vi "Gas Rack MAIN (PC).vi"() -> ()   [LabVIEW 2013]
uses:
  TypeDef/Controller Names.ctl
  TypeDef/StandConfigCluster.ctl
  TypeDef/DataCluster.ctl
  RT subVIs/Controls/TraceCluster.ctl
  TypeDef/Command Cluster.ctl
  TypeDef/TestCfgCluster.ctl
  TCP/PC/Event Mode.ctl
  TypeDef/Stability Cluster.ctl
  <vilib>/Utility/miscctls.llb/LVRowAndColumnTypeDef.ctl
  <vilib>/Utility/miscctls.llb/LVRowAndColumnUnsignedTypeDef.ctl
  TypeDef/Parameter Controls Mode.ctl
  TCP/PC/PCsend RTrecv CMD.ctl
  <vilib>/Utility/miscctls.llb/LVPositionTypeDef.ctl
  TypeDef/ConnSettingCluster.ctl
  <vilib>/Utility/config.llb/Write Key (String).vi
  <vilib>/Utility/file.llb/Write To Spreadsheet File (string).vi
  <vilib>/Utility/config.llb/NI_LVConfig.lvlib
panel:
  in  "Screen Control":enum32{"Page 1"}(tab)
  in  "pb.RunScreen":bool
  in  "pb.TestConfig":bool
  in  "pb.StandConfig":bool
  in  "Screen":T1(tab)=enum."Test Configuration Page"
  in  "FFTwindowMin":u16=300
  in  "FFTwindowMax":u16=1400 caption="Max"
  in  "Steps":u16(ring) items=["Manual", "1)   V=12, P=500, C=50", "2)   V=12, P=450, C=50", "3)   V=12, P=400, C=50"]
  out "Efficiency (%)":dbl format="%.1f"
  out "Controller CMD":dbl format="%#.1f"
  in  "Parameter 3":T2(ring)=enum."Command"
  in  "Setpoint3":dbl=10.0 caption="Setpoint 3" min=10.0 max=90.0 step=0.1
  out "Running?":bool
  in  "Serial Number":string
  out "Speed (RPM)":dbl format="%#.0f"
  out "PumpCurrent(Arms)":dbl caption="Pump Current\n(A RMS)" format="%.2f"
  out "CtrlrCurrent(A)":dbl caption="Controller\nCurrent (A)" format="%.2f"
  out "Fuel Temp (C)":dbl format="%.1f"
  out "Flow (L/H)":dbl format="%.1f"
  out "Pressure (kPa)":dbl format="%.1f"
  in  "Setpoint2":dbl caption="Setpoint 2" min=-1.0 max=800.0
  in  "Setpoint1":dbl caption="Setpoint 1" min=-1.0 max=18.0
  out "RS File Location":string caption="File Location"
  in  "pb.StartTest":bool
  out "Voltage (DC)":dbl caption="Controller\nVoltage (V)" format="%.2f"
  out "Stabilized?":bool
  in  "Tables":enum32{"Data", "Stats", "Notes"}(tab)
  in  "table.Data":string[][](table)
  in  "table.Stats":string[][](table)
  in  "Notes":string
  in  "Parameter 1":T3(ring)
  in  "Parameter 2":enum16{"Voltage", "Pressure", "Flow", "Speed"}(ring)=enum."Pressure"
  in  "Tab.Buttons":enum32{"Manual", "Test"}(tab)
  in  "pb.StartManual":bool
  in  "pb.GrabData":bool
  in  "pb.Pause Test":bool
  in  "pb.Skip Step":bool
  in  "pb.ClearProfile":bool
  in  "pb.load profile":bool
  in  "TestType":enum32{"Flow", "Test", "Hot\nFuel"}(radio)
  in  "File Location":string
  in  "Platform":string
  in  "Customer":string
  in  "Pump Control Style":T4
  in  "pb.load":bool
  in  "pb.save":bool
  in  "pb.new":bool
  in  "Pump Model":string
  in  "Durability Tank Number":string
  in  "Fuel Batch Number":string
  in  "Flow Test Fluid":string
  in  "Durability Fluid":string
  in  "Hours Completed":string
  in  "Shop Order Number":string
  in  "CA Number":string
  in  "Technician Name":string
  in  "Pump# Pages":enum32{"SN", "Auto"}(tab)
  in  "Serial Numbers":string[][](table)
  in  "pb.auto-pop":bool
  in  "pb.auto-confirm":bool
  in  "pb.auto-cancel":bool
  in  "Ending Serial Number":u32
  in  "Serial Number Step":u32
  in  "Starting Serial Number":u32
  in  "Parameters":string[][](table) caption="Parameter Setup"
  out "Hardware Style":string
  in  "Pressure Control":bool
  out "Max Command":dbl
  out "Min Command":dbl
  in  "Gauge Number":string
  out "Calibration Due Date":string
  in  "Speed Tolerance":dbl
  in  "Max Pressure":dbl
  in  "IP Address":string
  in  "Max Voltage":dbl
  in  "Free Flow Pressure":dbl
  in  "Free Flow Voltage":dbl
  in  "Init Free Flow (sec)":dbl
  in  "Max Current":dbl
  in  "Stable Count (sec)":dbl=1.0 min=1.0
  in  "Flow Tolerance":dbl
  in  "Voltage Tolerance":dbl
  in  "Pressure Tolerance":dbl
  in  "Parameter Timeout (sec)":dbl=3.0 min=6.0
  in  "Max Flow":dbl
  in  "Min Flow":dbl
  in  "pb.RetryRIO":bool
  in  "IP Address 2":string caption="IP Address"
  out "Tested Serial Numbers":string[][](table)
  out "Untested Serial Numbers":string[][](table)
  in  "pb.test cancel":bool
  in  "Next Serial Number":string
  in  "pb.select SN":bool
  out "InvalidResponses":string
  out "Error Out":errorcluster
  out "unreachable":bool
  in  "FlattenedData":string
  in  "Command":string
  in  "Connected?":bool
  in  "Connected? 2":bool
  in  "Panel Close?":bool
  out "StoredDataRow":i32
  in  "DataDisplayRefs":refnum<vi>[](array[refnum])
  # "Run Screen"
  # "Test Configuration Page"
  # "Stand Configuration Page"
  # "RIO Connection Page"
  # "Error occured with connection to RIO.\nCheck connections."
  # "Part Change Page"
  # "never implemented"
  # "Para 1 (0-4) [Voltage Pressure Flow Speed Deadhead]\nPara 2 (0-3) [Voltage Pressure Flow Speed]\nPara 3 (0-4) [Voltage Pressure Flow Speed Command]"
  # "New Features:"
  # "* Dynamically controls brushless pumps to meet parameters *"
  # "* Statistics include manually taken data points *"
  # "* Statistics updated with every data point taken *"
  # "* RPM is fully handled, no more user input for FFT windowing *"
  # "_______________________________________________________________________________________________________________________________________________________"
  # "* Calibration standardized *"
  # "* Voltage/current selectable at pump/controller *"
  # "_________________________________________________________________________________________________________________________________"
  # "* Added free flow on startup for brushless pumps *"
  # "Calibration due\nfor verification."
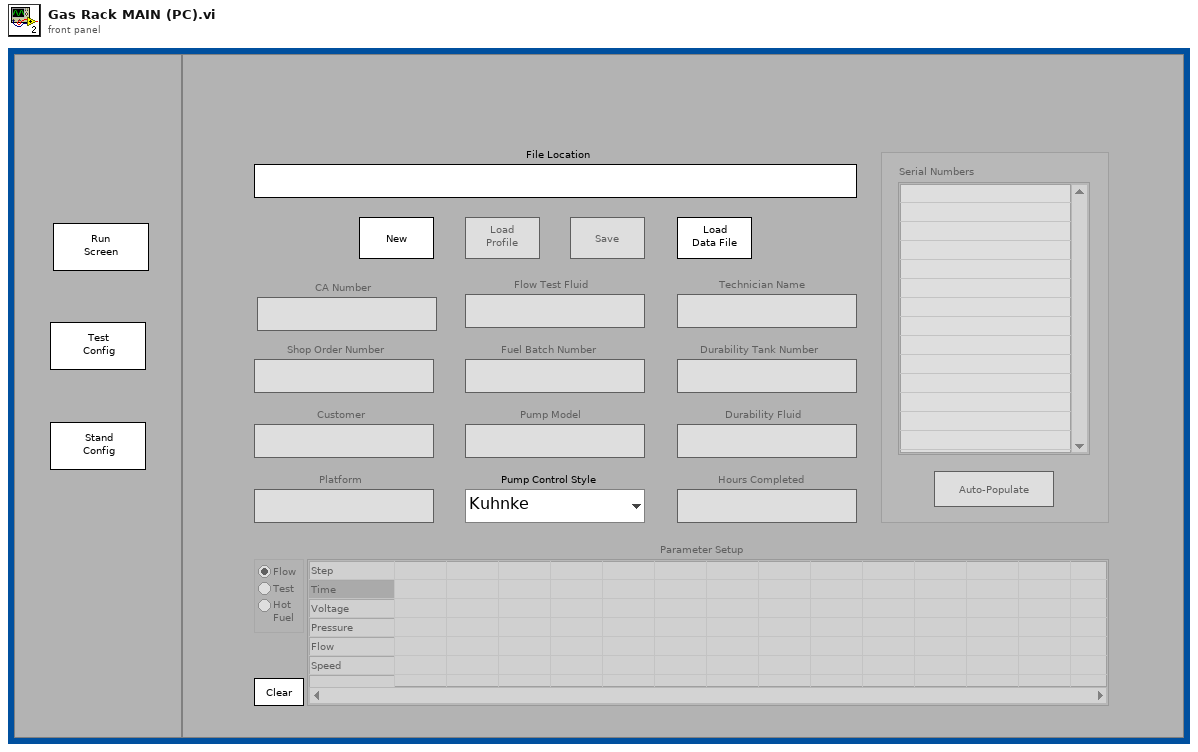
[diagram p1: front panel]
types:
  T1 = enum32{"Run Screen", "Test Configuration Page", "Stand Configuration Page", "RIO Connection", "Part Change", "Spare Front Panel Items", "Intro", "Cal Warning"}
  T2 = enum16{"Voltage", "Pressure", "Flow", "Speed", "Command"}
  T3 = enum16{"Voltage", "Pressure", "Flow", "Speed", "Deadhead"}
  T4 = typedef "Controller Names.ctl" = enum16{"Kuhnke", "McLaren", "Helbako BLDC", "Conti", "Hella E4LMF", "Hella E4LMD", "Hella E4DCG 20mm", "Hella E4DCG 30mm", "Helbako (old)", "TI PWM", "PSA", "Hella Hyundai Gas", "Hella Hyundai Diesel", "8 Comm", "10 Comm", "8 Comm Hella FCA", "10 Comm Hella FCA", "8 Comm Omron", "10 Comm Omron", "8 Comm Nissan", "10 Comm Nissan"}
  T5 = typedef "Stability Cluster.ctl" = cluster{"Voltage Tolerances":dbl, "Pressure Tolerances":dbl, "Flow Tolerances":dbl, "Speed Tolerances":dbl, "Stable Count (sec)":dbl}
  T6 = typedef "Command Cluster.ctl" = cluster{"Para1":i32, "SP1":dbl, "Para2":i32, "SP2":dbl, "Para3":i32, "SP3":dbl}
  T7 = cluster{"ParameterSet":string, "Data":string[][], "Step":i32, "EarliestDate":string, "Stats":string[][]}[]
  T8 = typedef "Event Mode.ctl" = enum16{"Init", "Get", "Set", "Destroy"}
  T9 = cluster{"Controller Name":T4, "CommSeg":i32, "PWM?":bool, "Frequency":i32, "Low Command":dbl, "High Command":dbl, "Stop Command":dbl, "Command Step":dbl, "Solenoid Stop?":bool, "Controller?":bool, "Name":string, "Indirect Nonzero CMD":dbl}[]
  T10 = cluster{"Controller Name":T4, "CommSeg":i32, "PWM?":bool, "Frequency":i32, "Low Command":dbl, "High Command":dbl, "Stop Command":dbl, "Command Step":dbl, "Solenoid Stop?":bool, "Controller?":bool, "Name":string, "Indirect Nonzero CMD":dbl}
  T11 = typedef "TestCfgCluster.ctl" = cluster{"Technician Name":string, "Shop Order Number":string, "Customer":string, "Platform":string, "Flow Test Fluid":string, "Fuel Batch #":string, "CA Number":string, "Durability Tank #":string, "Durability Fluid":string, "Hours Completed":string, "Pump Model":string, "Pump Control Style":T4}
  T12 = typedef "TraceCluster.ctl" = cluster{"PreTriggerPts":i32, "TotalPts":i32, "TriggerLvl":dbl, "PlotStyle":enum16{"Single - Rising Edge", "Single - Falling Edge", "Continuous", "Repeat - Rising Edge", "Repeat - Falling Edge"}, "TriggerChannel":i32, "TraceCtrl":bool}
  T13 = typedef "DataCluster.ctl" = cluster{"Pump Voltage (V)":dbl, "Pump Current (Arms)":dbl, "Pressure (kPA)":dbl, "Flow (L/H)":dbl, "Controller Voltage (V)":dbl, "Controller Current (A)":dbl, "Fuel Temp (C)":dbl, "Speed (RPM)":dbl, "Efficiency (%)":dbl, "Stabilized?":bool, "Controller CMD":dbl}
  T14 = typedef "StandConfigCluster.ctl" = cluster{"Max Voltage":dbl, "Voltage Tolerance":dbl, "Max Current":dbl, "Max Pressure":dbl, "Pressure Tolerance":dbl, "Min Flow":dbl, "Max Flow":dbl, "Flow Tolerance":dbl, "Speed Tolerance":dbl, "Stable Count":dbl, "Parameter Timeout":dbl, "Init Free Flow":dbl, "Free Flow Voltage":dbl, "Free Flow Pressure":dbl}
  T15 = cluster{"TestCfgCluster":T11, "Serial Numbers":string[], "StandConfigCluster":T14, "Serial Number":string, "table.Data":string[][], "table.Stats":string[][], "CommandCluster":T6, "DataCluster":T13, "RIOTries":i32, "TestRunning?":bool, "StepIndex":i32, "CurrentDataFile":path, "DefaultDataPath":path, "PreviousDataFile":path, "Untested SNs":string[], "Tested SNs":string[], "RIOconnection":bool, "StepTimeLimit":dbl, "WaitingData":bool, "Controller":cluster{"Controller Name":T4, "CommSeg":i32, "PWM?":bool, "Frequency":i32, "Low Command":dbl, "High Command":dbl, "Stop Command":dbl, "Command Step":dbl, "Solenoid Stop?":bool, "Controller?":bool, "Name":string, "Indirect Nonzero CMD":dbl}, "TraceCluster":T12, "IP Address":string, "TemplatePath":path, "Notes":string, "LastDataSet":string[], "ValidFile?":bool, "LastDataRow":i32, "LastStatRow":i32, "Gauge Number":string, "Calibration Due Date":string, "Free Flow":bool, "StepDataActive":dbl, "Parameters":string[][], "KF.Parameters":bool, "Flow?":bool, "ColInsert":bool, "SkipStep":bool, "KeepManualPts":bool, "Created/ModFiles":cluster{"FilePath":path, "Save?":bool}[], "Controller List":cluster{"Controller Name":T4, "CommSeg":i32, "PWM?":bool, "Frequency":i32, "Low Command":dbl, "High Command":dbl, "Stop Command":dbl, "Command Step":dbl, "Solenoid Stop?":bool, "Controller?":bool, "Name":string, "Indirect Nonzero CMD":dbl}[], "ProfilePath":path, "LastFileState":enum16{"New File", "Load File", "Neither"}, "NotLoadProfile":bool, "LastDataTime":i64, "ValidPara?":bool, "StatBundle":cluster{"ParameterSet":string, "Data":string[][], "Step":i32, "EarliestDate":string, "Stats":string[][]}[], "DesiredParameters":T6, "Stability Cluster":T5, "DataDisplayRefs":refnum<vi>[], "ExpectedFPGA":i32}
  T16 = typedef "LVRowAndColumnUnsignedTypeDef.ctl" = cluster{"Row":u32, "Column":u32}
  T17 = enum8{"Enabled", "Disabled", "Disabled and Grayed Out"}
  T18 = typedef "Parameter Controls Mode.ctl" = enum16{"Init", "Update Ranges", "Set Controls"}
  T19 = typedef "LVRowAndColumnTypeDef.ctl" = cluster{"Row":i32, "Column":i32}
  T20 = enum32{"invalid app kind", "Development System", "Run Time System", "Student Edition", "Embedded LabVIEW", "Evaluation", "Custom"}
  T21 = enum16{"Init", "Run Screen", "Test Config", "Stand Config", "Lock All", "Other Tab"}
  T22 = cluster{"Command":string, "FlattenedData":string}
  T23 = typedef "PCsend RTrecv CMD.ctl" = enum16{"ConnSettings", "Connect", "CMD", "Controller", "PSenable", "ReqCalDate", "Tolerances", "Stable Trigger", "Stop", "VPLimits", "NeedleValve", "SpeedWindow", "FreezeCmdPID", "LoadFPGA"}
  T24 = cluster{"CurrentDataFile":path, "StandConfigCluster":T14, "IP Address":string, "DefaultDataPath":path, "Gauge Number":string, "ExpectedFPGA":i32}
  T25 = typedef "RTsend PCrecv CMD.ctl" = enum16{"Data", "Connected?", "CalFileDate"}
  T26 = enum16{"Voltage", "Pressure", "Flow", "Speed", "Deadhead"}[]
  T27 = typedef "NI_LVConfig.lvlib/Config Data RefNum.ctl" = refnum<k1>
  T28 = typedef "eventvkey.ctl" = enum16{"ASCII", "Enter", "Return", "Shift", "Ctrl", "Alt", "Cmd", "Opt", "Caps", "NumLock", "Clear", "Break", "Up", "Down", "Left", "Right", "Insert", "Delete", "Home", "End", "PageUp", "PageDown", "Escape", "Help", "Pause", "ScrollLock", "F1", "F2", "F3", "F4", "F5", "F6", "F7", "F8", "F9", "F10", "F11", "F12", "F13", "F14", "F15", "F16", "F17", "F18", "F19", "F20", "F21", "F22", "F23", "F24", "Play", "VolumeUp", "VolumeDown", "Mute", "Two Byte Char"}
  T29 = enum16{"Left Button", "Center Button", "Right Button", "Window Close"}
  T30 = typedef "LVPositionTypeDef.ctl" = cluster{"Left":i32, "Top":i32}
  T31 = cluster{"CommandCluster":T6, "DesiredParameters":T6}
  T32 = cluster{"data string":string, "data string":string}
  T33 = typedef "ConnSettingCluster.ctl" = cluster{"ConnectAttemptLimit(5)":u32, "IP Address":string, "Send Port":u16, "Recv Port":u16}
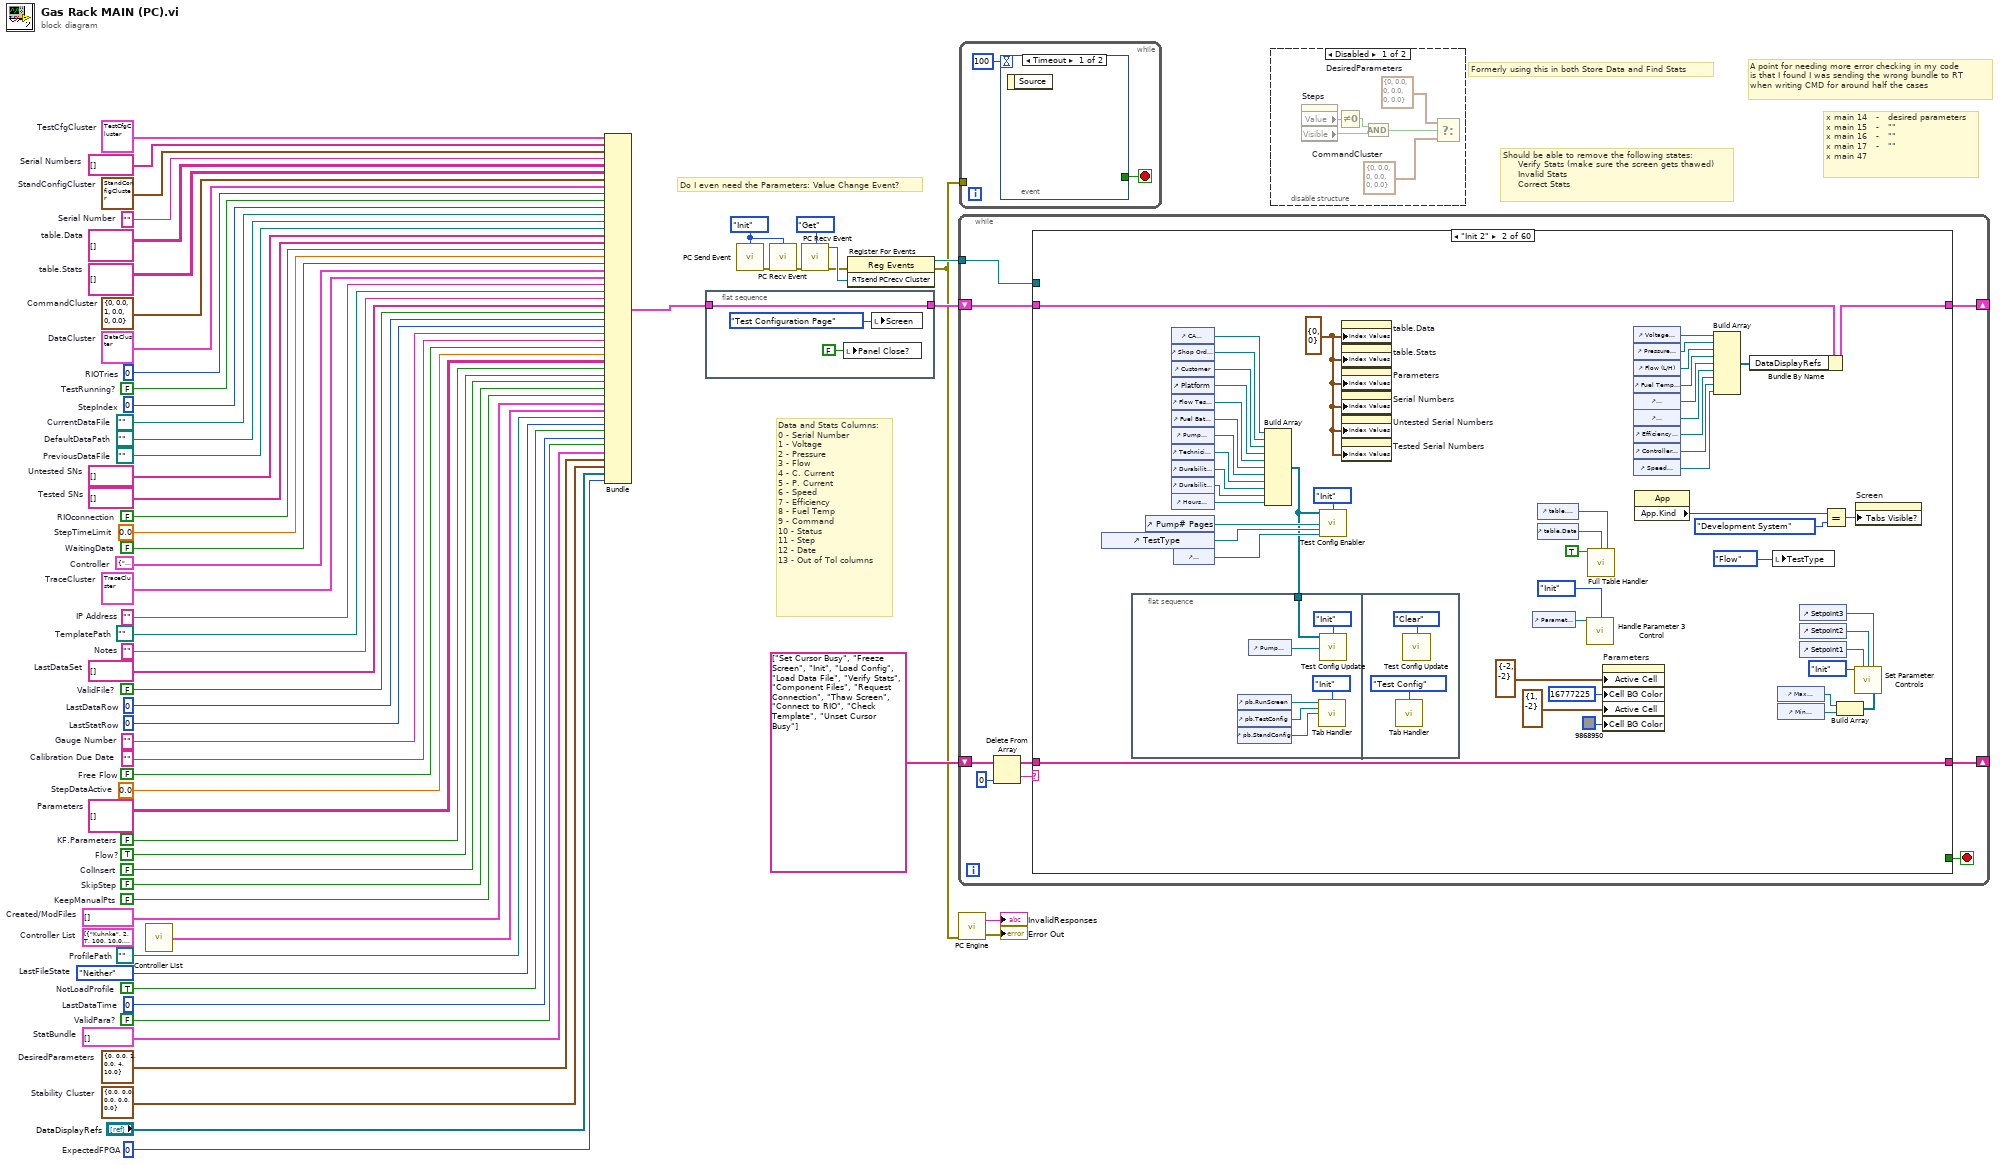
[diagram p0: block diagram]
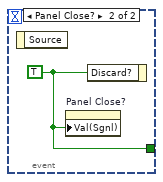
[diagram p3: hidden frame]
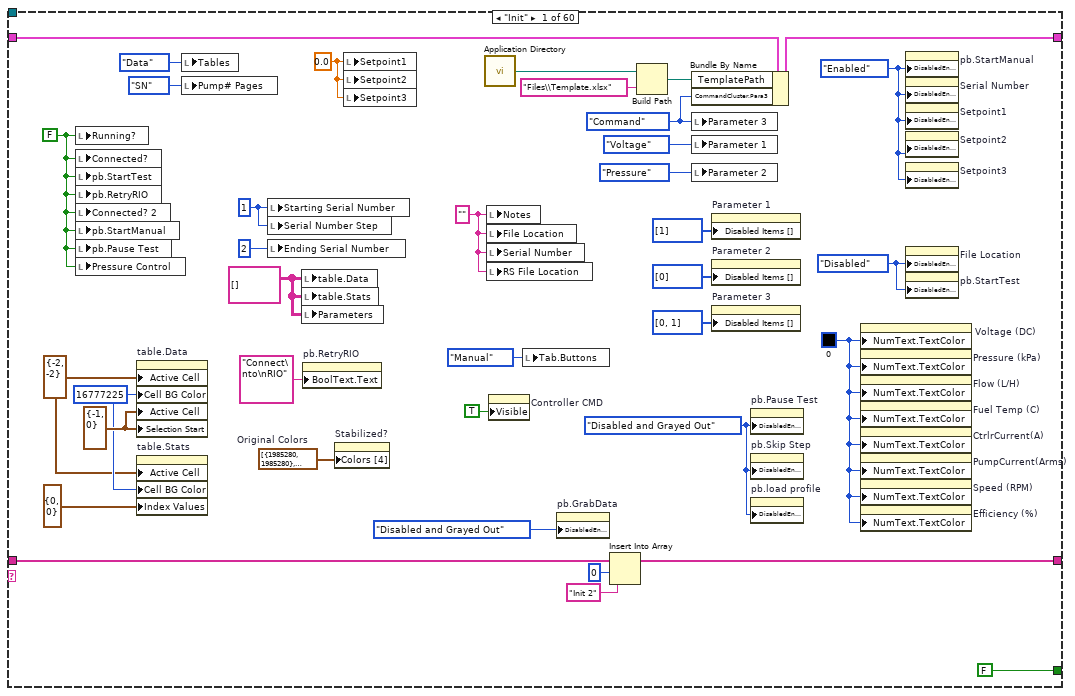
[diagram p4: hidden frame]
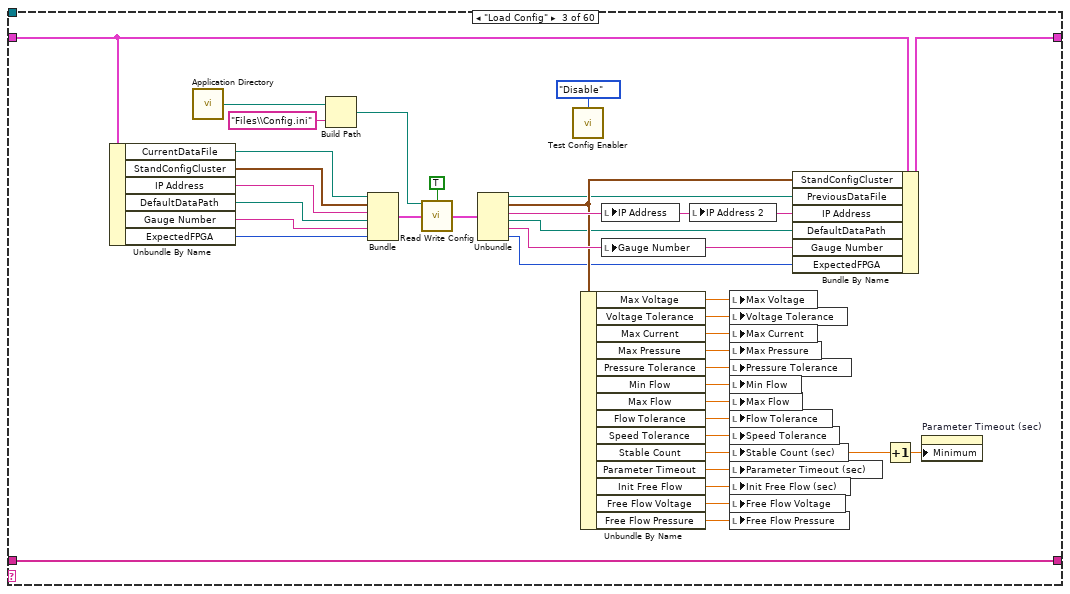
[diagram p5: hidden frame]
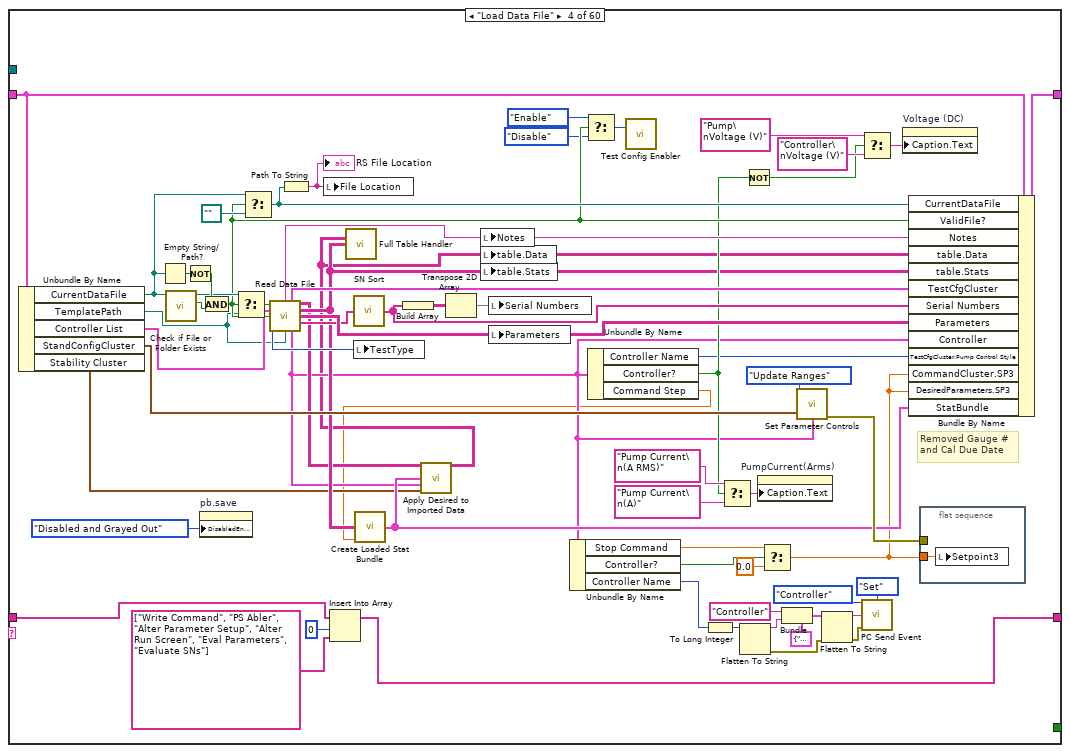
[diagram p6: hidden frame]
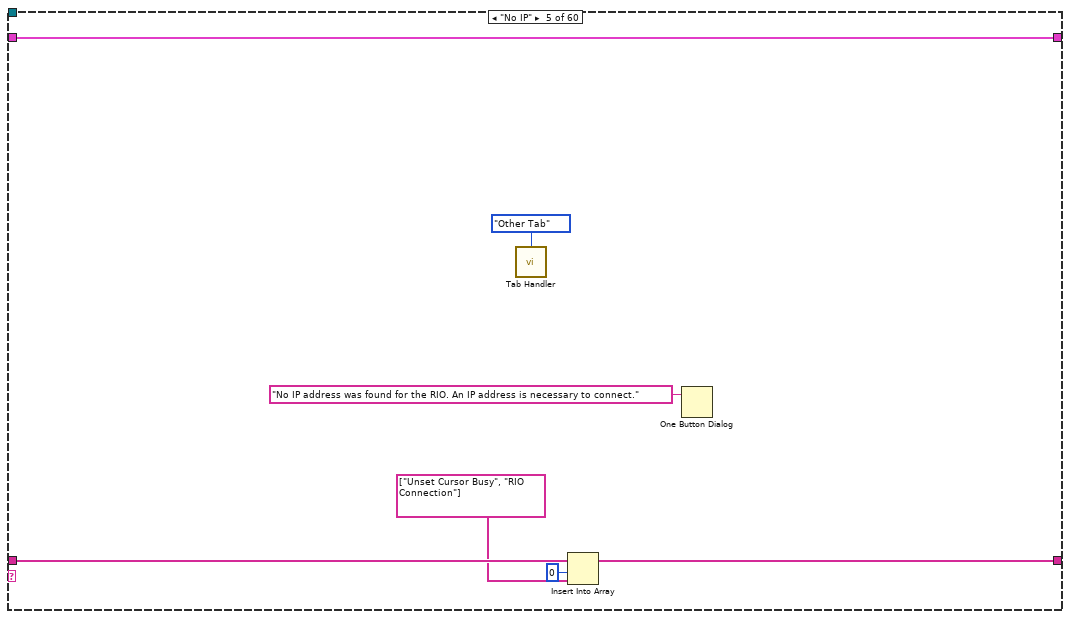
[diagram p7: hidden frame]
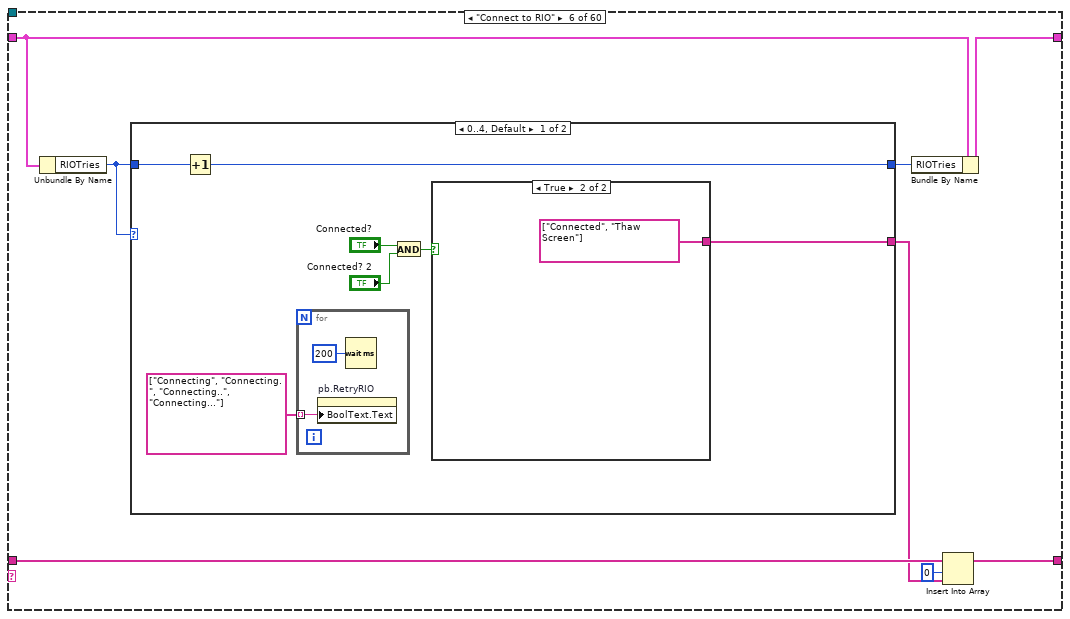
[diagram p8: hidden frame]
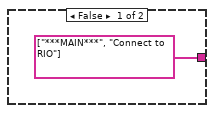
[diagram p9: hidden frame]
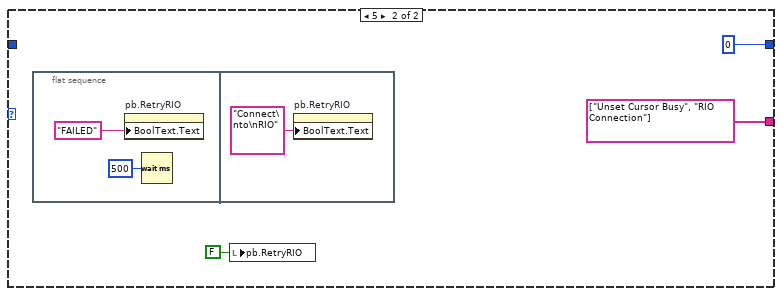
[diagram p10: hidden frame]
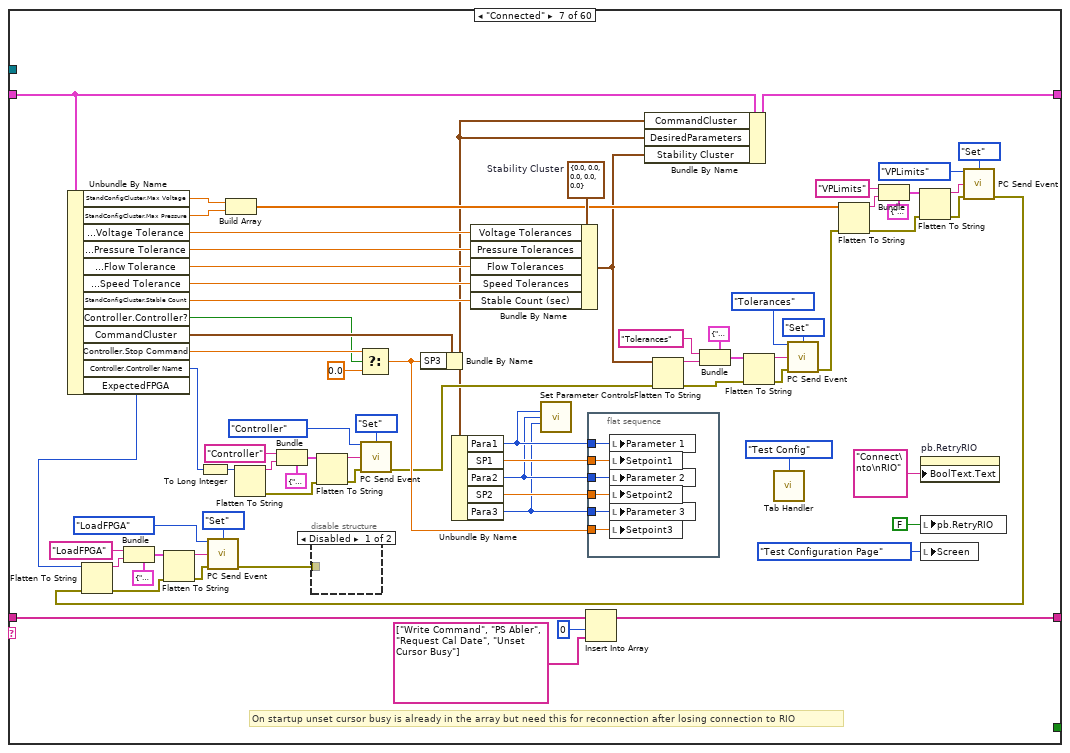
[diagram p11: hidden frame]
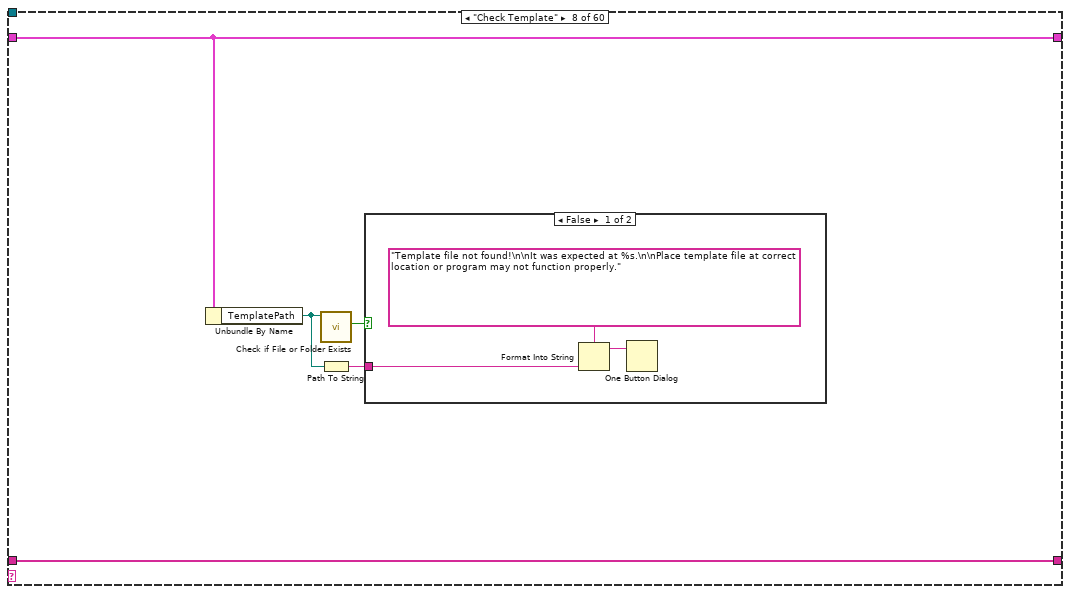
[diagram p13: hidden frame]
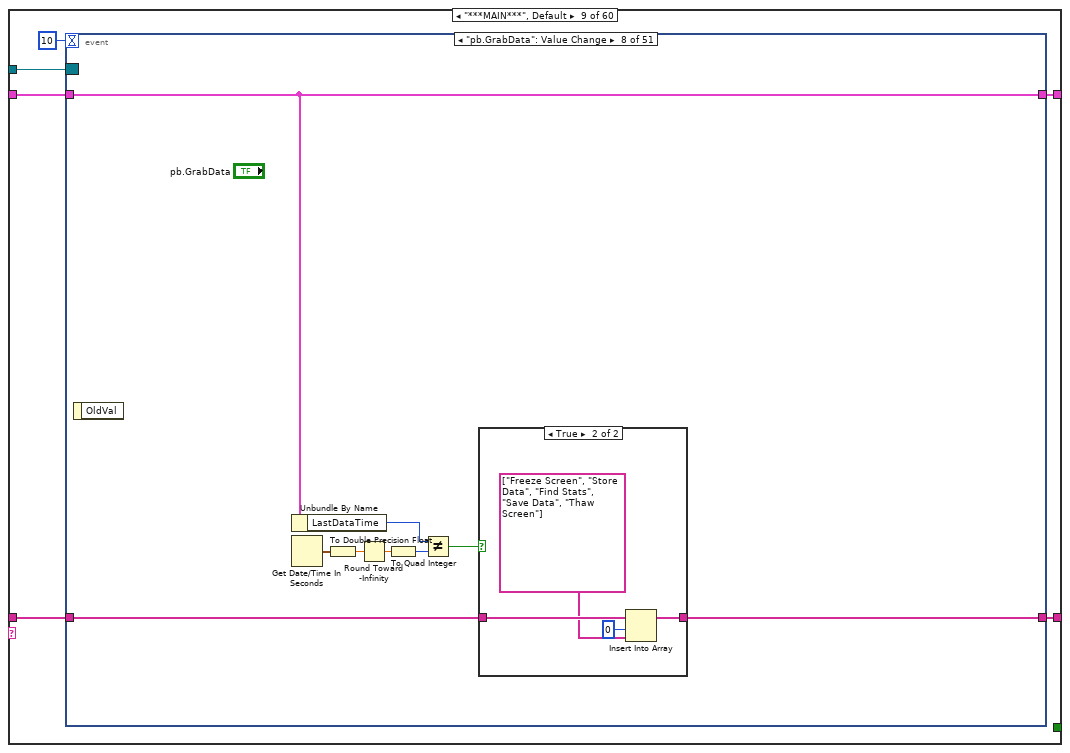
[diagram p15: hidden frame]
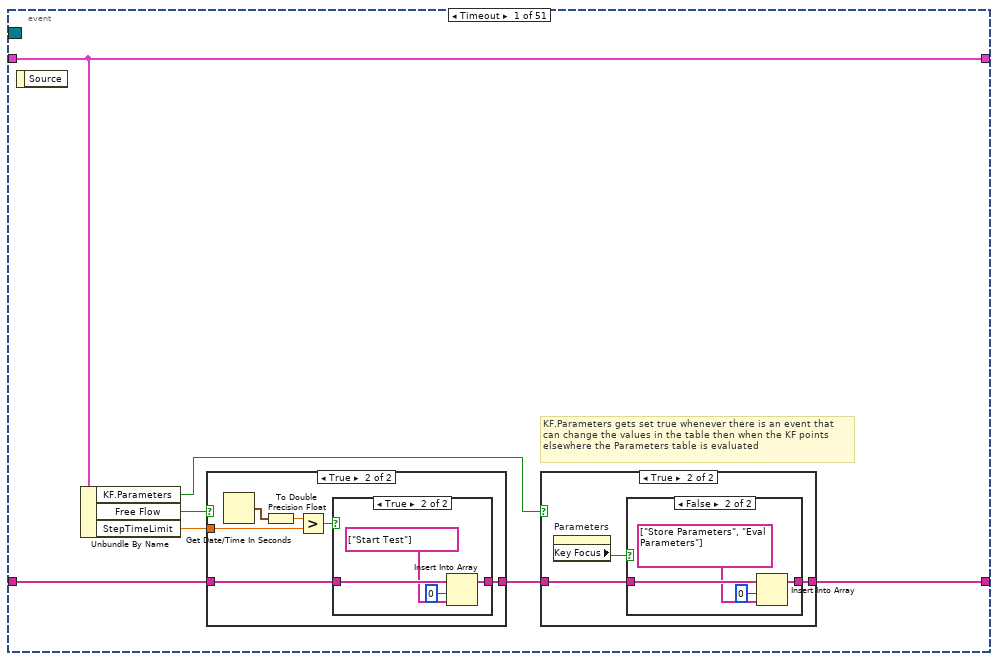
[diagram p16: hidden frame]
diagram:
  w1 = 0  # ExpectedFPGA
  w3 = T5 {"Voltage Tolerances"=0.0, "Pressure Tolerances"=0.0, "Flow Tolerances"=0.0, "Speed Tolerances"=0.0, "Stable Count (sec)"=0.0}  # Stability Cluster
  w4 = T6 {"Para1"=0, "SP1"=0.0, "Para2"=1, "SP2"=0.0, "Para3"=4, "SP3"=10.0}  # DesiredParameters
  w5 = T7 []  # StatBundle
  w6 = FALSE  # ValidPara?
  w7 = i64 0  # LastDataTime
  w15 = Event_Mode."Init" ("Mode")
  w21 = TRUE  # NotLoadProfile
  w22 = enum16{"New File", "Load File", "Neither"}."Neither"  # LastFileState
  w24 = path ""  # ProfilePath
  (unwired) T9 [{"Controller Name"=enum."Kuhnke", "CommSeg"=2, "PWM?"=TRUE, "Frequency"=100, "Low Command"=10.0, "High Command"=90.0, "Stop Command"=10.0, "Command Step"=0.1, "Solenoid Stop?"=FALSE, "Controller?"=TRUE, "Name"="Kuhnke", "Indirect Nonzero CMD"=15.0}, {"Controller Name"=enum."Helbako BLDC", "CommSeg"=2, "PWM?"=TRUE, "Frequency"=100, "Low Command"=10.0, "High Command"=90.0, "Stop Command"=10.0, "Command Step"=0.1, "Solenoid Stop?"=FALSE, "Controller?"=TRUE, "Name"="Helbako BLDC", "Indirect Nonzero CMD"=15.0}, {"Controller Name"=enum."Conti", "CommSeg"=2, "PWM?"=FALSE, "Frequency"=100, "Low Command"=0.0, "High Command"=800.0, "Stop Command"=0.0, "Command Step"=1.0, "Solenoid Stop?"=FALSE, "Controller?"=TRUE, "Name"="Conti", "Indirect Nonzero CMD"=0.0}, {"Controller Name"=enum."Hella E4LMF", "CommSeg"=2, "PWM?"=FALSE, "Frequency"=100, "Low Command"=0.0, "High Command"=100.0, "Stop Command"=0.0, "Command Step"=1.0, "Solenoid Stop?"=FALSE, "Controller?"=TRUE, "Name"="Hella BLDC Screw", "Indirect Nonzero CMD"=10.0}, {"Controller Name"=enum."Helbako (old)", "CommSeg"=2, "PWM?"=FALSE, "Frequency"=100, "Low Command"=0.0, "High Command"=100.0, "Stop Command"=0.0, "Command Step"=1.0, "Solenoid Stop?"=FALSE, "Controller?"=TRUE, "Name"="Hella BLDC Turbine", "Indirect Nonzero CMD"=10.0}, {"Controller Name"=enum."Helbako (old)", "CommSeg"=2, "PWM?"=FALSE, "Frequency"=100, "Low Command"=0.0, "High Command"=100.0, "Stop Command"=0.0, "Command Step"=0.1, "Solenoid Stop?"=FALSE, "Controller?"=TRUE, "Name"="Helbako (old)", "Indirect Nonzero CMD"=0.0}, {"Controller Name"=enum."TI PWM", "CommSeg"=2, "PWM?"=TRUE, "Frequency"=100, "Low Command"=0.0, "High Command"=100.0, "Stop Command"=0.0, "Command Step"=0.1, "Solenoid Stop?"=FALSE, "Controller?"=TRUE, "Name"="TI PWM", "Indirect Nonzero CMD"=0.0}, {"Controller Name"=enum."PSA", "CommSeg"=2, "PWM?"=TRUE, "Frequency"=100, "Low Command"=5.0, "High Command"=95.0, "Stop Command"=5.0, "Command Step"=0.1, "Solenoid Stop?"=FALSE, "Controller?"=TRUE, "Name"="PSA", "Indirect Nonzero CMD"=5.0}, {"Controller Name"=enum."Hella Hyundai Diesel", "CommSeg"=2, "PWM?"=FALSE, "Frequency"=100, "Low Command"=0.0, "High Command"=800.0, "Stop Command"=0.0, "Command Step"=1.0, "Solenoid Stop?"=TRUE, "Controller?"=TRUE, "Name"="Hella Gas", "Indirect Nonzero CMD"=0.0}, {"Controller Name"=enum."8 Comm", "CommSeg"=10, "PWM?"=FALSE, "Frequency"=100, "Low Command"=370.0, "High Command"=461.0, "Stop Command"=370.0, "Command Step"=1.0, "Solenoid Stop?"=TRUE, "Controller?"=TRUE, "Name"="Hella Diesel", "Indirect Nonzero CMD"=370.0}, {"Controller Name"=enum."8 Comm", "CommSeg"=8, "PWM?"=FALSE, "Frequency"=150, "Low Command"=0.0, "High Command"=1.0, "Stop Command"=0.0, "Command Step"=1.0, "Solenoid Stop?"=FALSE, "Controller?"=FALSE, "Name"="8 Comm", "Indirect Nonzero CMD"=0.0}, {"Controller Name"=enum."10 Comm", "CommSeg"=10, "PWM?"=FALSE, "Frequency"=150, "Low Command"=0.0, "High Command"=1.0, "Stop Command"=0.0, "Command Step"=1.0, "Solenoid Stop?"=FALSE, "Controller?"=FALSE, "Name"="10 Comm", "Indirect Nonzero CMD"=0.0}, {"Controller Name"=enum."10 Comm Hella FCA", "CommSeg"=8, "PWM?"=TRUE, "Frequency"=150, "Low Command"=0.0, "High Command"=50.0, "Stop Command"=80.0, "Command Step"=0.1, "Solenoid Stop?"=FALSE, "Controller?"=TRUE, "Name"="8 Comm Hella", "Indirect Nonzero CMD"=0.0}, {"Controller Name"=enum."8 Comm Omron", "CommSeg"=10, "PWM?"=TRUE, "Frequency"=150, "Low Command"=0.0, "High Command"=50.0, "Stop Command"=80.0, "Command Step"=0.1, "Solenoid Stop?"=FALSE, "Controller?"=TRUE, "Name"="10 Comm Hella", "Indirect Nonzero CMD"=0.0}, {"Controller Name"=enum."8 Comm Omron", "CommSeg"=8, "PWM?"=TRUE, "Frequency"=150, "Low Command"=5.0, "High Command"=50.0, "Stop Command"=75.0, "Command Step"=0.1, "Solenoid Stop?"=FALSE, "Controller?"=TRUE, "Name"="8 Comm Omron", "Indirect Nonzero CMD"=5.0}, {"Controller Name"=enum."10 Comm Omron", "CommSeg"=10, "PWM?"=TRUE, "Frequency"=150, "Low Command"=5.0, "High Command"=50.0, "Stop Command"=75.0, "Command Step"=0.1, "Solenoid Stop?"=FALSE, "Controller?"=TRUE, "Name"="10 Comm Omron", "Indirect Nonzero CMD"=5.0}, {"Controller Name"=enum."8 Comm Nissan", "CommSeg"=8, "PWM?"=TRUE, "Frequency"=10, "Low Command"=50.0, "High Command"=90.0, "Stop Command"=50.0, "Command Step"=0.1, "Solenoid Stop?"=TRUE, "Controller?"=TRUE, "Name"="8 Comm Nissan", "Indirect Nonzero CMD"=50.0}, {"Controller Name"=enum."10 Comm Nissan", "CommSeg"=10, "PWM?"=TRUE, "Frequency"=10, "Low Command"=50.0, "High Command"=90.0, "Stop Command"=50.0, "Command Step"=0.1, "Solenoid Stop?"=TRUE, "Controller?"=TRUE, "Name"="10 Comm Nissan", "Indirect Nonzero CMD"=50.0}]  # Controller List
  w25 = T10 {"Controller Name"=enum."Kuhnke", "CommSeg"=2, "PWM?"=TRUE, "Frequency"=100, "Low Command"=10.0, "High Command"=90.0, "Stop Command"=10.0, "Command Step"=0.1, "Solenoid Stop?"=FALSE, "Controller?"=TRUE, "Name"="Kuhnke", "Indirect Nonzero CMD"=15.0}  # Controller
  w50 = T11 {"Technician Name"="", "Shop Order Number"="", "Customer"="", "Platform"="", "Flow Test Fluid"="", "Fuel Batch #"="", "CA Number"="", "Durability Tank #"="", "Durability Fluid"="", "Hours Completed"="", "Pump Model"="", "Pump Control Style"=enum."Kuhnke"}  # TestCfgCluster
  w41 = T6 {"Para1"=0, "SP1"=0.0, "Para2"=1, "SP2"=0.0, "Para3"=0, "SP3"=0.0}  # CommandCluster
  w52 = T12 {"PreTriggerPts"=0, "TotalPts"=10, "TriggerLvl"=0.0, "PlotStyle"=enum."Single - Falling Edge", "TriggerChannel"=2, "TraceCtrl"=FALSE}  # TraceCluster
  w26 = cluster{"FilePath":path, "Save?":bool}[] []  # Created/ModFiles
  w27 = string[][] []  # table.Stats
  w28 = string[][] []  # table.Data
  w29 = FALSE  # KeepManualPts
  w30 = FALSE  # SkipStep
  w31 = FALSE  # ColInsert
  w32 = TRUE  # Flow?
  w33 = FALSE  # KF.Parameters
  w34 = string[][] []  # Parameters
  w35 = 0.0  # StepDataActive
  w36 = FALSE  # Free Flow
  w37 = ""  # Calibration Due Date
  w38 = ""  # Gauge Number
  w39 = path ""  # PreviousDataFile
  w40 = string[] []  # Tested SNs
  w42 = 0  # LastStatRow
  w43 = 0  # LastDataRow
  w44 = string[] []  # Serial Numbers
  w45 = ""  # Serial Number
  w46 = FALSE  # ValidFile?
  w47 = string[] []  # LastDataSet
  w48 = ""  # Notes
  w49 = path ""  # TemplatePath
  w51 = ""  # IP Address
  w53 = FALSE  # WaitingData
  w54 = 0.0  # StepTimeLimit
  w55 = T13 {"Pump Voltage (V)"=0.0, "Pump Current (Arms)"=0.0, "Pressure (kPA)"=0.0, "Flow (L/H)"=0.0, "Controller Voltage (V)"=0.0, "Controller Current (A)"=0.0, "Fuel Temp (C)"=0.0, "Speed (RPM)"=0.0, "Efficiency (%)"=0.0, "Stabilized?"=FALSE, "Controller CMD"=0.0}  # DataCluster
  w61 = string[] []  # Untested SNs
  w60 = path ""  # DefaultDataPath
  w59 = path ""  # CurrentDataFile
  w62 = T14 {"Max Voltage"=0.0, "Voltage Tolerance"=0.0, "Max Current"=0.0, "Max Pressure"=0.0, "Pressure Tolerance"=0.0, "Min Flow"=0.0, "Max Flow"=0.0, "Flow Tolerance"=0.0, "Speed Tolerance"=0.0, "Stable Count"=0.0, "Parameter Timeout"=0.0, "Init Free Flow"=0.0, "Free Flow Voltage"=0.0, "Free Flow Pressure"=0.0}  # StandConfigCluster
  w58 = 0  # StepIndex
  w57 = FALSE  # TestRunning?
  w56 = 0  # RIOTries
  w63 = FALSE  # RIOconnection
  # "x main 14   -   desired parameters\nx main 15   -   \"\"\nx main 16   -   \"\"\nx main 17   -   \"\"\nx main 47"
  # "Formerly using this in both Store Data and Find Stats"
  # "A point for needing more error checking in my code\nis that I found I was sending the wrong bundle to RT\nwhen writing CMD for around half the cases"
  # "Should be able to remove the following states:\n     Verify Stats (make sure the screen gets thawed)\n     Invalid Stats\n     Correct Stats"
  # "Data and Stats Columns:\n0 - Serial Number\n1 - Voltage\n2 - Pressure\n3 - Flow\n4 - C. Current\n5 - P. Current\n6 - Speed\n7 - Efficiency\n8 - Fuel Temp\n9 - Command\n10 - Status\n11 - Step\n12 - Date\n13 - Out of Tol columns"
  # "Do I even need the Parameters: Value Change Event?"
  n1 = call "Controller List.vi"() -> ("Controller List"=w23:T9)  [unwired: 5 in]
  n2 = Bundle("TestCfgCluster"=w50, "Serial Numbers"=w44, "StandConfigCluster"=w62, "Serial Number"=w45, "table.Data"=w28, "table.Stats"=w27, "CommandCluster"=w41, "DataCluster"=w55, "RIOTries"=w56, "TestRunning?"=w57, "StepIndex"=w58, "CurrentDataFile"=w59, "DefaultDataPath"=w60, "PreviousDataFile"=w39, "Untested SNs"=w61, "Tested SNs"=w40, "RIOconnection"=w63, "StepTimeLimit"=w54, "WaitingData"=w53, "Controller"=w25, "TraceCluster"=w52, "IP Address"=w51, "TemplatePath"=w49, "Notes"=w48, "LastDataSet"=w47, "ValidFile?"=w46, "LastDataRow"=w43, "LastStatRow"=w42, "Gauge Number"=w38, "Calibration Due Date"=w37, "Free Flow"=w36, "StepDataActive"=w35, "Parameters"=w34, "KF.Parameters"=w33, "Flow?"=w32, "ColInsert"=w31, "SkipStep"=w30, "KeepManualPts"=w29, "Created/ModFiles"=w26, "Controller List"=w23, "ProfilePath"=w24, "LastFileState"=w22, "NotLoadProfile"=w21, "LastDataTime"=w7, "ValidPara?"=w6, "StatBundle"=w5, "DesiredParameters"=w4, "Stability Cluster"=w3, "DataDisplayRefs"="DataDisplayRefs", "ExpectedFPGA"=w1) -> (w20:T15)  [unwired: 1 in]
  n3 = flat-sequence {
    tunnel: w20 -> [w66]
    tunnel: [w66] -> w10
    frame #0 {
      n4 = local write "Panel Close?"(FALSE ("Panel Close?")) -> ()
      n5 = local write "Screen"(T1."Test Configuration Page" ("Screen")) -> ()
    }
  }
  n6 = call "PC Send Event.vi"("Mode"=w15) -> ("Error Out"=w14:errorcluster)  [unwired: 13 in, 1 out]
  n7 = call "PC Recv Event.vi"("Mode"=w15, "Error In"=w14) -> ("Error Out"=w17:errorcluster)  [unwired: 12 in, 1 out]
  n8 = call "PC Recv Event.vi"("Mode"=Event_Mode."Get", "Error In"=w17) -> ("RTsend PCrecv Cluster"=w16:refnum<user-event>, "Error Out"=w13:errorcluster)  [unwired: 12 in]
  n9 = register-events(error in=w13, w16) -> (reference out=w19:refnum<event-registration>, error out=w8:errorcluster)  [unwired: 1 in]
  n10 = while {
    shift-right: [w72] -> _
    shift-left: string[] ["Set Cursor Busy", "Freeze Screen", "Init", "Load Config", "Load Data File", "Verify Stats", "Component Files", "Request Connection", "Thaw Screen", "Connect to RIO", "Check Template", "Unset Cursor Busy"] -> [w75]
    shift-right: [w67] -> _
    shift-left: w10 -> [w71]
    tunnel: w19 -> [w69]
    stop <- w70 stop-if-true
    n11 = Delete From Array(array=w75, index=0) -> (deleted portion=w68:string, array with subset deleted=w73:string[])  [unwired: 1 in]
    n12 = case shown="\"Init 2\"" w68 {
      selector: w68 -> [_ _ _ _ _ _ _ _ _ _ _ _ _ _ _ _ _ _ _ _ _ _ _ _ _ _ _ _ _ _ _ _ _ _ _ _ _ _ _ _ _ _ _ _ _ _ _ _ w2683 _ _ _ _ _ _ _ _ _ _ _]
      tunnel: w73 -> [w86 w162 w208 w211 w279 w286 w368 w390 w396 w1389 w1412 w1442 w1522 w1574 w1640 w1680 w1702 w1746 w1786 w1895 w1940 w1982 w2030 w2036 w2073 w2098 w2117 w2141 w2186 w2207 w2220 w2247 w2276 w2299 w2351 w2356 w2385 w2421 w2424 w2454 w2485 w2533 w2564 w2586 w2619 w2627 w2645 w2662 w2691 w2734 w2770 w2792 w2794 w2861 w2863 w2865 w2875 w2950 w2955 w2958]
      tunnel: [w85 w162 w208 w210 w276 w283 w367 w390 w394 w1388 w1411 w1441 w1521 w1573 w1639 w1680 w1702 w1746 w1785 w1895 w1939 w1982 w2030 w2035 w2070 w2098 w2117 w2140 w2186 w2207 w2219 w2246 w2275 w2298 w2351 w2355 w2384 w2421 w2423 w2454 w2484 w2533 w2563 w2585 w2619 w2627 w2645 w2661 w2697 w2734 w2770 w2792 w2793 w2861 w2863 w2865 w2875 w2948 w2955 w2958] -> w72
      tunnel: w71 -> [w99 w125 w204 w272 w280 w288 w374 w389 w398 w1391 w1414 w1440 w1520 w1570 w1645 w1674 w1699 w1743 w1787 w1894 w1947 w1989 w2013 w2038 w2082 w2096 w2137 w2144 w2177 w2204 w2235 w2253 w2296 w2302 w2344 w2382 w2394 w2420 w2445 w2455 w2483 w2535 w2562 w2584 w2605 w2622 w2646 w2663 w2699 w2735 w2771 w2785 w2796 w2862 w2864 w2866 w2874 w2944 w2956 w2959]
      tunnel: [FALSE _ _ _ _ _ _ _ _ _ _ _ _ _ _ _ _ _ _ _ _ _ _ _ _ _ _ _ _ _ _ _ _ _ _ _ _ _ _ _ _ _ _ _ _ _ _ _ _ _ _ _ _ _ _ _ _ _ TRUE _] -> w70
      tunnel: w69 -> [_ _ _ _ _ _ _ _ w399 _ _ _ _ _ _ _ _ _ _ _ _ _ _ _ _ _ _ _ _ _ _ _ _ _ _ _ _ _ _ _ _ _ _ _ _ _ _ _ _ _ _ _ _ _ _ _ _ _ _ _]
      tunnel: [w98 w124 w203 w271 w280 w287 w377 w389 w397 w1390 w1413 w1443 w1523 w1569 w1644 w1674 w1701 w1743 w1787 w1893 w1956 w1998 w2012 w2038 w2081 w2097 w2136 w2145 w2176 w2204 w2241 w2254 w2295 w2301 w2345 w2381 w2393 w2419 w2447 w2455 w2482 w2534 w2561 w2583 w2604 w2620 w2646 w2663 w2694 w2735 w2771 w2784 w2795 w2862 w2864 w2866 w2874 w2946 w2956 w2959] -> w67
      frame "Init" {
        w76 = T17."Disabled and Grayed Out" ("Disabled")
        w97 = T2."Command" ("Parameter 3.1")
        w101 = cluster{u32, u32}[] [{1985280, 1985280}, {6618880, 6618880}, {1985280, 1985280}, {6618880, 6618880}]  # Original Colors
        w95 = T19 {"Row"=-1, "Column"=0} ("Active Cell:Active Cell")
        w92 = T19 {"Row"=-2, "Column"=-2} ("Active Cell:Active Cell")
        w93 = u32 16777225 ("Active Cell:Cell Background Color")
        w103 = 0.0 ("Setpoint1")
        w105 = u32 1 ("Starting Serial Number")
        w87 = string[][] [] ("Brushless Parameters")
        w89 = "" ("Technician Name")
        w79 = u32 0
        w81 = T17."Disabled" ("Disabled")
        w78 = FALSE
        w96 = T17."Enabled" ("Disabled")
        n13 = local write "Running?"(w78) -> ()
        n14 = local write "Connected?"(w78) -> ()
        n15 = local write "pb.StartTest"(w78) -> ()
        n16 = local write "pb.RetryRIO"(w78) -> ()
        n17 = local write "Connected? 2"(w78) -> ()
        n18 = local write "pb.StartManual"(w78) -> ()
        n19 = local write "pb.Pause Test"(w78) -> ()
        n20 = local write "Pressure Control"(w78) -> ()
        n21 = property on="table.Data" class="Tbl (strict)"("Active Cell"=w92, "Cell BG Color"=w93, "Active Cell"=w95, "Selection Start"=w95) -> ()  [unwired: 2 in, 2 out]
        n22 = property on="table.Stats" class="Tbl (strict)"("Active Cell"=w92, "Cell BG Color"=w93, "Index Values"=T16 {"Row"=0, "Column"=0}) -> ()  [unwired: 2 in, 2 out]
        n23 = local write "Tables"(enum32{"Data", "Stats", "Notes"}."Data" ("Tables")) -> ()
        n24 = local write "Pump# Pages"(enum32{"SN", "Auto"}."SN" ("Pump# Pages")) -> ()
        n25 = local write "Starting Serial Number"(w105) -> ()
        n26 = local write "Serial Number Step"(w105) -> ()
        n27 = local write "Ending Serial Number"(u32 2 ("Starting Serial Number")) -> ()
        n28 = local write "table.Data"(w87) -> ()
        n29 = local write "table.Stats"(w87) -> ()
        n30 = local write "Parameters"(w87) -> ()
        n31 = property on="pb.RetryRIO" class="Bool (strict)"("BoolText.Text"="Connect\nto\nRIO" ("Boolean Text.Text")) -> ()  [unwired: 2 in, 2 out]
        n32 = property on="Stabilized?" class="Bool (strict)"("Colors [4]"=w101) -> ()  [unwired: 2 in, 2 out]
        n33 = local write "Setpoint1"(w103) -> ()
        n34 = local write "Setpoint2"(w103) -> ()
        n35 = local write "Setpoint3"(w103) -> ()
        n36 = call <vilib>:"Application Directory.vi"() -> ("Application Directory"=w88:path)
        n37 = local write "Notes"(w89) -> ()
        n38 = local write "File Location"(w89) -> ()
        n39 = local write "Serial Number"(w89) -> ()
        n40 = local write "RS File Location"(w89) -> ()
        n41 = property on="Controller CMD" class="DigNum (strict)"("Visible"=TRUE) -> ()  [unwired: 2 in, 2 out]
        n42 = local write "Tab.Buttons"(enum32{"Manual", "Test"}."Manual" ("Tab.Buttons")) -> ()
        n43 = property on="pb.GrabData" class="Bool"("DisabledEnum"=T17."Disabled and Grayed Out" ("Disabled")) -> ()  [unwired: 2 in, 2 out]
        n44 = Insert Into Array(array=w86, index=0, new element="Init 2" ("new element/subarray")) -> (w85:string[])
        n45 = Build Path(base path=w88, name or relative path="Files\\Template.xlsx") -> (appended path=w90:path)
        n46 = Bundle By Name(cluster=w99, "TemplatePath"=w90, "CommandCluster.Para3"=w97) -> (w98:T15)
        n47 = local write "Parameter 3"(w97) -> ()
        n48 = local write "Parameter 1"(T3."Voltage" ("Parameter 1")) -> ()
        n49 = local write "Parameter 2"(enum16{"Voltage", "Pressure", "Flow", "Speed"}."Pressure" ("Parameter 2")) -> ()
        n50 = property on="Parameter 1" class="Enum (strict)"("Disabled Items []"=i32[] [1]) -> ()  [unwired: 2 in, 2 out]
        n51 = property on="Parameter 2" class="Enum (strict)"("Disabled Items []"=i32[] [0]) -> ()  [unwired: 2 in, 2 out]
        n52 = property on="Parameter 3" class="Enum (strict)"("Disabled Items []"=i32[] [0, 1]) -> ()  [unwired: 2 in, 2 out]
        n53 = property on="pb.Pause Test" class="Bool (strict)"("DisabledEnum"=w76) -> ()  [unwired: 2 in, 2 out]
        n54 = property on="pb.Skip Step" class="Bool"("DisabledEnum"=w76) -> ()  [unwired: 2 in, 2 out]
        n55 = property on="pb.load profile" class="Bool"("DisabledEnum"=w76) -> ()  [unwired: 2 in, 2 out]
        n56 = property on="Voltage (DC)" class="DigNum (strict)"("NumText.TextColor"=w79) -> ()  [unwired: 2 in, 2 out]
        n57 = property on="Pressure (kPa)" class="DigNum (strict)"("NumText.TextColor"=w79) -> ()  [unwired: 2 in, 2 out]
        n58 = property on="Flow (L/H)" class="DigNum (strict)"("NumText.TextColor"=w79) -> ()  [unwired: 2 in, 2 out]
        n59 = property on="Fuel Temp (C)" class="DigNum (strict)"("NumText.TextColor"=w79) -> ()  [unwired: 2 in, 2 out]
        n60 = property on="CtrlrCurrent(A)" class="DigNum (strict)"("NumText.TextColor"=w79) -> ()  [unwired: 2 in, 2 out]
        n61 = property on="PumpCurrent(Arms)" class="DigNum (strict)"("NumText.TextColor"=w79) -> ()  [unwired: 2 in, 2 out]
        n62 = property on="Speed (RPM)" class="DigNum (strict)"("NumText.TextColor"=w79) -> ()  [unwired: 2 in, 2 out]
        n63 = property on="Efficiency (%)" class="DigNum (strict)"("NumText.TextColor"=w79) -> ()  [unwired: 2 in, 2 out]
        n64 = property on="pb.StartManual" class="Bool (strict)"("DisabledEnum"=w96) -> ()  [unwired: 2 in, 2 out]
        n65 = property on="Serial Number" class="Str"("DisabledEnum"=w96) -> ()  [unwired: 2 in, 2 out]
        n66 = property on="Setpoint1" class="DigNum (strict)"("DisabledEnum"=w96) -> ()  [unwired: 2 in, 2 out]
        n67 = property on="Setpoint2" class="DigNum (strict)"("DisabledEnum"=w96) -> ()  [unwired: 2 in, 2 out]
        n68 = property on="Setpoint3" class="DigNum (strict)"("DisabledEnum"=w96) -> ()  [unwired: 2 in, 2 out]
        n69 = property on="File Location" class="Str"("DisabledEnum"=w81) -> ()  [unwired: 2 in, 2 out]
        n70 = property on="pb.StartTest" class="Bool (strict)"("DisabledEnum"=w81) -> ()  [unwired: 2 in, 2 out]
      }
      frame "Init 2" {
        w147 = T19 {"Row"=0, "Column"=0} ("Selection Start")
        n71 = control-ref of="TestType"() -> (w149:refnum<vi>)
        n72 = flat-sequence {
          tunnel: w126 -> [w164]
          frame #0 {
            n73 = control-ref of="pb.RunScreen"() -> (w169:refnum<vi>)
            n74 = control-ref of="pb.TestConfig"() -> (w168:refnum<vi>)
            n75 = control-ref of="pb.StandConfig"() -> (w167:refnum<vi>)
            n76 = control-ref of="Pump Control Style"() -> (w163:refnum<vi>)
            n77 = call "Tab Handler.vi"("RunScreen Ref"=w169, "Mode"=T21."Init", "Test Config Ref"=w168, "Stand Config Ref"=w167) -> ()  [unwired: 12 in]
            n78 = call "Test Config Update.vi"("StringRefArray"=w164, "Mode"=enum16{"Init", "Clear", "Update"}."Init", "Pump Control Style"=w163) -> ()  [unwired: 12 in, 1 out]
          }
          frame #1 {
            n79 = call "Tab Handler.vi"("Mode"=T21."Test Config") -> ()  [unwired: 15 in]
            n80 = call "Test Config Update.vi"("Mode"=enum16{"Init", "Clear", "Update"}."Clear") -> ()  [unwired: 14 in, 1 out]
          }
        }
        n81 = control-ref of="Pump# Pages"() -> (w150:refnum<vi>)
        n82 = control-ref of="CA Number"() -> (w160:refnum<vi>)
        n83 = control-ref of="Shop Order Number"() -> (w161:refnum<vi>)
        n84 = control-ref of="Customer"() -> (w159:refnum<vi>)
        n85 = control-ref of="Platform"() -> (w158:refnum<vi>)
        n86 = control-ref of="Flow Test Fluid"() -> (w157:refnum<vi>)
        n87 = control-ref of="Fuel Batch Number"() -> (w156:refnum<vi>)
        n88 = control-ref of="Pump Model"() -> (w155:refnum<vi>)
        n89 = control-ref of="Technician Name"() -> (w154:refnum<vi>)
        n90 = control-ref of="Durability Tank Number"() -> (w153:refnum<vi>)
        n91 = control-ref of="Durability Fluid"() -> (w152:refnum<vi>)
        n92 = control-ref of="Hours Completed"() -> (w151:refnum<vi>)
        n93 = control-ref of="Parameters"() -> (w148:refnum<vi>)
        n94 = Build Array(w160, w161, w159, w158, w157, w156, w155, w154, w153, w152, w151) -> (w126:refnum<vi>[])
        n95 = call "Test Config Enabler.vi"("StringRefArray"=w126, "Mode"=enum16{"Init", "Enable", "Disable", "AutoPop"}."Init", "TabRef"=w150, "RadioButtonRef"=w149, "TableRef"=w148) -> ()  [unwired: 11 in]
        n96 = property on="table.Data" class="Tbl (strict)"("Index Values"=w147) -> ()  [unwired: 2 in, 2 out]
        n97 = property on="table.Stats" class="Tbl (strict)"("Index Values"=w147) -> ()  [unwired: 2 in, 2 out]
        n98 = property on="Parameters" class="Tbl (strict)"("Index Values"=w147) -> ()  [unwired: 2 in, 2 out]
        n99 = property on="Serial Numbers" class="Tbl (strict)"("Index Values"=w147) -> ()  [unwired: 2 in, 2 out]
        n100 = property on="Untested Serial Numbers" class="Tbl (strict)"("Index Values"=w147) -> ()  [unwired: 2 in, 2 out]
        n101 = property on="Tested Serial Numbers" class="Tbl (strict)"("Index Values"=w147) -> ()  [unwired: 2 in, 2 out]
        n102 = control-ref of="Parameter 3"() -> (w139:refnum<vi>)
        n103 = control-ref of="table.Stats"() -> (w129:refnum<vi>)
        n104 = control-ref of="table.Data"() -> (w128:refnum<vi>)
        n105 = call "Handle Parameter 3 Control.vi"("Reference In"=w139, "Mode"=enum16{"Init", "Set"}."Init") -> ()  [unwired: 11 in, 3 out]
        n106 = call "Full Table Handler.vi"("Init"=TRUE, "DataTableRef"=w128, "StatTableRef"=w129) -> ()  [unwired: 13 in]
        n107 = property on="Parameters" class="Tbl (strict)"("Active Cell"=T19 {"Row"=-2, "Column"=-2} ("Active Cell:Active Cell"), "Cell BG Color"=u32 16777225 ("White"), "Active Cell"=T19 {"Row"=1, "Column"=-2} ("Active Cell:Active Cell"), "Cell BG Color"=u32 9868950) -> ()  [unwired: 2 in, 2 out]
        n108 = control-ref of="Voltage (DC)"() -> (w123:refnum<vi>)
        n109 = control-ref of="Pressure (kPa)"() -> (w122:refnum<vi>)
        n110 = control-ref of="Flow (L/H)"() -> (w121:refnum<vi>)
        n111 = control-ref of="Fuel Temp (C)"() -> (w120:refnum<vi>)
        n112 = control-ref of="PumpCurrent(Arms)"() -> (w119:refnum<vi>)
        n113 = control-ref of="CtrlrCurrent(A)"() -> (w118:refnum<vi>)
        n114 = control-ref of="Efficiency (%)"() -> (w117:refnum<vi>)
        n115 = control-ref of="Controller CMD"() -> (w116:refnum<vi>)
        n116 = control-ref of="Speed (RPM)"() -> (w115:refnum<vi>)
        n117 = property class="App"() -> ("App.Kind"=w146:T20)  [unwired: 2 in, 2 out]
        n118 = Build Array(w123, w122, w121, w120, w119, w118, w117, w116, w115) -> (w114:refnum<vi>[])
        n119 = Bundle By Name(cluster=w125, "DataDisplayRefs"=w114) -> (w124:T15)
        n120 = local write "TestType"(enum32{"Flow", "Test", "Hot\nFuel"}."Flow" ("Enum.Radio")) -> ()
        n121 = control-ref of="Max Command"() -> (w134:refnum<vi>)
        n122 = control-ref of="Min Command"() -> (w133:refnum<vi>)
        n123 = control-ref of="Setpoint3"() -> (w137:refnum<vi>)
        n124 = control-ref of="Setpoint2"() -> (w136:refnum<vi>)
        n125 = control-ref of="Setpoint1"() -> (w135:refnum<vi>)
        n126 = Equal?(x=w146, y=T20."Development System" ("Application:Kind")) -> (x = y?=w113:bool)
        n127 = Build Array(w134, w133) -> (w132:refnum<vi>[])
        n128 = call "Set Parameter Controls.vi"("Controls Mode (Set)"=Parameter_Controls_Mode."Init" ("Controls Mode"), "Para 1 Ref"=w135, "Para 2 Ref"=w136, "Para 3 Ref"=w137, "Min/Max Refs"=w132) -> ()  [unwired: 10 in, 1 out]
        n129 = property on="Screen" class="TabCtl (strict)"("Tabs Visible?"=w113) -> ()  [unwired: 2 in, 2 out]
      }
      frame "Load Config" {
        n130 = Unbundle By Name(w204) -> ("CurrentDataFile"=w174:path, "StandConfigCluster"=w206:T14, "IP Address"=w207:string, "DefaultDataPath"=w175:path, "Gauge Number"=w185:string, "ExpectedFPGA"=w178:i32)
        n131 = call <vilib>:"Application Directory.vi"() -> ("Application Directory"=w182:path)
        n132 = Build Path(base path=w182, name or relative path="Files\\Config.ini") -> (appended path=w183:path)
        n133 = Bundle("CurrentDataFile"=w174, "StandConfigCluster"=w206, "IP Address"=w207, "DefaultDataPath"=w175, "Gauge Number"=w185, "ExpectedFPGA"=w178) -> (w186:T24)  [unwired: 1 in]
        n134 = call "Read Write Config.vi"("Config File"=w183, "Read?"=TRUE, "Cluster In"=w186) -> ("Cluster Out"=w202:T24)  [unwired: 11 in, 1 out]
        n135 = Unbundle(w202) -> ("CurrentDataFile"=w173:path, "StandConfigCluster"=w177:T14, "IP Address"=w187:string, "DefaultDataPath"=w172:path, "Gauge Number"=w184:string, "ExpectedFPGA"=w176:i32)
        n136 = call "Test Config Enabler.vi"("Mode"=enum16{"Init", "Enable", "Disable", "AutoPop"}."Disable") -> ()  [unwired: 15 in]
        n137 = Unbundle By Name(w177) -> ("Max Voltage"=w200:dbl, "Voltage Tolerance"=w199:dbl, "Max Current"=w188:dbl, "Max Pressure"=w198:dbl, "Pressure Tolerance"=w197:dbl, "Min Flow"=w196:dbl, "Max Flow"=w195:dbl, "Flow Tolerance"=w194:dbl, "Speed Tolerance"=w193:dbl, "Stable Count"=w180:dbl, "Parameter Timeout"=w192:dbl, "Init Free Flow"=w191:dbl, "Free Flow Voltage"=w190:dbl, "Free Flow Pressure"=w189:dbl)
        n138 = local write "IP Address"(w187) -> ()
        n139 = local write "Gauge Number"(w184) -> ()
        n140 = local write "IP Address 2"(w187) -> ()
        n141 = local write "Max Voltage"(w200) -> ()
        n142 = local write "Voltage Tolerance"(w199) -> ()
        n143 = local write "Max Current"(w188) -> ()
        n144 = local write "Max Pressure"(w198) -> ()
        n145 = local write "Pressure Tolerance"(w197) -> ()
        n146 = local write "Min Flow"(w196) -> ()
        n147 = local write "Max Flow"(w195) -> ()
        n148 = local write "Flow Tolerance"(w194) -> ()
        n149 = local write "Speed Tolerance"(w193) -> ()
        n150 = local write "Stable Count (sec)"(w180) -> ()
        n151 = local write "Parameter Timeout (sec)"(w192) -> ()
        n152 = local write "Init Free Flow (sec)"(w191) -> ()
        n153 = local write "Free Flow Voltage"(w190) -> ()
        n154 = local write "Free Flow Pressure"(w189) -> ()
        n155 = Bundle By Name(cluster=w204, "StandConfigCluster"=w177, "PreviousDataFile"=w173, "IP Address"=w187, "DefaultDataPath"=w172, "Gauge Number"=w184, "ExpectedFPGA"=w176) -> (w203:T15)
        n156 = Increment(x=w180) -> (x+1=w179:dbl)
        n157 = property on="Parameter Timeout (sec)" class="DigNum (strict)"("Minimum"=w179) -> ()  [unwired: 2 in, 2 out]
      }
      frame "Load Data File" {
        # "Removed Gauge #\nand Cal Due Date"
        n158 = Unbundle By Name(w272) -> ("CurrentDataFile"=w257:path, "TemplatePath"=w219:path, "Controller List"=w235:T9, "StandConfigCluster"=w228:T14, "Stability Cluster"=w214:T5)
        n159 = Empty String/Path?(string/path=w257) -> (empty?=w268:bool)
        n160 = call <vilib>:"Check if File or Folder Exists.vi"("path"=w257) -> ("file or folder exists?"=w267:bool, "dup path"=w256:path)  [unwired: 8 in, 1 out]
        n161 = Not(x=w268) -> (.not. x?=w266:bool)
        n162 = property on="pb.save" class="Bool"("DisabledEnum"=T17."Disabled and Grayed Out" ("Disabled")) -> ()  [unwired: 2 in, 2 out]
        n163 = And(x=w266, y=w267) -> (x .and. y?=w237:bool)
        n164 = Select(t=w256, s=w237, f=w219) -> (s? t:f=w265:path)
        n165 = Select(t=w257, s=w237, f=path "") -> (s? t:f=w262:path)
        n166 = call "Read Data File.vi"("Filepath"=w265, "Controller List"=w235, "ValidFile?"=w237, "TemplatePath"=w219) -> ("Notes"=w264:string, "TestCfgCluster"=w223:T11, "Data"=w217:string[][], "Stats"=w221:string[][], "Profile"=w238:string[][], "Test Style"=w229:enum32{"Flow", "Test", "Hot\nFuel"}, "Part#s"=w234:string[], "Controller"=w215:T10)  [unwired: 3 in, 1 out]
        n167 = Path To String(path=w262) -> (string=w236:string)
        "RS File Location" <- w236
        n168 = local write "File Location"(w236) -> ()
        n169 = Insert Into Array(array=w211, index=0, new element=string[] ["Write Command", "PS Abler", "Alter Parameter Setup", "Alter Run Screen", "Eval Parameters", "Evaluate SNs"]) -> (w210:string[])
        n170 = call "SN Sort.vi"("Array In"=w234) -> ("Array Out"=w233:string[])  [unwired: 14 in]
        n171 = local write "TestType"(w229) -> ()
        n172 = Build Array(w233) -> (w261:string[][])
        n173 = Transpose 2D Array(2D array=w261) -> (transposed array=w260:string[][])
        n174 = local write "Notes"(w264) -> ()
        n175 = local write "table.Stats"(w221) -> ()
        n176 = local write "Serial Numbers"(w260) -> ()
        n177 = local write "Parameters"(w238) -> ()
        n178 = Unbundle By Name(w215) -> ("Stop Command"=w251:dbl, "Controller?"=w252:bool, "Controller Name"=w239:T4)
        n179 = Select(t=enum16{"Init", "Enable", "Disable", "AutoPop"}."Enable" ("Mode"), s=w237, f=enum16{"Init", "Enable", "Disable", "AutoPop"}."Disable" ("Mode")) -> (s? t:f=w227:enum16{"Init", "Enable", "Disable", "AutoPop"})
        n180 = Unbundle By Name(w215) -> ("Controller Name"=w218:T4, "Controller?"=w222:bool, "Command Step"=w212:dbl)
        n181 = call "Create Loaded Stat Bundle.vi"("StatArray"=w221, "CMD Step"=w212) -> ("StatBundle Out"=w216:T7)  [unwired: 13 in]
        n182 = call "Apply Desired to Imported Data.vi"("table.Data In"=w217, "StatBundle"=w216, "Controller"=w215, "Stability Cluster"=w214) -> ("table.Data Out"=w213:string[][])  [unwired: 11 in]
        n183 = call "Full Table Handler.vi"("table.Data"=w213, "table.Stats"=w221) -> ()  [unwired: 14 in]
        n184 = local write "table.Data"(w213) -> ()
        n185 = call "Test Config Enabler.vi"("Mode"=w227) -> ()  [unwired: 15 in]
        n186 = To Long Integer(number=w239) -> (32bit integer=w242:i32)
        n187 = Select(t="Pump Current\n(A RMS)" ("Caption.Text"), s=w222, f="Pump Current\n(A)" ("Caption.Text")) -> (s? t:f=w230:string)
        n188 = Flatten To String(anything=w242) -> (data string=w243:string, error out=w241:errorcluster)  [unwired: 3 in, 1 out]
        n189 = Not(x=w222) -> (.not. x?=w224:bool)
        n190 = property on="PumpCurrent(Arms)" class="DigNum (strict)"("Caption.Text"=w230) -> ()  [unwired: 2 in, 2 out]
        n191 = Select(t=w251, s=w252, f=0.0) -> (s? t:f=w209:dbl)
        n192 = Bundle(cluster=T22 {"Command"="", "FlattenedData"=""}, "Command"="Controller", "FlattenedData"=w243) -> (w245:T22)
        n193 = call "Set Parameter Controls.vi"("Controls Mode (Set)"=Parameter_Controls_Mode."Update Ranges", "StandConfigCluster"=w228, "Controller"=w215) -> ("Error Out"=w220:errorcluster)  [unwired: 12 in]
        n194 = Flatten To String(anything=w245, error in (no error)=w241) -> (data string=w247:string, error out=w240:errorcluster)  [unwired: 2 in, 1 out]
        n195 = Select(t="Pump\nVoltage (V)", s=w224, f="Controller\nVoltage (V)") -> (s? t:f=w253:string)
        n196 = call "PC Send Event.vi"("PC Send Command"=PCsend_RTrecv_CMD."Controller", "Mode"=Event_Mode."Set", "Flattened Data"=w247, "Error In"=w240) -> ()  [unwired: 10 in, 2 out]
        n197 = property on="Voltage (DC)" class="DigNum (strict)"("Caption.Text"=w253) -> ()  [unwired: 2 in, 2 out]
        n198 = Bundle By Name(cluster=w272, "CurrentDataFile"=w262, "ValidFile?"=w237, "Notes"=w264, "table.Data"=w213, "table.Stats"=w221, "TestCfgCluster"=w223, "Serial Numbers"=w233, "Parameters"=w238, "Controller"=w215, "TestCfgCluster.Pump Control Style"=w218, "CommandCluster.SP3"=w209, "DesiredParameters.SP3"=w209, "StatBundle"=w216) -> (w271:T15)
        n199 = flat-sequence {
          tunnel: w209 -> [w273]
          tunnel: w220 -> [_]
          frame #0 {
            n200 = local write "Setpoint3"(w273) -> ()
          }
        }
      }
      frame "No IP" {
        n201 = call "Tab Handler.vi"("Mode"=T21."Other Tab") -> ()  [unwired: 15 in]
        n202 = Insert Into Array(array=w279, index=0, new element=string[] ["Unset Cursor Busy", "RIO Connection"]) -> (w276:string[])
        n203 = One Button Dialog(message="No IP address was found for the RIO. An IP address is necessary to connect.") -> ()  [unwired: 1 in, 1 out]
      }
      frame "Connect to RIO" {
        n204 = Unbundle By Name(w288) -> ("RIOTries"=w281:i32)
        n205 = case shown="0..4, Default" w281 {
          tunnel: [w295 string[] ["Unset Cursor Busy", "RIO Connection"]] -> w285
          tunnel: w281 -> [w294 _]
          tunnel: [w293 0] -> w282
          frame 0..4, Default {
            n206 = Increment(x=w294) -> (x+1=w293:i32)
            n207 = for {
              tunnel: string[] ["Connecting", "Connecting.", "Connecting..", "Connecting..."] -> [w297] mode=indexing
              n208 = property on="pb.RetryRIO" class="Bool (strict)"("BoolText.Text"=w297) -> ()  [unwired: 2 in, 2 out]
              n209 = Wait (ms)(milliseconds to wait=u32 200) -> ()  [unwired: 1 out]
            }
            n210 = And(x="Connected?", y="Connected? 2") -> (x .and. y?=w292:bool)
            n211 = case shown="True" w292 {
              tunnel: [string[] ["***MAIN***", "Connect to RIO"] string[] ["Connected", "Thaw Screen"]] -> w295
              frame False {
              }
              frame True {
              }
            }
          }
          frame 5 {
            n212 = flat-sequence {
              frame #0 {
                n213 = property on="pb.RetryRIO" class="Bool (strict)"("BoolText.Text"="FAILED" ("Boolean Text.Text")) -> ()  [unwired: 2 in, 2 out]
                n214 = Wait (ms)(milliseconds to wait=u32 500) -> ()  [unwired: 1 out]
              }
              frame #1 {
                n215 = property on="pb.RetryRIO" class="Bool (strict)"("BoolText.Text"="Connect\nto\nRIO" ("Boolean Text.Text")) -> ()  [unwired: 2 in, 2 out]
              }
            }
            n216 = local write "pb.RetryRIO"(FALSE ("pb.RetryRIO")) -> ()
          }
        }
        n217 = Bundle By Name(cluster=w288, "RIOTries"=w282) -> (w287:T15)
        n218 = Insert Into Array(array=w286, index=0, new element=w285) -> (w283:string[])
      }
      frame "Connected" {
        w347 = T5 {"Voltage Tolerances"=0.0, "Pressure Tolerances"=0.0, "Flow Tolerances"=0.0, "Speed Tolerances"=0.0, "Stable Count (sec)"=0.0}  # Stability Cluster
        # "On startup unset cursor busy is already in the array but need this for reconnection after losing connection to RIO"
        n219 = Unbundle By Name(w374) -> ("StandConfigCluster.Max Voltage"=w324:dbl, "StandConfigCluster.Max Pressure"=w323:dbl, "StandConfigCluster.Voltage Tolerance"=w346:dbl, "StandConfigCluster.Pressure Tolerance"=w345:dbl, "StandConfigCluster.Flow Tolerance"=w344:dbl, "StandConfigCluster.Speed Tolerance"=w343:dbl, "StandConfigCluster.Stable Count"=w342:dbl, "Controller.Controller?"=w365:bool, "CommandCluster"=w370:T6, "Controller.Stop Command"=w373:dbl, "Controller.Controller Name"=w339:T4, "ExpectedFPGA"=w308:i32)
        n220 = To Long Integer(number=w339) -> (32bit integer=w360:i32)
        n221 = Build Array(w324, w323) -> (w326:dbl[])
        n222 = Flatten To String(anything=w360) -> (data string=w361:string, error out=w359:errorcluster)  [unwired: 3 in, 1 out]
        n223 = Bundle(cluster=T22 {"Command"="", "FlattenedData"=""}, "Command"="Controller", "FlattenedData"=w361) -> (w363:T22)
        n224 = Flatten To String(anything=w363, error in (no error)=w359) -> (data string=w356:string, error out=w355:errorcluster)  [unwired: 2 in, 1 out]
        n225 = Select(t=w373, s=w365, f=0.0) -> (s? t:f=w371:dbl)
        n226 = call "PC Send Event.vi"("PC Send Command"=PCsend_RTrecv_CMD."Controller", "Mode"=Event_Mode."Set", "Flattened Data"=w356, "Error In"=w355) -> ("Error Out"=w319:errorcluster)  [unwired: 10 in, 1 out]
        n227 = Bundle By Name(cluster=w370, "SP3"=w371) -> (w318:T6)
        n228 = Unbundle By Name(w318) -> ("Para1"=w338:i32, "SP1"=w376:dbl, "Para2"=w337:i32, "SP2"=w375:dbl, "Para3"=w336:i32)
        n229 = Bundle By Name(cluster=w347, "Voltage Tolerances"=w346, "Pressure Tolerances"=w345, "Flow Tolerances"=w344, "Speed Tolerances"=w343, "Stable Count (sec)"=w342) -> (w320:T5)
        n230 = call "Set Parameter Controls.vi"("Para 1"=w338, "Para 2"=w337, "Para 3"=w336) -> ()  [unwired: 12 in, 1 out]
        n231 = Insert Into Array(array=w368, index=0, new element=string[] ["Write Command", "PS Abler", "Request Cal Date", "Unset Cursor Busy"]) -> (w367:string[])
        n232 = flat-sequence {
          tunnel: w376 -> [w385]
          tunnel: w375 -> [w384]
          tunnel: w371 -> [w383]
          tunnel: w338 -> [w382]
          tunnel: w337 -> [w381]
          tunnel: w336 -> [w380]
          frame #0 {
            n233 = local write "Parameter 1"(w382) -> ()
            n234 = local write "Setpoint1"(w385) -> ()
            n235 = local write "Parameter 2"(w381) -> ()
            n236 = local write "Setpoint2"(w384) -> ()
            n237 = local write "Parameter 3"(w380) -> ()
            n238 = local write "Setpoint3"(w383) -> ()
          }
        }
        n239 = Bundle By Name(cluster=w374, "CommandCluster"=w318, "DesiredParameters"=w318, "Stability Cluster"=w320) -> (w377:T15)
        n240 = Flatten To String(anything=w320, error in (no error)=w319) -> (data string=w350:string, error out=w341:errorcluster)  [unwired: 2 in, 1 out]
        n241 = Bundle(cluster=T22 {"Command"="", "FlattenedData"=""}, "Command"="Tolerances", "FlattenedData"=w350) -> (w352:T22)
        n242 = Flatten To String(anything=w352, error in (no error)=w341) -> (data string=w353:string, error out=w340:errorcluster)  [unwired: 2 in, 1 out]
        n243 = call "Tab Handler.vi"("Mode"=T21."Test Config") -> ()  [unwired: 15 in]
        n244 = call "PC Send Event.vi"("PC Send Command"=PCsend_RTrecv_CMD."Tolerances", "Mode"=Event_Mode."Set", "Flattened Data"=w353, "Error In"=w340) -> ("Error Out"=w321:errorcluster)  [unwired: 10 in, 1 out]
        n245 = Flatten To String(anything=w326, error in (no error)=w321) -> (data string=w334:string, error out=w325:errorcluster)  [unwired: 2 in, 1 out]
        n246 = Bundle(cluster=T22 {"Command"="", "FlattenedData"=""}, "Command"="VPLimits", "FlattenedData"=w334) -> (w332:T22)
        n247 = Flatten To String(anything=w332, error in (no error)=w325) -> (data string=w328:string, error out=w327:errorcluster)  [unwired: 2 in, 1 out]
        n248 = property on="pb.RetryRIO" class="Bool (strict)"("BoolText.Text"="Connect\nto\nRIO" ("Boolean Text.Text")) -> ()  [unwired: 2 in, 2 out]
        n249 = local write "pb.RetryRIO"(FALSE ("pb.RetryRIO")) -> ()
        n250 = local write "Screen"(T1."Test Configuration Page" ("Screen")) -> ()
        n251 = call "PC Send Event.vi"("PC Send Command"=PCsend_RTrecv_CMD."VPLimits", "Mode"=Event_Mode."Set", "Flattened Data"=w328, "Error In"=w327) -> ("Error Out"=w307:errorcluster)  [unwired: 10 in, 1 out]
        n252 = Flatten To String(anything=w308, error in (no error)=w307) -> (data string=w312:string, error out=w313:errorcluster)  [unwired: 2 in, 1 out]
        n253 = Bundle(cluster=T22 {"Command"="", "FlattenedData"=""}, "Command"="LoadFPGA", "FlattenedData"=w312) -> (w310:T22)
        n254 = Flatten To String(anything=w310, error in (no error)=w313) -> (data string=w316:string, error out=w317:errorcluster)  [unwired: 2 in, 1 out]
        n255 = call "PC Send Event.vi"("PC Send Command"=PCsend_RTrecv_CMD."LoadFPGA", "Mode"=Event_Mode."Set", "Flattened Data"=w316, "Error In"=w317) -> ("Error Out"=w306:errorcluster)  [unwired: 10 in, 1 out]
        n256 = disable-structure shown="Disabled" {
          disable-tunnel: w306 -> [_ _]
          frame Disabled {
          }
          frame Enabled {
          }
        }
      }
      frame "Check Template" {
        n257 = Unbundle By Name(w389) -> ("TemplatePath"=w387:path)
        n258 = call <vilib>:"Check if File or Folder Exists.vi"("path"=w387) -> ("file or folder exists?"=w388:bool)  [unwired: 8 in, 2 out]
        n259 = Path To String(path=w387) -> (string=w386:string)
        n260 = case shown="False" w388 {
          tunnel: w386 -> [w392 _]
          frame False {
            n261 = Format Into String(format string="Template file not found!\n\nIt was expected at %s.\n\nPlace template file at correct location or program may not function properly.", w392) -> (resulting string=w391:string)  [unwired: 2 in, 1 out]
            n262 = One Button Dialog(message=w391) -> ()  [unwired: 1 in, 1 out]
          }
          frame True {
          }
        }
      }
      frame "***MAIN***", Default {
        n263 = event shown="[7] \"pb.GrabData\": Value Change" {
          selector: w399 -> [_ _ _ _ _ _ _ _ _ _ _ _ _ _ _ _ _ _ _ _ _ _ _ _ _ _ _ _ _ _ _ _ _ _ _ _ _ _ _ _ _ _ _ _ _ _ _ _ _ _ _]
          dyn-events: _ -> [_ _ _ _ _ _ _ _ _ _ _ _ _ _ _ _ _ _ _ _ _ _ _ _ _ _ _ _ _ _ _ _ _ _ _ _ _ _ _ _ _ _ _ _ _ _ _ _ _ _ _]
          timeout: 10 -> [_ _ _ _ _ _ _ _ _ _ _ _ _ _ _ _ _ _ _ _ _ _ _ _ _ _ _ _ _ _ _ _ _ _ _ _ _ _ _ _ _ _ _ _ _ _ _ _ _ _ _]
          tunnel: [w406 w432 w434 w513 w518 w521 w535 w548 w568 w582 w583 w600 w623 w625 w631 w763 w816 w845 w876 w882 w888 w899 w951 w967 w986 w1005 w1026 w1029 w1036 w1063 w1113 w1117 w1125 w1165 w1216 w1220 w1227 w1230 w1237 w1251 w1263 w1276 w1291 w1304 w1306 w1321 w1326 w1344 w1375 w1378 w1381] -> w397
          tunnel: w398 -> [w406 w432 w436 w513 w518 w521 w535 w548 w561 w582 w584 w600 w623 w626 w649 w783 w834 w859 w876 w882 w888 w897 w951 w967 w986 w1005 w1026 w1029 w1037 w1108 w1113 w1117 w1126 w1177 w1213 w1220 w1228 w1230 w1238 w1251 w1263 w1277 w1292 w1304 w1306 w1321 w1326 w1345 w1375 w1378 w1382]
          tunnel: w396 -> [w403 w431 w435 w514 w517 w522 w537 w555 w562 w580 w587 w603 w622 w630 w638 w769 w824 w852 w875 w881 w887 w900 w961 w977 w988 w1009 w1025 w1028 w1032 w1100 w1112 w1116 w1128 w1142 w1215 w1219 w1226 w1229 w1247 w1250 w1264 w1273 w1288 w1302 w1309 w1320 w1325 w1329 w1374 w1377 w1385]
          tunnel: [w400 w428 w433 w514 w517 w522 w536 w554 w563 w579 w586 w602 w621 w629 w637 w770 w823 w851 w875 w881 w887 w900 w960 w977 w987 w1008 w1025 w1028 w1031 w1099 w1111 w1115 w1127 w1169 w1215 w1219 w1226 w1229 w1247 w1250 w1264 w1272 w1287 w1301 w1308 w1320 w1324 w1328 w1374 w1377 w1384] -> w394
          event Timeout {
            # "KF.Parameters gets set true whenever there is an event that\ncan change the values in the table then when the KF points\nelsewhere the Parameters table is evaluated"
            n264 = event-data() -> ()  [unwired: 1 in, 1 out]
            n265 = Unbundle By Name(w406) -> ("KF.Parameters"=w402:bool, "Free Flow"=w405:bool, "StepTimeLimit"=w404:dbl)
            n266 = case shown="True" w405 {
              tunnel: w403 -> [w416 w418]
              tunnel: [w416 w417] -> w401
              tunnel: w404 -> [_ w420]
              frame False {
              }
              frame True {
                n267 = Get Date/Time In Seconds() -> (seconds since 1Jan1904=w422:timestamp)
                n268 = To Double Precision Float(number=w422) -> (double precision float=w421:dbl)
                n269 = Greater?(x=w421, y=w420) -> (0:w419:bool)
                n270 = case shown="True" w419 {
                  tunnel: w418 -> [w423 w427]
                  tunnel: [w423 w424] -> w417
                  frame False {
                  }
                  frame True {
                    n271 = Insert Into Array(array=w427, index=0, new element=string[] ["Start Test"]) -> (w424:string[])
                  }
                }
              }
            }
            n272 = case shown="True" w402 {
              tunnel: w401 -> [w407 w410]
              tunnel: [w407 w409] -> w400
              frame False {
              }
              frame True {
                n273 = property on="Parameters" class="Tbl (strict)"() -> ("Key Focus"=w408:bool)  [unwired: 2 in, 2 out]
                n274 = case shown="False" w408 {
                  tunnel: w410 -> [w411 w415]
                  tunnel: [w411 w412] -> w409
                  frame True {
                  }
                  frame False {
                    n275 = Insert Into Array(array=w415, index=0, new element=string[] ["Store Parameters", "Eval Parameters"]) -> (w412:string[])
                  }
                }
              }
            }
          }
          event "Panel Close?": Value Change {
            n276 = event-data() -> ()  [unwired: 1 in, 1 out]
            n277 = Insert Into Array(array=w431, index=0, new element=string[] ["Exit Preparation"]) -> (w428:string[])
          }
          event User Event {
            n278 = event-data() -> ("RTsend/PCrecv CMD"=w438:T25, "Flattened Data"=w437:string)  [unwired: 1 in]
            n279 = case shown="\"Data\"" w438 {
              tunnel: w437 -> [_ w463 w482 w503]
              tunnel: w436 -> [w440 w461 w479 w500]
              tunnel: w435 -> [w439 w455 w475 w504]
              tunnel: [w440 w462 w480 w499] -> w434
              tunnel: [w439 w454 w474 w504] -> w433
              frame Default {
              }
              frame "Data" {
                w460 = T13 {"Pump Voltage (V)"=0.0, "Pump Current (Arms)"=0.0, "Pressure (kPA)"=0.0, "Flow (L/H)"=0.0, "Controller Voltage (V)"=0.0, "Controller Current (A)"=0.0, "Fuel Temp (C)"=0.0, "Speed (RPM)"=0.0, "Efficiency (%)"=0.0, "Stabilized?"=FALSE, "Controller CMD"=0.0}  # DataCluster
                n280 = Unbundle By Name(w461) -> ("DesiredParameters"=w443:T6, "Stability Cluster"=w444:T5, "Controller.Controller?"=w446:bool, "DataDisplayRefs"=w445:refnum<vi>[], "TestRunning?"=w459:bool, "WaitingData"=w458:bool, "StepDataActive"=w457:dbl, "Free Flow"=w456:bool, "StepTimeLimit"=w453:dbl, "LastDataTime"=w450:i64, "StandConfigCluster.Stable Count"=w451:dbl)
                n281 = Unflatten From String(type=w460, binary string=w463) -> (value=w448:T13)  [unwired: 3 in, 2 out]
                n282 = local read "TestType"() -> (w452:enum32{"Flow", "Test", "Hot\nFuel"})
                n283 = control-ref of="Stabilized?"() -> (w447:refnum<vi>)
                n284 = call "Write Values and Check for Stabilization.vi"("DataCluster In"=w448, "DesiredParameters"=w443, "Stability Cluster"=w444, "Controller?"=w446, "DataDisplayRefs"=w445, "StabilizedRef"=w447) -> ("DataCluster Out"=w442:T13)  [unwired: 9 in]
                n285 = Unbundle By Name(w442) -> ("Stabilized?"=w441:bool)
                n286 = call "Test Sequencer.vi"("WaitingData"=w458, "TestRunning?"=w459, "Stabilized?"=w441, "Stabilized"=w447, "StepDataActive"=w457, "FreeFlow"=w456, "StepTimeLimit"=w453, "State Array In"=w455, "LastDataTime"=w450, "StableCount"=w451, "TestType"=w452) -> ("FreezeCmdPID"=w449:bool, "State Array Out"=w454:string[])  [unwired: 3 in]
                n287 = case shown="True" w449 {
                  frame False {
                  }
                  frame True {
                    n288 = Flatten To String(anything=TRUE) -> (data string=w469:string, error out=w468:errorcluster)  [unwired: 3 in, 1 out]
                    n289 = Bundle(cluster=T22 {"Command"="", "FlattenedData"=""}, "Command"="FreezeCmdPID", "FlattenedData"=w469) -> (w471:T22)
                    n290 = Flatten To String(anything=w471, error in (no error)=w468) -> (data string=w466:string, error out=w465:errorcluster)  [unwired: 2 in, 1 out]
                    n291 = call "PC Send Event.vi"("PC Send Command"=PCsend_RTrecv_CMD."FreezeCmdPID", "Mode"=Event_Mode."Set", "Flattened Data"=w466, "Error In"=w465) -> ()  [unwired: 10 in, 2 out]
                  }
                }
                n292 = Bundle By Name(cluster=w461, "DataCluster"=w442) -> (w462:T15)
              }
              frame "Connected?" {
                n293 = Unbundle By Name(w479) -> ("RIOconnection"=w477:bool)
                n294 = Unflatten From String(type=TRUE, binary string=w482) -> (value=w478:bool)  [unwired: 3 in, 2 out]
                n295 = Less?(x=w478, y=w477) -> (x < y?=w476:bool)
                n296 = Bundle By Name(cluster=w479, "RIOconnection"=w478) -> (w480:T15)
                n297 = local write "Connected?"(w478) -> ()
                n298 = local write "Connected? 2"(w478) -> ()
                n299 = case shown="True" w476 {
                  tunnel: w475 -> [w483 w488]
                  tunnel: [w483 w487] -> w474
                  frame False {
                  }
                  frame True {
                    n300 = local write "pb.RetryRIO"(FALSE ("pb.RetryRIO")) -> ()
                    n301 = call "Tab Handler.vi"("Mode"=T21."Other Tab") -> ()  [unwired: 15 in]
                    n302 = property on="pb.RetryRIO" class="Bool (strict)"("BoolText.Text"="Connect\nto\nRIO" ("Boolean Text.Text")) -> ()  [unwired: 2 in, 2 out]
                    n303 = Insert Into Array(array=w488, index=0, new element=string[] ["Unset Cursor Busy", "RIO Connection"]) -> (w487:string[])
                  }
                }
              }
              frame "CalFileDate" {
                n304 = Unflatten From String(type=cluster{i32, u8} {0, 0}, binary string=w503) -> (value=w494:cluster{i32, u8})  [unwired: 3 in, 2 out]
                n305 = Unbundle(w494) -> (w493:i32, w492:u8)
                n306 = case shown="2" w492 {
                  tunnel: ["Standard" "Portable" "Warranty"] -> w491
                  frame 0, Default {
                  }
                  frame 1 {
                  }
                  frame 2 {
                  }
                }
                "Hardware Style" <- w491
                n307 = call "Cal Date Valid.vi"("PrevCalDate"=w493) -> ("Cal Valid?"=w496:bool, "Calibration Due Date"=w497:string)  [unwired: 9 in]
                "Calibration Due Date" <- w497
                n308 = Select(t=u32 0, s=w496, f=u32 16711680) -> (s? t:f=w498:u32)
                n309 = case shown="False" w496 {
                  frame True {
                  }
                  frame False {
                    n310 = flat-sequence {
                      frame #0 {
                        n311 = local write "Screen"(T1."Cal Warning" ("Screen")) -> ()
                      }
                      frame #1 {
                        n312 = Wait (ms)(milliseconds to wait=u32 2500) -> ()  [unwired: 1 out]
                      }
                      frame #2 {
                        n313 = local write "Screen"(T1."Test Configuration Page" ("Screen")) -> ()
                      }
                    }
                  }
                }
                n314 = property on="Voltage (DC)" class="DigNum (strict)"("NumText.TextColor"=w498) -> ()  [unwired: 2 in, 2 out]
                n315 = property on="Pressure (kPa)" class="DigNum (strict)"("NumText.TextColor"=w498) -> ()  [unwired: 2 in, 2 out]
                n316 = property on="Flow (L/H)" class="DigNum (strict)"("NumText.TextColor"=w498) -> ()  [unwired: 2 in, 2 out]
                n317 = property on="Fuel Temp (C)" class="DigNum (strict)"("NumText.TextColor"=w498) -> ()  [unwired: 2 in, 2 out]
                n318 = property on="CtrlrCurrent(A)" class="DigNum (strict)"("NumText.TextColor"=w498) -> ()  [unwired: 2 in, 2 out]
                n319 = property on="PumpCurrent(Arms)" class="DigNum (strict)"("NumText.TextColor"=w498) -> ()  [unwired: 2 in, 2 out]
                n320 = property on="Speed (RPM)" class="DigNum (strict)"("NumText.TextColor"=w498) -> ()  [unwired: 2 in, 2 out]
                n321 = property on="Efficiency (%)" class="DigNum (strict)"("NumText.TextColor"=w498) -> ()  [unwired: 2 in, 2 out]
                n322 = Bundle By Name(cluster=w500, "Calibration Due Date"=w497) -> (w499:T15)
              }
            }
          }
          event "pb.RunScreen": Value Change {
            n323 = event-data() -> ()  [unwired: 1 in, 1 out]
            n324 = call "Tab Handler.vi"("Mode"=T21."Run Screen") -> ()  [unwired: 15 in]
            n325 = local write "Screen"(T1."Run Screen" ("Screen")) -> ()
          }
          event "pb.TestConfig": Value Change {
            n326 = event-data() -> ()  [unwired: 1 in, 1 out]
            n327 = call "Tab Handler.vi"("Mode"=T21."Test Config") -> ()  [unwired: 15 in]
            n328 = local write "Screen"(T1."Test Configuration Page" ("Screen")) -> ()
          }
          event "pb.StandConfig": Value Change {
            n329 = event-data() -> ()  [unwired: 1 in, 1 out]
            n330 = call "Tab Handler.vi"("Mode"=T21."Stand Config") -> ()  [unwired: 15 in]
            n331 = local write "Screen"(T1."Stand Configuration Page" ("Screen")) -> ()
          }
          event "pb.StartManual": Value Change {
            n332 = event-data() -> ()  [unwired: 1 in, 1 out]
            n333 = Unbundle By Name(w535) -> ("ValidFile?"=w525:bool, "ValidPara?"=w526:bool, "Controller.Stop Command"=w523:dbl)
            n334 = And(x=w525, y=w526) -> (x .and. y?=w524:bool)
            n335 = case shown="False" "pb.StartManual" {
              tunnel: [string[] ["Stop Manual", "Alter Run Screen"] string[] ["Write Command", "Alter Run Screen"]] -> w539
              tunnel: T17."Enabled" ("Disabled") -> [_ w545]
              tunnel: T17."Disabled and Grayed Out" ("Disabled") -> [w541 _]
              tunnel: [w541 w545] -> w527
              tunnel: w524 -> [_ _]
              tunnel: w523 -> [_ _]
              frame False {
                n336 = call "Tab Handler.vi"("Mode"=T21."Run Screen") -> ()  [unwired: 15 in]
              }
              frame True {
                w543 = u16 0 items=["Manual", "1)   V=1, P=1, C=15", "2)   V=2, P=2, C=15", "3)   V=3, P=3, C=15"] ("Steps")
                n337 = call "Tab Handler.vi"("Mode"=T21."Lock All") -> ()  [unwired: 15 in]
                n338 = local write "Steps"(w543) -> ()
              }
            }
            n339 = Compound Arithmetic op=AND(w524, invert "pb.StartManual") -> (w533:bool)
            n340 = Select(t=T17."Enabled" ("Disabled"), s=w533, f=T17."Disabled and Grayed Out" ("Disabled")) -> (s? t:f=w534:T17)
            n341 = Insert Into Array(array=w537, index=0, new element=w539) -> (w536:string[])
            n342 = property on="pb.StartTest" class="Bool (strict)"("DisabledEnum"=w534) -> ()  [unwired: 2 in, 2 out]
            n343 = property on="pb.GrabData" class="Bool"("DisabledEnum"=w527) -> ()  [unwired: 2 in, 2 out]
          }
          event "pb.GrabData": Value Change {
            n344 = event-data() -> ()  [unwired: 1 in, 1 out]
            n345 = Unbundle By Name(w548) -> ("LastDataTime"=w551:i64)
            n346 = Get Date/Time In Seconds() -> (seconds since 1Jan1904=w553:timestamp)
            n347 = To Double Precision Float(number=w553) -> (double precision float=w549:dbl)
            n348 = Round Toward -Infinity(1:w549) -> (0:w552:dbl)
            n349 = To Quad Integer(1:w552) -> (0:w550:i64)
            n350 = Not Equal?(x=w551, y=w550) -> (x != y?=w547:bool)
            n351 = case shown="True" w547 {
              tunnel: w555 -> [w556 w559]
              tunnel: [w556 w558] -> w554
              frame False {
              }
              frame True {
                n352 = Insert Into Array(array=w559, index=0, new element=string[] ["Freeze Screen", "Store Data", "Find Stats", "Save Data", "Thaw Screen"]) -> (w558:string[])
              }
            }
          }
          event "pb.new": Value Change {
            n353 = event-data() -> ()  [unwired: 1 in, 1 out]
            n354 = Unbundle By Name(w561) -> ("ValidFile?"=w565:bool, "table.Data"=w564:string[][])
            n355 = Empty Array?(array=w564) -> (empty?=w566:bool)
            n356 = Or(x=w565, y=w566) -> (x .or. y?=w567:bool)
            n357 = case shown="True" w567 {
              tunnel: w562 -> [w573 w577]
              tunnel: [w572 w576] -> w563
              frame True {
                n358 = Insert Into Array(array=w573, index=0, new element="New File" ("new element/subarray")) -> (w572:string[])
              }
              frame False {
                n359 = Insert Into Array(array=w577, index=0, new element="Save Check New" ("new element/subarray")) -> (w576:string[])
              }
            }
            n360 = Bundle By Name(cluster=w561, "LastFileState"=enum16{"New File", "Load File", "Neither"}."New File") -> (w568:T15)
          }
          event "pb.save": Value Change {
            n361 = event-data() -> ()  [unwired: 1 in, 1 out]
            n362 = Insert Into Array(array=w580, index=0, new element=string[] ["Store Parameters", "Eval Parameters", "Save Test Config"]) -> (w579:string[])
          }
          event "pb.load": Value Change {
            n363 = event-data() -> ()  [unwired: 1 in, 1 out]
            n364 = Unbundle By Name(w584) -> ("ValidFile?"=w589:bool, "table.Data"=w591:string[][])
            n365 = Empty Array?(array=w591) -> (empty?=w590:bool)
            n366 = Or(x=w589, y=w590) -> (x .or. y?=w588:bool)
            n367 = case shown="True" w588 {
              tunnel: w587 -> [w595 w599]
              tunnel: [w594 w598] -> w586
              frame True {
                n368 = Insert Into Array(array=w595, index=0, new element="Load File" ("new element/subarray")) -> (w594:string[])
              }
              frame False {
                n369 = Insert Into Array(array=w599, index=0, new element="Save Check Load" ("new element/subarray")) -> (w598:string[])
              }
            }
            n370 = Bundle By Name(cluster=w584, "LastFileState"=enum16{"New File", "Load File", "Neither"}."Load File") -> (w583:T15)
          }
          event "pb.StartTest": Value Change {
            n371 = event-data() -> ()  [unwired: 1 in, 1 out]
            n372 = case shown="False" "pb.StartTest" {
              tunnel: w603 -> [w609 w614]
              tunnel: [w608 w613] -> w602
              frame True {
                # "Start Test"
                n373 = call "Tab Handler.vi"("Mode"=T21."Lock All") -> ()  [unwired: 15 in]
                n374 = local write "Tab.Buttons"(enum32{"Manual", "Test"}."Test" ("Tab.Buttons")) -> ()
                n375 = Insert Into Array(array=w609, index=0, new element=string[] ["PS Abler", "Evaluate SNs", "Start Test Prep"]) -> (w608:string[])
              }
              frame False {
                n376 = call "Tab Handler.vi"("Mode"=T21."Run Screen") -> ()  [unwired: 15 in]
                n377 = local write "Tab.Buttons"(enum32{"Manual", "Test"}."Manual" ("Tab.Buttons")) -> ()
                n378 = Insert Into Array(array=w614, index=0, new element=string[] ["Stop Test"]) -> (w613:string[])
              }
            }
          }
          event "pb.Pause Test": Value Change {
            n379 = event-data() -> ()  [unwired: 1 in, 1 out]
            n380 = Select(t="Pause Test" ("new element/subarray"), s="pb.Pause Test", f="Resume Test" ("new element/subarray")) -> (s? t:f=w616:string)
            n381 = Insert Into Array(array=w622, index=0, new element=w616) -> (w621:string[])
          }
          event "pb.Skip Step": Value Change {
            n382 = event-data() -> ()  [unwired: 1 in, 1 out]
            n383 = Bundle By Name(cluster=w626, "SkipStep"=TRUE) -> (w625:T15)
            n384 = Insert Into Array(array=w630, index=0, new element="Skip Step" ("new element/subarray")) -> (w629:string[])
          }
          event "Parameter 1": Value Change {
            n385 = event-data() -> ("OldVal"=w653:T3, "NewVal"=w652:T3)  [unwired: 1 in]
            n386 = Unbundle By Name(w649) -> ("Controller.Stop Command"=w651:dbl, "CommandCluster.SP3"=w650:dbl)
            n387 = case shown="Default" w653 {
              selector: w653 -> [w669 _]
              tunnel: [w686 w753] -> w640
              tunnel: [w685 w745] -> w641
              tunnel: [w684 w751] -> w642
              tunnel: [w683 w745] -> w643
              tunnel: w652 -> [_ w749]
              tunnel: [w675 w747] -> w647
              tunnel: [w674 w746] -> w646
              frame Default {
                n388 = property on="Parameter 1" class="Enum (strict)"() -> ("Disabled Items []"=w671:i32[])  [unwired: 2 in, 2 out]
                n389 = local read "Parameter 2"() -> (w688:enum16{"Voltage", "Pressure", "Flow", "Speed"})
                n390 = local read "Setpoint2"() -> (w678:dbl)
                n391 = Not Equal?(x=T3."Voltage" ("OldVal"), y=w669) -> (x != y?=w668:bool)
                n392 = case shown="\"Deadhead\"" "Parameter 1" {
                  selector: "Parameter 1" -> [w706 w714 w722 w730 w742]
                  tunnel: w688 -> [w705 w713 w721 w729 _]
                  tunnel: [FALSE w718 w726 w734 FALSE] -> w690
                  tunnel: 0.0 ("Setpoint1") -> [w707 w716 w724 w732 w736]
                  tunnel: [w709 w717 w725 w733 T17."Disabled and Grayed Out" ("Disabled")] -> w682
                  tunnel: T17."Enabled" ("Disabled") -> [w709 w717 w725 w733 _]
                  tunnel: [w707 w716 w724 w732 w736] -> w680
                  tunnel: [w708 w715 w723 w731 w735] -> w679
                  tunnel: w678 -> [w708 w715 w723 w731 _]
                  tunnel: [w706 w714 w722 w730 w742] -> w677
                  tunnel: [w705 w713 w721 w729 enum16{"Voltage", "Pressure", "Flow", "Speed"}."Voltage" ("Parameter2")] -> w676
                  tunnel: [w704 w712 w720 w728 w740] -> w673
                  tunnel: [w703 w711 w719 w727 i32[] [] ("Disabled Items []")] -> w672
                  tunnel: w671 -> [w703 w711 w719 w727 _]
                  tunnel: w668 -> [_ _ _ _ w738]
                  frame "Voltage", Default {
                    n393 = Build Array(w706) -> (w704:T26)
                  }
                  frame "Pressure" {
                    n394 = Greater?(x=w714, y=w713) -> (0:w718:bool)
                    n395 = Build Array(w714) -> (w712:T26)
                  }
                  frame "Flow" {
                    n396 = Greater?(x=w722, y=w721) -> (0:w726:bool)
                    n397 = Build Array(w722) -> (w720:T26)
                  }
                  frame "Speed" {
                    n398 = Greater?(x=w730, y=w729) -> (0:w734:bool)
                    n399 = Build Array(w730) -> (w728:T26)
                  }
                  frame "Deadhead" {
                    w740 = enum16{"Voltage", "Pressure", "Flow", "Speed"}[] [enum."Pressure", enum."Flow", enum."Speed"] items=["Voltage", "Pressure", "Flow", "Speed"]
                    # "should be an array\nof incoming para1"
                    n400 = local read "Setpoint1"() -> (w737:dbl)
                    n401 = Select(t=w736, s=w738, f=w737) -> (s? t:f=w735:dbl)
                  }
                }
                n402 = case shown="True" w690 {
                  tunnel: [w694 w701] -> w686
                  tunnel: [w693 w698] -> w684
                  tunnel: [w696 w702] -> w685
                  tunnel: [w695 w697] -> w683
                  tunnel: w680 -> [w696 w697]
                  tunnel: w679 -> [w695 w702]
                  tunnel: w677 -> [w694 w698]
                  tunnel: w676 -> [w693 w701]
                  tunnel: [w691 w700] -> w675
                  tunnel: [w692 w699] -> w674
                  tunnel: w673 -> [w692 w700]
                  tunnel: w672 -> [w691 w699]
                  frame False {
                    # "Parameters\nare in the\ncorrect order"
                  }
                  frame True {
                    # "Switch\nparameter\norder"
                  }
                }
                n403 = property on="Setpoint1" class="DigNum (strict)"("DisabledEnum"=w682) -> ()  [unwired: 2 in, 2 out]
              }
              frame "Deadhead" {
                w745 = 0.0 ("Setpoint1")
                n404 = Increment(x=w749) -> (x+1=w752:T3)
                n405 = Less Or Equal?(x=w752, y=T3."Speed") -> (x <= y?=w754:bool)
                n406 = case shown="True" w754 {
                  tunnel: w749 -> [w758 w762]
                  tunnel: [w757 w762] -> w753
                  tunnel: w749 -> [w759 w761]
                  tunnel: [w757 w761] -> w748
                  tunnel: w752 -> [_ w760]
                  tunnel: [w758 w760] -> w751
                  tunnel: [w759 w760] -> w750
                  frame False {
                    w757 = T3."Voltage" ("NewVal")
                  }
                  frame True {
                  }
                }
                n407 = property on="Setpoint1" class="DigNum (strict)"("DisabledEnum"=T17."Enabled" ("Disabled")) -> ()  [unwired: 2 in, 2 out]
                n408 = Build Array(w748) -> (w746:T26)
                n409 = Build Array(w750) -> (w747:T26)
              }
            }
            n410 = local read "pb.StartManual"() -> (w639:bool)
            n411 = case shown="True" w639 {
              tunnel: w638 -> [w658 w661]
              tunnel: [w658 w660] -> w637
              frame False {
              }
              frame True {
                n412 = Insert Into Array(array=w661, index=0, new element=string[] ["Write Command"]) -> (w660:string[])
              }
            }
            n413 = call "Handle Parameter 3 Control.vi"("Parameter 1"=w640, "Parameter 2"=w642, "Stop Command"=w651, "Last Command"=w650) -> ("Parameter 3"=w648:i32, "Command  Out"=w644:dbl)  [unwired: 9 in, 1 out]
            n414 = property on="Parameter 1" class="Enum (strict)"("Disabled Items []"=w647) -> ()  [unwired: 2 in, 2 out]
            n415 = property on="Parameter 2" class="Enum (strict)"("Disabled Items []"=w646) -> ()  [unwired: 2 in, 2 out]
            n416 = call "Set Parameter Controls.vi"("Para 1"=w640, "Para 2"=w642, "Para 3"=w648) -> ("Error Out"=w645:errorcluster)  [unwired: 12 in]
            n417 = property on="Steps" class="Ring (strict)"() -> ("Value"=w636:u16, "Visible"=w634:bool)  [unwired: 2 in, 2 out]
            n418 = flat-sequence {
              tunnel: w645 -> [_]
              tunnel: w644 -> [w667]
              tunnel: w643 -> [w666]
              tunnel: w642 -> [w665]
              tunnel: w641 -> [w664]
              tunnel: w640 -> [w663]
              frame #0 {
                n419 = local write "Parameter 1"(w663) -> ()
                n420 = local write "Setpoint1"(w664) -> ()
                n421 = local write "Parameter 2"(w665) -> ()
                n422 = local write "Setpoint2"(w666) -> ()
                n423 = local write "Setpoint3"(w667) -> ()
              }
            }
            n424 = Not Equal To 0?(x=w636) -> (x != 0?=w635:bool)
            n425 = And(x=w635, y=w634) -> (x .and. y?=w633:bool)
            n426 = Bundle By Name(cluster=w649, "CommandCluster.Para1"=w640, "CommandCluster.SP1"=w641, "CommandCluster.Para2"=w642, "CommandCluster.SP2"=w643, "CommandCluster.Para3"=w648, "CommandCluster.SP3"=w644) -> (w632:T15)
            n427 = case shown="False" w633 {
              tunnel: w632 -> [w656 w657]
              tunnel: [w655 w657] -> w631
              frame False {
                # "Not running a test\nstep so make:\nDesiredParameters\n= CommandCluster"
                n428 = Unbundle By Name(w656) -> ("CommandCluster"=w654:T6)
                n429 = Bundle By Name(cluster=w656, "DesiredParameters"=w654) -> (w655:T15)
              }
              frame True {
                # "Running a test step\nso do not change\nDesiredParameters"
              }
            }
          }
          event "Parameter 2": Value Change {
            n430 = event-data() -> ()  [unwired: 1 in, 1 out]
            n431 = Unbundle By Name(w783) -> ("Controller.Stop Command"=w781:dbl, "CommandCluster.SP3"=w782:dbl)
            n432 = local read "Parameter 1"() -> (w785:T3)
            n433 = Build Array("Parameter 2") -> (w778:enum16{"Voltage", "Pressure", "Flow", "Speed"}[])
            n434 = case shown="\"Voltage\"..\"Flow\", Default" "Parameter 2" {
              selector: "Parameter 2" -> [w813 _]
              tunnel: w785 -> [w814 _]
              tunnel: [w812 FALSE] -> w784
              frame "Voltage".."Flow", Default {
                n435 = Less?(x=w813, y=w814) -> (x < y?=w812:bool)
              }
              frame "Speed" {
              }
            }
            n436 = property on="Parameter 1" class="Enum (strict)"("Disabled Items []"=w778) -> ()  [unwired: 2 in, 2 out]
            n437 = local read "pb.StartManual"() -> (w771:bool)
            n438 = case shown="True" w784 {
              tunnel: [w803 w807] -> w775
              tunnel: [w802 w806] -> w776
              tunnel: [w801 0.0 ("Setpoint1")] -> w773
              tunnel: [0.0 ("Setpoint1") w805] -> w774
              frame False {
                # "Parameters in correct order"
                n439 = local read "Parameter 1"() -> (w803:T3)
                n440 = local read "Parameter 2"() -> (w802:enum16{"Voltage", "Pressure", "Flow", "Speed"})
                n441 = local read "Setpoint1"() -> (w801:dbl)
              }
              frame True {
                # "Switch"
                n442 = property on="Parameter 1" class="Enum (strict)"() -> ("Disabled Items []"=w809:i32[])  [unwired: 2 in, 2 out]
                n443 = property on="Parameter 2" class="Enum (strict)"() -> ("Disabled Items []"=w808:i32[])  [unwired: 2 in, 2 out]
                n444 = local read "Parameter 2"() -> (w807:enum16{"Voltage", "Pressure", "Flow", "Speed"})
                n445 = local read "Parameter 1"() -> (w806:T3)
                n446 = local read "Setpoint1"() -> (w805:dbl)
                n447 = flat-sequence {
                  tunnel: w808 -> [w811]
                  tunnel: w809 -> [w810]
                  frame #0 {
                    n448 = property on="Parameter 2" class="Enum (strict)"("Disabled Items []"=w810) -> ()  [unwired: 2 in, 2 out]
                    n449 = property on="Parameter 1" class="Enum (strict)"("Disabled Items []"=w811) -> ()  [unwired: 2 in, 2 out]
                  }
                }
              }
            }
            n450 = case shown="True" w771 {
              tunnel: w769 -> [w790 w793]
              tunnel: [w790 w792] -> w770
              frame False {
              }
              frame True {
                n451 = Insert Into Array(array=w793, index=0, new element=string[] ["Write Command"]) -> (w792:string[])
              }
            }
            n452 = call "Handle Parameter 3 Control.vi"("Parameter 1"=w775, "Parameter 2"=w776, "Stop Command"=w781, "Last Command"=w782) -> ("Parameter 3"=w779:i32, "Command  Out"=w780:dbl)  [unwired: 9 in, 1 out]
            n453 = call "Set Parameter Controls.vi"("Para 1"=w775, "Para 2"=w776, "Para 3"=w779) -> ("Error Out"=w772:errorcluster)  [unwired: 12 in]
            n454 = property on="Steps" class="Ring (strict)"() -> ("Value"=w768:u16, "Visible"=w766:bool)  [unwired: 2 in, 2 out]
            n455 = Not Equal To 0?(x=w768) -> (x != 0?=w767:bool)
            n456 = flat-sequence {
              tunnel: w780 -> [w799]
              tunnel: w776 -> [w798]
              tunnel: w775 -> [w797]
              tunnel: w774 -> [w796]
              tunnel: w773 -> [w795]
              tunnel: w772 -> [_]
              frame #0 {
                n457 = local write "Parameter 1"(w797) -> ()
                n458 = local write "Setpoint1"(w795) -> ()
                n459 = local write "Parameter 2"(w798) -> ()
                n460 = local write "Setpoint2"(w796) -> ()
                n461 = local write "Setpoint3"(w799) -> ()
              }
            }
            n462 = And(x=w767, y=w766) -> (x .and. y?=w765:bool)
            n463 = Bundle By Name(cluster=w783, "CommandCluster.Para1"=w775, "CommandCluster.SP1"=w773, "CommandCluster.Para2"=w776, "CommandCluster.SP2"=w774, "CommandCluster.Para3"=w779, "CommandCluster.SP3"=w780) -> (w764:T15)
            n464 = case shown="False" w765 {
              tunnel: w764 -> [w788 w789]
              tunnel: [w787 w789] -> w763
              frame False {
                # "Not running a test\nstep so make:\nDesiredParameters\n= CommandCluster"
                n465 = Unbundle By Name(w788) -> ("CommandCluster"=w786:T6)
                n466 = Bundle By Name(cluster=w788, "DesiredParameters"=w786) -> (w787:T15)
              }
              frame True {
                # "Running a test step\nso do not change\nDesiredParameters"
              }
            }
          }
          event "Parameter 3": Value Change {
            # "have to have the new\nmin/max values in before\nasserting new value"
            n467 = event-data() -> ()  [unwired: 1 in, 1 out]
            n468 = Unbundle By Name(w834) -> ("CommandCluster.Para1"=w825:i32, "CommandCluster.Para2"=w829:i32, "Controller.Stop Command"=w833:dbl)
            n469 = Equal?(x="Parameter 3", y=T2."Command") -> (x = y?=w830:bool)
            n470 = call "Set Parameter Controls.vi"("Para 1"=w825, "Para 2"=w829, "Para 3"="Parameter 3") -> ("Error Out"=w827:errorcluster)  [unwired: 12 in]
            n471 = local read "pb.StartManual"() -> (w822:bool)
            n472 = Select(t=w833, s=w830, f=0.0) -> (s? t:f=w831:dbl)
            n473 = flat-sequence {
              tunnel: w831 -> [w844]
              tunnel: w827 -> [_]
              frame #0 {
                n474 = local write "Setpoint3"(w844) -> ()
              }
            }
            n475 = case shown="True" w822 {
              tunnel: w824 -> [w839 w842]
              tunnel: [w839 w841] -> w823
              frame False {
              }
              frame True {
                n476 = Insert Into Array(array=w842, index=0, new element=string[] ["Write Command"]) -> (w841:string[])
              }
            }
            n477 = Bundle By Name(cluster=w834, "CommandCluster.Para3"="Parameter 3", "CommandCluster.SP3"=w831) -> (w817:T15)
            n478 = property on="Steps" class="Ring (strict)"() -> ("Value"=w821:u16, "Visible"=w819:bool)  [unwired: 2 in, 2 out]
            n479 = Not Equal To 0?(x=w821) -> (x != 0?=w820:bool)
            n480 = And(x=w820, y=w819) -> (x .and. y?=w818:bool)
            n481 = case shown="False" w818 {
              tunnel: w817 -> [w837 w838]
              tunnel: [w836 w838] -> w816
              frame False {
                # "Not running a test\nstep so make:\nDesiredParameters\n= CommandCluster"
                n482 = Unbundle By Name(w837) -> ("CommandCluster"=w835:T6)
                n483 = Bundle By Name(cluster=w837, "DesiredParameters"=w835) -> (w836:T15)
              }
              frame True {
                # "Running a test step\nso do not change\nDesiredParameters"
              }
            }
          }
          event "Setpoint1", "Setpoint2", "Setpoint3": Value Change {
            n484 = event-data() -> ()  [unwired: 1 in, 1 out]
            n485 = local read "Parameter 1"() -> (w865:T3)
            n486 = Equal?(x=w865, y=T3."Deadhead") -> (x = y?=w863:bool)
            n487 = Select(t=0.0, s=w863, f="Setpoint1") -> (s? t:f=w860:dbl)
            n488 = Bundle By Name(cluster=w859, "CommandCluster.SP1"=w860, "CommandCluster.SP2"="Setpoint2", "CommandCluster.SP3"="Setpoint3") -> (w847:T15)
            n489 = local read "pb.StartManual"() -> (w854:bool)
            n490 = property on="Steps" class="Ring (strict)"() -> ("Value"=w850:u16, "Visible"=w848:bool)  [unwired: 2 in, 2 out]
            n491 = Not Equal To 0?(x=w850) -> (x != 0?=w849:bool)
            n492 = And(x=w849, y=w848) -> (x .and. y?=w846:bool)
            n493 = case shown="False" w846 {
              tunnel: w847 -> [w869 w870]
              tunnel: [w868 w870] -> w845
              frame False {
                # "Not running a test\nstep so make:\nDesiredParameters\n= CommandCluster"
                n494 = Unbundle By Name(w869) -> ("CommandCluster"=w867:T6)
                n495 = Bundle By Name(cluster=w869, "DesiredParameters"=w867) -> (w868:T15)
              }
              frame True {
                # "Running a test step\nso do not change\nDesiredParameters"
              }
            }
            n496 = Select(t=string[] ["Apply Limits", "Write Command"], s=w854, f=string[] ["PS Abler", "Apply Limits"]) -> (s? t:f=w853:string[])
            n497 = Insert Into Array(array=w852, index=0, new element=w853) -> (w851:string[])
          }
          event "pb.auto-pop": Value Change {
            w872 = T17."Disabled and Grayed Out" ("Disabled")
            n498 = event-data() -> ()  [unwired: 1 in, 1 out]
            n499 = local write "Pump# Pages"(enum32{"SN", "Auto"}."Auto" ("Pump# Pages")) -> ()
            n500 = call "Test Config Enabler.vi"("Mode"=enum16{"Init", "Enable", "Disable", "AutoPop"}."AutoPop") -> ()  [unwired: 15 in]
            n501 = call "Tab Handler.vi"("Mode"=T21."Lock All") -> ()  [unwired: 15 in]
            n502 = property on="pb.new" class="Bool"("DisabledEnum"=w872) -> ()  [unwired: 2 in, 2 out]
            n503 = property on="pb.save" class="Bool"("DisabledEnum"=w872) -> ()  [unwired: 2 in, 2 out]
            n504 = property on="pb.load" class="Bool"("DisabledEnum"=w872) -> ()  [unwired: 2 in, 2 out]
            n505 = property on="pb.load profile" class="Bool"("DisabledEnum"=w872) -> ()  [unwired: 2 in, 2 out]
          }
          event "pb.auto-cancel": Value Change {
            w878 = T17."Enabled" ("Disabled")
            n506 = event-data() -> ()  [unwired: 1 in, 1 out]
            n507 = local write "Pump# Pages"(enum32{"SN", "Auto"}."SN" ("Pump# Pages")) -> ()
            n508 = call "Tab Handler.vi"("Mode"=T21."Test Config") -> ()  [unwired: 15 in]
            n509 = property on="pb.new" class="Bool"("DisabledEnum"=w878) -> ()  [unwired: 2 in, 2 out]
            n510 = property on="pb.save" class="Bool"("DisabledEnum"=w878) -> ()  [unwired: 2 in, 2 out]
            n511 = property on="pb.load" class="Bool"("DisabledEnum"=w878) -> ()  [unwired: 2 in, 2 out]
            n512 = property on="pb.load profile" class="Bool"("DisabledEnum"=w878) -> ()  [unwired: 2 in, 2 out]
            n513 = call "Test Config Enabler.vi"("Mode"=enum16{"Init", "Enable", "Disable", "AutoPop"}."Enable") -> ()  [unwired: 15 in]
          }
          event "Starting Serial Number", "Serial Number Step", "Ending Serial Number": Value Change {
            n514 = event-data() -> ()  [unwired: 1 in, 1 out]
            n515 = call "Valid AutoPopulate.vi"("Starting Serial Number"="Ending Serial Number", "Ending Serial Number"="Starting Serial Number", "Serial Number Step"="Serial Number Step") -> ("Valid?"=w883:bool)  [unwired: 12 in]
            n516 = case shown="False" w883 {
              frame False {
                n517 = property on="pb.auto-confirm" class="Bool"("DisabledEnum"=T17."Disabled and Grayed Out" ("Disabled")) -> ()  [unwired: 2 in, 2 out]
              }
              frame True {
                n518 = property on="pb.auto-confirm" class="Bool"("DisabledEnum"=T17."Enabled" ("Disabled")) -> ()  [unwired: 2 in, 2 out]
              }
            }
          }
          event "pb.auto-confirm": Value Change {
            n519 = event-data() -> ()  [unwired: 1 in, 1 out]
            n520 = local read "Starting Serial Number"() -> (w892:u32)
            n521 = local read "Ending Serial Number"() -> (w894:u32)
            n522 = local read "Serial Number Step"() -> (w896:u32)
            n523 = To Long Integer(number=w892) -> (32bit integer=w891:i32)
            n524 = To Long Integer(number=w894) -> (32bit integer=w893:i32)
            n525 = To Long Integer(number=w896) -> (32bit integer=w895:i32)
            n526 = call "Valid AutoPopulate.vi"("Starting Serial Number"=w894, "Ending Serial Number"=w892, "Serial Number Step"=w896) -> ("Valid?"=w898:bool)  [unwired: 12 in]
            n527 = case shown="True" w898 {
              tunnel: w895 -> [_ w917]
              tunnel: w893 -> [_ w915]
              tunnel: w891 -> [_ w914]
              tunnel: [w901 w913] -> w899
              tunnel: w897 -> [w901 w905]
              frame False {
                n528 = property on="pb.auto-confirm" class="Bool"("DisabledEnum"=T17."Disabled and Grayed Out" ("Disabled")) -> ()  [unwired: 2 in, 2 out]
              }
              frame True {
                n529 = Less?(x=w914, y=w915) -> (x < y?=w916:bool)
                n530 = while {
                  shift-right: [w933] -> _
                  shift-left: w914 -> [w937]
                  tunnel: w917 -> [w936]
                  tunnel: w915 -> [w934]
                  tunnel: w916 -> [w935]
                  tunnel: [w932] -> w909 mode=indexing
                  tunnel: [w930] -> w910
                  stop <- w931 stop-if-true
                  n531 = case shown="False" w935 {
                    tunnel: w937 -> [w943 w949]
                    tunnel: w936 -> [w942 w948]
                    tunnel: [w939 w946] -> w933
                    tunnel: w934 -> [w938 w945]
                    tunnel: [w941 w947] -> w931
                    tunnel: [w940 w944] -> w930
                    frame False {
                      n532 = Subtract(x=w943, y=w942) -> (x-y=w939:i32)
                      n533 = Less Or Equal?(x=w939, y=w938) -> (x <= y?=w941:bool)
                      n534 = Equal?(x=w939, y=w938) -> (x = y?=w940:bool)
                    }
                    frame True {
                      n535 = Add(x=w949, y=w948) -> (x+y=w946:i32)
                      n536 = Greater Or Equal?(x=w946, y=w945) -> (x >= y?=w947:bool)
                      n537 = Equal?(x=w946, y=w945) -> (x = y?=w944:bool)
                    }
                  }
                  n538 = Number To Decimal String(number=w933) -> (decimal integer string=w932:string)  [unwired: 1 in]
                }
                n539 = Unbundle By Name(w905) -> ("ValidFile?"=w906:bool)
                n540 = property on="pb.auto-confirm" class="Bool"("DisabledEnum"=T17."Enabled" ("Disabled")) -> ()  [unwired: 2 in, 2 out]
                n541 = case shown="True" w906 {
                  frame False {
                  }
                  frame True {
                    n542 = property on="pb.save" class="Bool"("DisabledEnum"=T17."Enabled" ("Disabled")) -> ()  [unwired: 2 in, 2 out]
                  }
                }
                n543 = Number To Decimal String(number=w914) -> (decimal integer string=w918:string)  [unwired: 1 in]
                n544 = case shown="False" w910 {
                  tunnel: w909 -> [w922 w923]
                  tunnel: [w921 w923] -> w908
                  frame False {
                    n545 = Delete From Array(array=w922) -> (array with subset deleted=w921:string[])  [unwired: 2 in, 1 out]
                  }
                  frame True {
                  }
                }
                n546 = Insert Into Array(array=w908, index=0, new element=w918) -> (w904:string[])
                n547 = call "SN Sort.vi"("Array In"=w904) -> ("Array Out"=w903:string[])  [unwired: 14 in]
                n548 = Bundle By Name(cluster=w905, "Serial Numbers"=w903) -> (w913:T15)
                n549 = Build Array(w903) -> (w912:string[][])
                n550 = Transpose 2D Array(2D array=w912) -> (transposed array=w911:string[][])
                n551 = stacked-sequence {
                  tunnel: w911 -> [w924 _]
                  frame #0 {
                    n552 = local write "Serial Numbers"(w924) -> ()
                  }
                  frame #1 {
                    w926 = T17."Enabled" ("Disabled")
                    n553 = local write "Pump# Pages"(enum32{"SN", "Auto"}."SN" ("Pump# Pages")) -> ()
                    n554 = property on="pb.new" class="Bool"("DisabledEnum"=w926) -> ()  [unwired: 2 in, 2 out]
                    n555 = property on="pb.save" class="Bool"("DisabledEnum"=w926) -> ()  [unwired: 2 in, 2 out]
                    n556 = property on="pb.load" class="Bool"("DisabledEnum"=w926) -> ()  [unwired: 2 in, 2 out]
                    n557 = property on="pb.load profile" class="Bool"("DisabledEnum"=w926) -> ()  [unwired: 2 in, 2 out]
                    n558 = property on="Serial Numbers" class="Tbl (strict)"("Index Values"=T16 {"Row"=0, "Column"=0}) -> ()  [unwired: 2 in, 2 out]
                    n559 = call "Tab Handler.vi"("Mode"=T21."Test Config") -> ()  [unwired: 15 in]
                    n560 = call "Test Config Enabler.vi"("Mode"=enum16{"Init", "Enable", "Disable", "AutoPop"}."Enable") -> ()  [unwired: 15 in]
                  }
                }
              }
            }
          }
          event "table.Data": Mouse Up {
            # "If the click was in the scrollbar ignore\nif it was not handle selecting the correct row"
            n561 = event-data() -> ("Coords.Horizontal"=w955:i32, "Coords.Vertical"=w954:i32)  [unwired: 1 in]
            n562 = In Range and Coerce(upper limit=-640, x=w955, lower limit=-657) -> (In Range?=w953:bool)  [unwired: 1 out]
            n563 = In Range and Coerce(upper limit=-337, x=w954, lower limit=-599) -> (In Range?=w952:bool)  [unwired: 1 out]
            n564 = And(x=w953, y=w952) -> (x .and. y?=w950:bool)
            n565 = case shown="False" w950 {
              tunnel: w961 -> [w962 w966]
              tunnel: [w962 w963] -> w960
              frame True {
              }
              frame False {
                n566 = Insert Into Array(array=w966, index=0, new element=string[] ["Data Table Mouse Up"]) -> (w963:string[])
              }
            }
          }
          event "table.Stats": Mouse Up {
            # "If the click was in the\nscrollbar, ignore it. If it\nwas not, handle selecting\nthe correct row"
            n567 = event-data() -> ("Coords.Horizontal"=w970:i32, "Coords.Vertical"=w969:i32)  [unwired: 1 in]
            n568 = In Range and Coerce(upper limit=-640, x=w970, lower limit=-657) -> (In Range?=w972:bool)  [unwired: 1 out]
            n569 = In Range and Coerce(upper limit=-337, x=w969, lower limit=-599) -> (In Range?=w971:bool)  [unwired: 1 out]
            n570 = And(x=w972, y=w971) -> (x .and. y?=w968:bool)
            n571 = case shown="False" w968 {
              tunnel: w967 -> [_ w979]
              frame True {
              }
              frame False {
                n572 = Unbundle By Name(w979) -> ("table.Data"=w981:string[][], "table.Stats"=w982:string[][])
                n573 = property on="table.Stats" class="Tbl (strict)"() -> ("Selection Start"=w980:T19)  [unwired: 2 in, 2 out]
                n574 = Unbundle(w980) -> ("Row"=w978:i32)  [unwired: 1 out]
                n575 = call "Full Table Handler.vi"("table.Data"=w981, "table.Stats"=w982, "Stat Row Index"=w978) -> ()  [unwired: 13 in]
              }
            }
          }
          event "table.Data": Mouse Down? {
            n576 = event-data() -> ("Button"=w991:u16)  [unwired: 1 in]
            n577 = Unbundle By Name(w986) -> ("TestRunning?"=w985:bool)
            n578 = Equal?(x=w991, y=u16 2) -> (x = y?=w984:bool)
            n579 = Compound Arithmetic op=AND(invert w985, w984) -> (w983:bool)
            n580 = case shown="True" w983 {
              tunnel: w988 -> [w994 w1003]
              tunnel: [w993 w1003] -> w987
              frame True {
                # "Right-Click"
                n581 = Two Button Dialog(message="Delete highlighted row?", 1:"No" ("F button name (\"Cancel\")"), 2:"Yes" ("T button name (\"OK\")")) -> (T button?=w992:bool)
                n582 = case shown="True" w992 {
                  tunnel: w994 -> [w998 w1002]
                  tunnel: [w998 w1001] -> w993
                  frame False {
                  }
                  frame True {
                    n583 = Insert Into Array(array=w1002, index=0, new element="Delete Data Row" ("new element/subarray")) -> (w1001:string[])
                  }
                }
              }
              frame False {
                # "Left-Click handled by mouse up event"
              }
            }
            n584 = event-data("Discard?"=FALSE) -> ()  [unwired: 1 in, 1 out]
          }
          event "table.Stats": Mouse Down? {
            n585 = event-data() -> ("Button"=w1012:u16)  [unwired: 1 in]
            n586 = Unbundle By Name(w1005) -> ("TestRunning?"=w1007:bool)
            n587 = Equal?(x=w1012, y=u16 2) -> (x = y?=w1006:bool)
            n588 = Compound Arithmetic op=AND(invert w1007, w1006) -> (w1004:bool)
            n589 = case shown="True" w1004 {
              tunnel: w1009 -> [w1015 w1024]
              tunnel: [w1014 w1024] -> w1008
              frame True {
                # "Right-Click"
                n590 = Two Button Dialog(message="Delete highlighted row?", 1:"No" ("F button name (\"Cancel\")"), 2:"Yes" ("T button name (\"OK\")")) -> (T button?=w1013:bool)
                n591 = case shown="True" w1013 {
                  tunnel: w1015 -> [w1019 w1023]
                  tunnel: [w1019 w1022] -> w1014
                  frame False {
                  }
                  frame True {
                    n592 = Insert Into Array(array=w1023, index=0, new element="Delete Stat Row" ("new element/subarray")) -> (w1022:string[])
                  }
                }
              }
              frame False {
                # "Left-Click handled by mouse up event"
              }
            }
            n593 = event-data("Discard?"=FALSE) -> ()  [unwired: 1 in, 1 out]
          }
          event "table.Data": Value Change {
            # "The only situation where this event occurs is if\nsomeone tries to change a serial number but\ncannot disable this control or I lose my insert\nand delete functionality"
            n594 = event-data() -> ()  [unwired: 1 in, 1 out]
            n595 = Unbundle By Name(w1026) -> ("table.Data"=w1027:string[][])
            n596 = local write "table.Data"(w1027) -> ()
          }
          event "table.Stats": Value Change {
            # "The only situation where this event occurs is if\nsomeone tries to change a serial number but\ncannot disable this control or I lose my insert\nand delete functionality"
            n597 = event-data() -> ()  [unwired: 1 in, 1 out]
            n598 = Unbundle By Name(w1029) -> ("table.Stats"=w1030:string[][])
            n599 = local write "table.Stats"(w1030) -> ()
          }
          event "IP Address": Value Change {
            n600 = event-data() -> ("NewVal"=w1035:string)  [unwired: 1 in]
            n601 = String Length(string=w1035) -> (length=w1047:i32)
            n602 = Search and Replace String(replace all?=TRUE ("replace all? (F)"), input string=w1035, search string=".") -> (number of replacements=w1041:i32)  [unwired: 5 in, 3 out]
            n603 = In Range and Coerce(upper limit=15, x=w1047, lower limit=7) -> (In Range?=w1042:bool)  [unwired: 1 out]
            n604 = Equal?(x=w1041, y=3) -> (x = y?=w1039:bool)
            n605 = And(x=w1039, y=w1042) -> (x .and. y?=w1038:bool)
            n606 = case shown="True" w1038 {
              tunnel: w1035 -> [_ w1050]
              frame False {
              }
              frame True {
                n607 = Current VI's Path() -> (path=w1054:path)
                n608 = Strip Path(path=w1054) -> (stripped path=w1053:path)  [unwired: 1 out]
                n609 = Build Path(base path=w1053, name or relative path="IP.ini") -> (appended path=w1051:path)
                n610 = call <vilib>:"Open Config Data.vi"("configuration file path"=w1051) -> ("error out"=w1057:errorcluster, "refnum"=w1055:T27)  [unwired: 8 in, 1 out]
                n611 = call-poly <vilib>:"Write Key.vi"("section"="IP", "error in (no error)"=w1057, "value"=w1050, "key"="IP Address", "refnum"=w1055) -> ("error out"=w1048:errorcluster, "refnum out"=w1049:T27)  [unwired: 4 in, 1 out]
                n612 = local write "IP Address"(w1050) -> ()
                n613 = local write "IP Address 2"(w1050) -> ()
                n614 = call <vilib>:"Close Config Data.vi"("error in (no error)"=w1048, "refnum"=w1049) -> ()  [unwired: 8 in, 2 out]
              }
            }
            n615 = Bundle By Name(cluster=w1037, "IP Address"=w1035) -> (w1036:T15)
            n616 = Insert Into Array(array=w1032, index=0, new element="Save Config") -> (w1031:string[])
          }
          event "Max Voltage", "Voltage Tolerance", "Max Current", "Max Pressure", "Pressure Tolerance", "Min Flow", "Max Flow", "Flow Tolerance", "Speed Tolerance", "Parameter Timeout (sec)", "Stable Count (sec)", "Init Free Flow (sec)", "Free Flow Voltage", "Free Flow Pressure", "Gauge Number": Value Change {
            w1088 = T5 {"Voltage Tolerances"=0.0, "Pressure Tolerances"=0.0, "Flow Tolerances"=0.0, "Speed Tolerances"=0.0, "Stable Count (sec)"=0.0}  # Stability Cluster
            n617 = event-data() -> ()  [unwired: 1 in, 1 out]
            n618 = call "Remove Tildes (String).vi"("String In"="Gauge Number") -> ("String Out"=w1080:string)  [unwired: 2 in]
            n619 = Build Array("Max Voltage", "Max Pressure") -> (w1070:dbl[])
            n620 = Bundle By Name(cluster=w1108, "StandConfigCluster.Max Voltage"="Max Voltage", "StandConfigCluster.Voltage Tolerance"="Voltage Tolerance", "StandConfigCluster.Max Current"="Max Current", "StandConfigCluster.Max Pressure"="Max Pressure", "StandConfigCluster.Pressure Tolerance"="Pressure Tolerance", "StandConfigCluster.Min Flow"="Min Flow", "StandConfigCluster.Max Flow"="Max Flow", "StandConfigCluster.Flow Tolerance"="Flow Tolerance", "StandConfigCluster.Speed Tolerance"="Speed Tolerance", "StandConfigCluster.Stable Count"="Stable Count (sec)", "StandConfigCluster.Parameter Timeout"="Parameter Timeout (sec)", "StandConfigCluster.Init Free Flow"="Init Free Flow (sec)", "StandConfigCluster.Free Flow Voltage"="Free Flow Voltage", "StandConfigCluster.Free Flow Pressure"="Free Flow Pressure", "Gauge Number"=w1080) -> (w1064:T15)
            n621 = Flatten To String(anything=w1070) -> (data string=w1079:string, error out=w1068:errorcluster)  [unwired: 3 in, 1 out]
            n622 = Bundle(cluster=T22 {"Command"="", "FlattenedData"=""}, "Command"="VPLimits", "FlattenedData"=w1079) -> (w1077:T22)
            n623 = Flatten To String(anything=w1077, error in (no error)=w1068) -> (data string=w1073:string, error out=w1072:errorcluster)  [unwired: 2 in, 1 out]
            n624 = Unbundle By Name(w1064) -> ("StandConfigCluster"=w1083:T14, "Controller"=w1082:T10)
            n625 = call "PC Send Event.vi"("PC Send Command"=PCsend_RTrecv_CMD."VPLimits", "Mode"=Event_Mode."Set", "Flattened Data"=w1073, "Error In"=w1072) -> ("Error Out"=w1067:errorcluster)  [unwired: 10 in, 1 out]
            n626 = Bundle By Name(cluster=w1088, "Voltage Tolerances"="Voltage Tolerance", "Pressure Tolerances"="Pressure Tolerance", "Flow Tolerances"="Flow Tolerance", "Speed Tolerances"="Speed Tolerance", "Stable Count (sec)"="Stable Count (sec)") -> (w1062:T5)
            n627 = Add(x="Stable Count (sec)", y=2.0) -> (x+y=w1060:dbl)
            n628 = Insert Into Array(array=w1100, index=0, new element="Save Config") -> (w1099:string[])
            n629 = property on="Parameter Timeout (sec)" class="DigNum (strict)"("Minimum"=w1060) -> ()  [unwired: 2 in, 2 out]
            n630 = Bundle By Name(cluster=w1064, "Stability Cluster"=w1062) -> (w1063:T15)
            n631 = Flatten To String(anything=w1062, error in (no error)=w1067) -> (data string=w1091:string, error out=w1066:errorcluster)  [unwired: 2 in, 1 out]
            n632 = Bundle(cluster=T22 {"Command"="", "FlattenedData"=""}, "Command"="Tolerances", "FlattenedData"=w1091) -> (w1093:T22)
            n633 = call "Set Parameter Controls.vi"("Controls Mode (Set)"=Parameter_Controls_Mode."Update Ranges", "StandConfigCluster"=w1083, "Controller"=w1082) -> ()  [unwired: 12 in, 1 out]
            n634 = Flatten To String(anything=w1093, error in (no error)=w1066) -> (data string=w1094:string, error out=w1065:errorcluster)  [unwired: 2 in, 1 out]
            n635 = call "PC Send Event.vi"("PC Send Command"=PCsend_RTrecv_CMD."Tolerances", "Mode"=Event_Mode."Set", "Flattened Data"=w1094, "Error In"=w1065) -> ()  [unwired: 10 in, 2 out]
          }
          event "pb.select SN": Value Change {
            n636 = event-data() -> ()  [unwired: 1 in, 1 out]
            n637 = Insert Into Array(array=w1112, index=0, new element="Part Change" ("new element/subarray")) -> (w1111:string[])
          }
          event "Next Serial Number": Key Down {
            n638 = event-data() -> ("VKey"=w1114:T28)  [unwired: 1 in]
            n639 = case shown="\"Enter\", \"Return\"" w1114 {
              tunnel: w1116 -> [w1118 w1120]
              tunnel: [w1118 w1119] -> w1115
              frame Default {
              }
              frame "Enter", "Return" {
                n640 = Insert Into Array(array=w1120, index=0, new element="Part Change" ("new element/subarray")) -> (w1119:string[])
              }
            }
          }
          event "pb.test cancel": Value Change {
            n641 = event-data() -> ()  [unwired: 1 in, 1 out]
            n642 = Unbundle By Name(w1126) -> ("TestRunning?"=w1129:bool)
            n643 = case shown="True" w1129 {
              tunnel: w1128 -> [w1131 w1139]
              tunnel: [w1131 w1138] -> w1127
              tunnel: w1126 -> [w1130 w1135]
              tunnel: [w1130 w1134] -> w1125
              frame False {
              }
              frame True {
                w1133 = FALSE ("pb.StartTest")
                n644 = local write "Tab.Buttons"(enum32{"Manual", "Test"}."Manual" ("Tab.Buttons")) -> ()
                n645 = local write "pb.StartTest"(w1133) -> ()
                n646 = Insert Into Array(array=w1139, index=0, new element=string[] ["Stop Test"]) -> (w1138:string[])
                n647 = Bundle By Name(cluster=w1135, "TestRunning?"=w1133) -> (w1134:T15)
                n648 = local write "Running?"(w1133) -> ()
              }
            }
            n649 = call "Tab Handler.vi"("Mode"=T21."Run Screen") -> ()  [unwired: 15 in]
            n650 = local write "Screen"(T1."Run Screen" ("Screen")) -> ()
          }
          event Value Change {
            w1140 = 4 ("DesiredParameters.Para3")
            w1151 = Event_Mode."Set" ("Mode")
            # "Eval Parameters was added so that if there is data in\nthe command row of the profile it will be deleted\nwhen changing from controller to no controller"
            n651 = event-data() -> ()  [unwired: 1 in, 1 out]
            n652 = Unbundle By Name(w1177) -> ("Controller List"=w1161:T9, "ValidFile?"=w1166:bool, "StandConfigCluster"=w1164:T14)
            n653 = Index Array(array=w1161, index="Pump Control Style") -> (element=w1163:T10)
            n654 = case shown="True" w1166 {
              frame False {
              }
              frame True {
                n655 = property on="pb.save" class="Bool"("DisabledEnum"=T17."Enabled" ("Disabled")) -> ()  [unwired: 2 in, 2 out]
              }
            }
            n656 = Unbundle By Name(w1163) -> ("Stop Command"=w1168:dbl, "Controller Name"=w1179:T4, "Controller?"=w1144:bool)
            n657 = To Long Integer(number=w1179) -> (32bit integer=w1178:i32)
            n658 = Flatten To String(anything=w1178) -> (data string=w1180:string, error out=w1174:errorcluster)  [unwired: 3 in, 1 out]
            n659 = Not(x=w1144) -> (.not. x?=w1143:bool)
            n660 = Bundle(cluster=T22 {"Command"="", "FlattenedData"=""}, "Command"="Controller", "FlattenedData"=w1180) -> (w1182:T22)
            n661 = Flatten To String(anything=w1182, error in (no error)=w1174) -> (data string=w1184:string, error out=w1173:errorcluster)  [unwired: 2 in, 1 out]
            n662 = Select(t=w1168, s=w1144, f=nan) -> (s? t:f=w1141:dbl)
            n663 = call "PC Send Event.vi"("PC Send Command"=PCsend_RTrecv_CMD."Controller", "Mode"=w1151, "Flattened Data"=w1184, "Error In"=w1173) -> ("Error Out"=w1152:errorcluster)  [unwired: 10 in, 1 out]
            n664 = Select(t="Pump Current\n(A RMS)" ("Caption.Text"), s=w1144, f="Pump Current\n(A)" ("Caption.Text")) -> (s? t:f=w1145:string)
            n665 = Select(t="Pump\nVoltage (V)", s=w1143, f="Controller\nVoltage (V)") -> (s? t:f=w1170:string)
            n666 = local read "FFTwindowMax"() -> (w1150:u16)
            n667 = local read "FFTwindowMin"() -> (w1149:u16)
            n668 = property on="PumpCurrent(Arms)" class="DigNum (strict)"("Caption.Text"=w1145) -> ()  [unwired: 2 in, 2 out]
            n669 = property on="Voltage (DC)" class="DigNum (strict)"("Caption.Text"=w1170) -> ()  [unwired: 2 in, 2 out]
            n670 = Insert Into Array(array=w1142, index=0, new element=string[] ["Write Command", "PS Abler", "Alter Run Screen", "Alter Parameter Setup", "Eval Parameters"]) -> (w1169:string[])
            n671 = call "Set Parameter Controls.vi"("Controls Mode (Set)"=Parameter_Controls_Mode."Update Ranges", "StandConfigCluster"=w1164, "Controller"=w1163) -> ("Error Out"=w1162:errorcluster)  [unwired: 12 in]
            n672 = Bundle("FFTwindowMin"=w1149, "FFTwindowMax"=w1150) -> (w1148:cluster{"FFTwindowMin":u16, "FFTwindowMax":u16})  [unwired: 1 in]
            n673 = Flatten To String(anything=w1148, error in (no error)=w1152) -> (data string=w1160:string, error out=w1153:errorcluster)  [unwired: 2 in, 1 out]
            n674 = Bundle(cluster=T22 {"Command"="", "FlattenedData"=""}, "Command"="SpeedWindow", "FlattenedData"=w1160) -> (w1158:T22)
            n675 = flat-sequence {
              tunnel: w1141 -> [w1189]
              tunnel: w1162 -> [_]
              tunnel: w1140 -> [w1188]
              frame #0 {
                n676 = local write "Parameter 3"(w1188) -> ()
                n677 = local write "Setpoint3"(w1189) -> ()
              }
            }
            n678 = Flatten To String(anything=w1158, error in (no error)=w1153) -> (data string=w1155:string, error out=w1154:errorcluster)  [unwired: 2 in, 1 out]
            n679 = Bundle By Name(cluster=w1177, "CommandCluster.Para3"=w1140, "DesiredParameters.Para3"=w1140, "DesiredParameters.SP3"=w1141, "CommandCluster.SP3"=w1141, "Controller"=w1163, "TestCfgCluster.Pump Control Style"=w1179) -> (w1165:T15)
            n680 = call "PC Send Event.vi"("PC Send Command"=PCsend_RTrecv_CMD."SpeedWindow", "Mode"=w1151, "Flattened Data"=w1155, "Error In"=w1154) -> ()  [unwired: 10 in, 2 out]
          }
          event "Technician Name", "Shop Order Number", "Customer", "Platform", "Flow Test Fluid", "Fuel Batch Number", "CA Number", "Durability Tank Number", "Durability Fluid", "Hours Completed", "Pump Model": Value Change {
            n681 = event-data() -> ()  [unwired: 1 in, 1 out]
            n682 = Unbundle By Name(w1213) -> ("ValidFile?"=w1214:bool)
            n683 = case shown="True" w1214 {
              frame False {
              }
              frame True {
                n684 = property on="pb.save" class="Bool"("DisabledEnum"=T17."Enabled" ("Disabled")) -> ()  [unwired: 2 in, 2 out]
              }
            }
            n685 = call "Remove Tildes (String).vi"("String In"="Technician Name") -> ("String Out"=w1201:string)  [unwired: 2 in]
            n686 = call "Remove Tildes (String).vi"("String In"="Shop Order Number") -> ("String Out"=w1200:string)  [unwired: 2 in]
            n687 = call "Remove Tildes (String).vi"("String In"="Customer") -> ("String Out"=w1199:string)  [unwired: 2 in]
            n688 = call "Remove Tildes (String).vi"("String In"="Platform") -> ("String Out"=w1198:string)  [unwired: 2 in]
            n689 = call "Remove Tildes (String).vi"("String In"="Flow Test Fluid") -> ("String Out"=w1197:string)  [unwired: 2 in]
            n690 = call "Remove Tildes (String).vi"("String In"="Fuel Batch Number") -> ("String Out"=w1196:string)  [unwired: 2 in]
            n691 = call "Remove Tildes (String).vi"("String In"="CA Number") -> ("String Out"=w1195:string)  [unwired: 2 in]
            n692 = call "Remove Tildes (String).vi"("String In"="Durability Tank Number") -> ("String Out"=w1194:string)  [unwired: 2 in]
            n693 = call "Remove Tildes (String).vi"("String In"="Durability Fluid") -> ("String Out"=w1193:string)  [unwired: 2 in]
            n694 = call "Remove Tildes (String).vi"("String In"="Hours Completed") -> ("String Out"=w1192:string)  [unwired: 2 in]
            n695 = call "Remove Tildes (String).vi"("String In"="Pump Model") -> ("String Out"=w1191:string)  [unwired: 2 in]
            n696 = Bundle By Name(cluster=w1213, "TestCfgCluster.Technician Name"=w1201, "TestCfgCluster.Shop Order Number"=w1200, "TestCfgCluster.Customer"=w1199, "TestCfgCluster.Platform"=w1198, "TestCfgCluster.Flow Test Fluid"=w1197, "TestCfgCluster.Fuel Batch #"=w1196, "TestCfgCluster.CA Number"=w1195, "TestCfgCluster.Durability Tank #"=w1194, "TestCfgCluster.Durability Fluid"=w1193, "TestCfgCluster.Hours Completed"=w1192, "TestCfgCluster.Pump Model"=w1191) -> (w1216:T15)
          }
          event "Serial Number": Mouse Down {
            n697 = event-data() -> ("Mods.Double Click"=w1218:bool)  [unwired: 1 in]
            n698 = case shown="True" w1218 {
              frame False {
              }
              frame True {
                n699 = property on="pb.select SN" class="Bool"("Key Focus"=TRUE) -> ()  [unwired: 2 in, 2 out]
                n700 = call "Tab Handler.vi"("Mode"=T21."Other Tab") -> ()  [unwired: 15 in]
                n701 = local write "Screen"(T1."Part Change" ("Screen")) -> ()
              }
            }
          }
          event "Serial Number": Value Change {
            n702 = event-data() -> ()  [unwired: 1 in, 1 out]
            n703 = local read "Serial Number"() -> (w1225:string)
            n704 = call "Remove Tildes (String).vi"("String In"=w1225) -> ("String Out"=w1224:string)  [unwired: 2 in]
            n705 = Bundle By Name(cluster=w1228, "Serial Number"=w1224) -> (w1227:T15)
          }
          event "Serial Numbers": Key Down? {
            n706 = event-data() -> ("CtlRef"=w1236:refnum<vi>, "Char"=w1235:i16, "VKey"=w1234:T28, "ScanCode"=w1233:i16)  [unwired: 1 in]
            n707 = call "TableControl_1Column.vi"("CtlRef"=w1236, "CharIn"=w1235, "VKey"=w1234, "ScanCode"=w1233) -> ("CharOut"=w1232:i16, "Discard?"=w1231:bool)  [unwired: 10 in]
            n708 = event-data("Char"=w1232, "Discard?"=w1231) -> ()  [unwired: 1 in, 1 out]
          }
          event "Serial Numbers": Value Change {
            n709 = event-data() -> ()  [unwired: 1 in, 1 out]
            n710 = Unbundle By Name(w1238) -> ("ValidFile?"=w1244:bool)
            n711 = Index Array(array="Serial Numbers", index (col)=0 ("disabled index (col)")) -> (element=w1243:string[])  [unwired: 1 in]
            n712 = case shown="True" w1244 {
              frame False {
              }
              frame True {
                n713 = property on="pb.save" class="Bool"("DisabledEnum"=T17."Enabled" ("Disabled")) -> ()  [unwired: 2 in, 2 out]
              }
            }
            n714 = call "Remove Tildes (Array).vi"("String In"=w1243) -> ("String Out"=w1242:string[])  [unwired: 2 in]
            n715 = call "Remove Duplicates.vi"("Array In"=w1242) -> ("Array Out"=w1241:string[])  [unwired: 2 in]
            n716 = Build Array(w1241) -> (w1240:string[][])
            n717 = Transpose 2D Array(2D array=w1240) -> (transposed array=w1239:string[][])
            n718 = Bundle By Name(cluster=w1238, "Serial Numbers"=w1241) -> (w1237:T15)
            n719 = local write "Serial Numbers"(w1239) -> ()
          }
          event "Untested Serial Numbers": Mouse Down {
            n720 = event-data() -> ()  [unwired: 1 in, 1 out]
            n721 = flat-sequence {
              tunnel: [w1254] -> w1249
              frame #0 {
                n722 = local read "Untested Serial Numbers"() -> (w1257:string[][])
                n723 = local read "Next Serial Number"() -> (w1253:string)
                n724 = property on="Untested Serial Numbers" class="Tbl (strict)"() -> ("EditPos"=w1260:T19)  [unwired: 2 in, 2 out]
                n725 = Unbundle By Name(w1260) -> ("Row"=w1258:i32)
                n726 = call "Remove Tildes (String).vi"("String In"=w1253) -> ("String Out"=w1252:string)  [unwired: 2 in]
                n727 = Index Array(array=w1257, index (row)=w1258, index (col)=0 ("disabled index (col)")) -> (element=w1255:string)
                n728 = Empty String/Path?(string/path=w1255) -> (empty?=w1256:bool)
                n729 = Select(t=w1252, s=w1256, f=w1255) -> (s? t:f=w1254:string)
              }
            }
            n730 = local write "Next Serial Number"(w1249) -> ()
          }
          event "Tested Serial Numbers": Mouse Down {
            n731 = event-data() -> ()  [unwired: 1 in, 1 out]
            n732 = local read "Tested Serial Numbers"() -> (w1266:string[][])
            n733 = local read "Next Serial Number"() -> (w1262:string)
            n734 = property on="Tested Serial Numbers" class="Tbl (strict)"() -> ("EditPos"=w1267:T19)  [unwired: 2 in, 2 out]
            n735 = Unbundle By Name(w1267) -> ("Row"=w1270:i32)
            n736 = call "Remove Tildes (String).vi"("String In"=w1262) -> ("String Out"=w1261:string)  [unwired: 2 in]
            n737 = Index Array(array=w1266, index (row)=w1270, index (col)=0 ("disabled index (col)")) -> (element=w1268:string)
            n738 = Empty String/Path?(string/path=w1268) -> (empty?=w1269:bool)
            n739 = Select(t=w1261, s=w1269, f=w1268) -> (s? t:f=w1265:string)
            n740 = local write "Next Serial Number"(w1265) -> ()
          }
          event "Notes": Value Change {
            n741 = event-data() -> ()  [unwired: 1 in, 1 out]
            n742 = Unbundle By Name(w1277) -> ("ValidFile?"=w1278:bool)
            n743 = case shown="True" w1278 {
              tunnel: w1273 -> [w1279 w1283]
              tunnel: [w1279 w1282] -> w1272
              frame False {
              }
              frame True {
                n744 = Insert Into Array(array=w1283, index=0, new element="Save Test Config" ("new element/subarray")) -> (w1282:string[])
              }
            }
            n745 = call "Remove Tildes (String).vi"("String In"="Notes") -> ("String Out"=w1274:string)  [unwired: 2 in]
            n746 = Bundle By Name(cluster=w1277, "Notes"=w1274) -> (w1276:T15)
          }
          event "Parameters": Key Down? {
            n747 = event-data() -> ("CtlRef"=w1298:refnum<vi>, "Char"=w1297:i16, "VKey"=w1296:T28, "ScanCode"=w1295:i16)  [unwired: 1 in]
            n748 = Unbundle By Name(w1292) -> ("Controller.Controller?"=w1293:bool)
            n749 = local read "TestType"() -> (w1289:enum32{"Flow", "Test", "Hot\nFuel"})
            n750 = call "ProfilesTableControl.vi"("CtlRef"=w1298, "Flow?"=w1289, "Controller?"=w1293, "CharIn"=w1297, "VKey"=w1296, "ScanCode"=w1295) -> ("ColInsert?"=w1284:bool, "CharOut"=w1299:i16, "Discard?"=w1294:bool)  [unwired: 7 in]
            n751 = Insert Into Array(array=w1288, index=0, new element="Store Parameters" ("new element/subarray")) -> (w1287:string[])
            n752 = Bundle By Name(cluster=w1292, "KF.Parameters"=TRUE, "ColInsert"=w1284) -> (w1291:T15)
            n753 = event-data("Char"=w1299, "Discard?"=w1294) -> ()  [unwired: 1 in, 1 out]
          }
          event "Parameters": Value Change {
            n754 = event-data() -> ()  [unwired: 1 in, 1 out]
            n755 = Insert Into Array(array=w1302, index=0, new element=string[] ["Store Parameters", "Eval Para No Warning"]) -> (w1301:string[])
          }
          event "TestType": Value Change {
            n756 = event-data() -> ()  [unwired: 1 in, 1 out]
            n757 = Insert Into Array(array=w1309, index=0, new element=string[] ["Alter Parameter Setup", "Eval Parameters"]) -> (w1308:string[])
          }
          event "Pressure Control": Value Change {
            n758 = event-data() -> ()  [unwired: 1 in, 1 out]
            n759 = Flatten To String(anything="Pressure Control") -> (data string=w1319:string, error out=w1311:errorcluster)  [unwired: 3 in, 1 out]
            n760 = Bundle(cluster=T22 {"Command"="", "FlattenedData"=""}, "Command"="NeedleValve", "FlattenedData"=w1319) -> (w1317:T22)
            n761 = Flatten To String(anything=w1317, error in (no error)=w1311) -> (data string=w1313:string, error out=w1312:errorcluster)  [unwired: 2 in, 1 out]
            n762 = call "PC Send Event.vi"("PC Send Command"=PCsend_RTrecv_CMD."NeedleValve", "Mode"=Event_Mode."Set", "Flattened Data"=w1313, "Error In"=w1312) -> ()  [unwired: 10 in, 2 out]
          }
          event "pb.load profile": Value Change {
            n763 = event-data() -> ()  [unwired: 1 in, 1 out]
            n764 = Insert Into Array(array=w1325, index=0, new element="Load Profile Prep" ("new element/subarray")) -> (w1324:string[])
          }
          event "Steps": Value Change {
            n765 = event-data() -> ()  [unwired: 1 in, 1 out]
            n766 = Unbundle By Name(w1345) -> ("Controller.Controller?"=w1343:bool, "CommandCluster"=w1352:T6, "Parameters"=w1351:string[][], "Controller.Stop Command"=w1340:dbl)
            n767 = case shown="0" "Steps" {
              selector: "Steps" -> [_ w1361]
              tunnel: [w1353 w1359] -> w1331
              tunnel: w1352 -> [_ w1358]
              tunnel: w1351 -> [_ w1357]
              tunnel: w1340 -> [w1355 _]
              tunnel: w1343 -> [_ w1356]
              frame 0 {
                n768 = Bundle By Name(cluster=T6 {"Para1"=0, "SP1"=0.0, "Para2"=1, "SP2"=0.0, "Para3"=4, "SP3"=0.0} ("CMD Cluster Out"), "SP3"=w1355) -> (w1353:T6)
              }
              frame 1.., Default {
                n769 = Decrement(x=w1361) -> (x-1=w1360:u16)
                n770 = call "Test Step Parser.vi"("Controller?"=w1356, "Step In"=w1360, "CMD Cluster IN"=w1358, "Profile"=w1357) -> ("CMD Cluster Out"=w1359:T6)  [unwired: 8 in, 3 out]
              }
            }
            n771 = Unbundle By Name(w1331) -> ("Para1"=w1339:i32, "SP1"=w1350:dbl, "Para2"=w1338:i32, "SP2"=w1349:dbl, "Para3"=w1347:i32, "SP3"=w1341:dbl)
            n772 = Equal?(x=4, y=w1339) -> (x = y?=w1335:bool)
            n773 = Insert Into Array(array=w1329, index=0, new element=string[] ["Write Command", "PS Abler"]) -> (w1328:string[])
            n774 = local write "Parameter 1"(w1339) -> ()
            n775 = local write "Setpoint1"(w1350) -> ()
            n776 = local write "Parameter 2"(w1338) -> ()
            n777 = local write "Setpoint2"(w1349) -> ()
            n778 = local write "Parameter 3"(w1347) -> ()
            n779 = local write "Setpoint3"(w1341) -> ()
            n780 = Build Array(w1339) -> (w1333:i32[])
            n781 = Build Array(w1338) -> (w1342:i32[])
            n782 = Bundle By Name(cluster=w1345, "CommandCluster"=w1331, "DesiredParameters"=w1331) -> (w1344:T15)
            n783 = call "Handle Parameter 3 Control.vi"("Parameter 1"=w1339, "Parameter 2"=w1338, "Stop Command"=w1340, "Last Command"=w1341) -> ("Parameter 3"=w1337:i32, "Error Out"=w1336:errorcluster)  [unwired: 9 in, 1 out]
            n784 = Select(t=i32[] [1, 2, 3] ("appended array"), s=w1335, f=w1333) -> (s? t:f=w1332:i32[])
            n785 = property on="Parameter 2" class="Enum (strict)"("Disabled Items []"=w1332) -> ()  [unwired: 2 in, 2 out]
            n786 = property on="Parameter 1" class="Enum (strict)"("Disabled Items []"=w1342) -> ()  [unwired: 2 in, 2 out]
            n787 = call "Set Parameter Controls.vi"("Para 1"=w1339, "Para 2"=w1338, "Para 3"=w1337, "Error In"=w1336) -> ()  [unwired: 11 in, 1 out]
          }
          event "FFTwindowMax", "FFTwindowMin": Value Change {
            n788 = event-data() -> ()  [unwired: 1 in, 1 out]
            n789 = Bundle("FFTwindowMin"="FFTwindowMin", "FFTwindowMax"="FFTwindowMax") -> (w1362:cluster{"FFTwindowMin":u16, "FFTwindowMax":u16})  [unwired: 1 in]
            n790 = Flatten To String(anything=w1362) -> (data string=w1373:string, error out=w1365:errorcluster)  [unwired: 3 in, 1 out]
            n791 = Bundle(cluster=T22 {"Command"="", "FlattenedData"=""}, "Command"="SpeedWindow", "FlattenedData"=w1373) -> (w1371:T22)
            n792 = Flatten To String(anything=w1371, error in (no error)=w1365) -> (data string=w1367:string, error out=w1366:errorcluster)  [unwired: 2 in, 1 out]
            n793 = call "PC Send Event.vi"("PC Send Command"=PCsend_RTrecv_CMD."SpeedWindow", "Mode"=Event_Mode."Set", "Flattened Data"=w1367, "Error In"=w1366) -> ()  [unwired: 10 in, 2 out]
          }
          event "Tables": Value Change {
            n794 = event-data() -> ()  [unwired: 1 in, 1 out]
            n795 = Equal?(x="Tables", y=enum32{"Data", "Stats", "Notes"}."Notes" ("Tables")) -> (x = y?=w1376:bool)
            n796 = property on="Notes" class="Str"("Key Focus"=w1376) -> ()  [unwired: 2 in, 2 out]
          }
          event "pb.ClearProfile": Value Change {
            w1383 = string[][] [] ("Parameters")
            n797 = event-data() -> ()  [unwired: 1 in, 6 out]
            n798 = local write "Parameters"(w1383) -> ()
            n799 = Bundle By Name(cluster=w1382, "Parameters"=w1383) -> (w1381:T15)
            n800 = Insert Into Array(array=w1385, index=0, new element=string[] ["Store Parameters", "Eval Para No Warning"]) -> (w1384:string[])
          }
        }
      }
      frame "Save Check New" {
        n801 = call <vilib>:"Three Button Dialog.vi"("Allow user to close window? (TRUE)"=FALSE, "message"="Data has been stored without a file location to save to. Would you like to save the data?") -> ("Which Button?"=w1392:T29)  [unwired: 9 in]
        n802 = case shown="\"Center Button\"" w1392 {
          tunnel: [w1397 w1403 w1410] -> w1390
          tunnel: w1391 -> [w1398 w1404 w1410]
          tunnel: w1389 -> [w1396 w1408 w1409]
          tunnel: [w1395 w1407 w1409] -> w1388
          frame "Left Button", Default {
            # "Yes"
            n803 = Bundle By Name(cluster=w1398, "KeepManualPts"=TRUE) -> (w1397:T15)
            n804 = Insert Into Array(array=w1396, index=0, new element="New File" ("new element/subarray")) -> (w1395:string[])
          }
          frame "Center Button" {
            # "No"
            n805 = Bundle By Name(cluster=w1404, "KeepManualPts"=FALSE) -> (w1403:T15)
            n806 = Insert Into Array(array=w1408, index=0, new element="New File" ("new element/subarray")) -> (w1407:string[])
          }
          frame "Right Button" {
            # "Cancel"
          }
        }
      }
      frame "Save Check Load" {
        n807 = call <vilib>:"Three Button Dialog.vi"("Allow user to close window? (TRUE)"=FALSE, "message"="Data has been stored without a file location to save to. Would you like to save the data?") -> ("Which Button?"=w1415:T29)  [unwired: 9 in]
        n808 = case shown="\"Center Button\"" w1415 {
          tunnel: [w1421 w1427 w1433] -> w1413
          tunnel: w1414 -> [w1422 w1428 w1433]
          tunnel: w1412 -> [w1420 w1431 w1432]
          tunnel: [w1419 w1430 w1432] -> w1411
          frame "Left Button", Default {
            # "Yes"
            n809 = Bundle By Name(cluster=w1422, "KeepManualPts"=TRUE) -> (w1421:T15)
            n810 = Insert Into Array(array=w1420, index=0, new element=string[] ["Load File"]) -> (w1419:string[])
          }
          frame "Center Button" {
            # "No"
            n811 = Bundle By Name(cluster=w1428, "KeepManualPts"=FALSE) -> (w1427:T15)
            n812 = Insert Into Array(array=w1431, index=0, new element=string[] ["Load File"]) -> (w1430:string[])
          }
          frame "Right Button" {
            # "Cancel"
          }
        }
      }
      frame "New File" {
        # "Probably redundant..."
        n813 = Unbundle By Name(w1440) -> ("DefaultDataPath"=w1444:path, "Created/ModFiles"=w1445:cluster{"FilePath":path, "Save?":bool}[], "TemplatePath"=w1434:path, "KeepManualPts"=w1439:bool)
        n814 = call "File Dialog4"("start path"=w1444, "prompt"="Create a new file", "pattern (all files)"="*.xlsx", "pattern label"="Excel Workbook") -> ("selected path"=w1451:path, "cancelled"=w1449:bool, "error out"=w1452:errorcluster)  [unwired: 8 in, 1 out]
        n815 = call <vilib>:"Check if File or Folder Exists.vi"("path"=w1451) -> ("file or folder exists?"=w1450:bool, "dup path"=w1447:path)  [unwired: 8 in, 1 out]
        n816 = call <vilib>:"Clear Errors.vi"("error in (no error)"=w1452) -> ()  [unwired: 6 in, 1 out]
        n817 = case shown="True" w1450 {
          tunnel: w1449 -> [w1456 _]
          tunnel: [w1456 w1457] -> w1448
          tunnel: w1447 -> [w1455 w1459]
          tunnel: [w1455 w1458] -> w1446
          frame False {
            # "The file does not exist\n\nno changes needed"
          }
          frame True {
            n818 = Two Button Dialog(message="File already exists! Continuing will permanently delete all previous data.", 2:"Continue" ("T button name (\"OK\")")) -> (T button?=w1460:bool)  [unwired: 1 in]
            n819 = case shown="True" w1460 {
              tunnel: w1459 -> [w1464 w1467]
              tunnel: [w1464 w1466] -> w1458
              tunnel: [TRUE FALSE] -> w1457
              frame False {
                # "cancel any\nactions\ndont want\nto delete\nfile already\ncreated"
              }
              frame True {
                # "Delete file\ndont cancel\nstart fresh\nfile with \nsame name"
                n820 = Delete(path (use dialog)=w1467) -> (deleted path=w1466:path)  [unwired: 4 in, 2 out]
              }
            }
          }
        }
        n821 = Select(t=string[] ["Save Config", "Save Test Config", "Save Component Data"], s=w1439, f=string[] ["Save Config", "New Test Config", "Save Test Config"]) -> (s? t:f=w1436:string[])
        n822 = case shown="False" w1448 {
          tunnel: w1440 -> [w1470 w1487]
          tunnel: [w1469 w1486] -> w1443
          tunnel: w1446 -> [_ w1485]
          tunnel: w1442 -> [w1471 w1482]
          tunnel: [w1471 w1481] -> w1441
          tunnel: w1445 -> [_ w1479]
          tunnel: w1436 -> [_ w1477]
          tunnel: w1434 -> [_ w1473]
          frame True {
            # "New File Canceled"
            n823 = Bundle By Name(cluster=w1470, "KeepManualPts"=FALSE) -> (w1469:T15)
          }
          frame False {
            n824 = Path To String(path=w1485) -> (string=w1489:string)
            n825 = Equal?(x=path "" ("selected path"), y=w1485) -> (x = y?=w1478:bool)
            n826 = Strip Path(path=w1485) -> (stripped path=w1488:path)  [unwired: 1 out]
            n827 = Select(t="", s=w1478, f=w1489) -> (s? t:f=w1484:string)
            n828 = case shown="False" w1478 {
              tunnel: w1485 -> [_ w1493]
              tunnel: w1473 -> [_ w1492]
              frame True {
              }
              frame False {
                # "If the path is not empty\nor created, create the file"
                n829 = call "Create Hidden Files.vi"("TemplatePath"=w1492, "DataFilePath"=w1493) -> ()  [unwired: 7 in, 3 out]
              }
            }
            n830 = local write "File Location"(w1484) -> ()
            n831 = local write "RS File Location"(w1484) -> ()
            n832 = case shown="False" w1478 {
              tunnel: w1487 -> [w1503 w1507]
              tunnel: [w1502 w1506] -> w1486
              tunnel: w1485 -> [w1495 w1505]
              tunnel: w1488 -> [w1501 _]
              tunnel: w1479 -> [w1498 _]
              frame False {
                w1494 = TRUE ("ValidFile?")
                n833 = Bundle("deleted path"=w1495, TRUE) -> (w1496:cluster{"deleted path":path, bool})  [unwired: 1 in]
                n834 = Build Array (concatenate)(w1496, w1498) -> (w1500:cluster{"FilePath":path, "Save?":bool}[])
                n835 = Bundle By Name(cluster=w1503, "Created/ModFiles"=w1500, "CurrentDataFile"=w1495, "DefaultDataPath"=w1501, "ValidFile?"=w1494, "KeepManualPts"=FALSE, "NotLoadProfile"=w1494) -> (w1502:T15)
              }
              frame True {
                n836 = Bundle By Name(cluster=w1507, "CurrentDataFile"=w1505, "KeepManualPts"=FALSE) -> (w1506:T15)
              }
            }
            n837 = Insert Into Array(array=w1482, index=0, new element=w1477) -> (w1481:string[])
            n838 = Select(t=enum16{"Init", "Enable", "Disable", "AutoPop"}."Disable" ("Mode"), s=w1478, f=enum16{"Init", "Enable", "Disable", "AutoPop"}."Enable" ("Mode")) -> (s? t:f=w1474:enum16{"Init", "Enable", "Disable", "AutoPop"})
            n839 = property on="pb.load profile" class="Bool"("DisabledEnum"=T17."Enabled" ("Disabled")) -> ()  [unwired: 2 in, 2 out]
            n840 = property on="pb.save" class="Bool"("DisabledEnum"=T17."Disabled and Grayed Out" ("Disabled")) -> ()  [unwired: 2 in, 2 out]
            n841 = call "Test Config Enabler.vi"("Mode"=w1474) -> ()  [unwired: 15 in]
          }
        }
      }
      frame "Load File" {
        # "F:File has already been opened once during this run of the program - prevent opening"
        # "File exists and is the\ncorrect filetype"
        n842 = Unbundle By Name(w1520) -> ("Created/ModFiles"=w1516:cluster{"FilePath":path, "Save?":bool}[], "PreviousDataFile"=w1519:path, "CurrentDataFile"=w1533:path, "Created/ModFiles"=w1517:cluster{"FilePath":path, "Save?":bool}[])
        n843 = for {
          tunnel: w1516 -> [w1540] mode=indexing
          tunnel: [w1539] -> w1514 mode=indexing
          n844 = Unbundle(w1540) -> ("FilePath"=w1539:path)  [unwired: 1 out]
        }
        n845 = Empty String/Path?(string/path=w1533) -> (empty?=w1534:bool)
        n846 = Select(t=w1519, s=w1534, f=w1533) -> (s? t:f=w1527:path)
        n847 = Strip Path(path=w1527) -> (name=w1526:string)  [unwired: 1 out]
        n848 = call "File Dialog"("start path"=w1527, "prompt"="Select a file to load", "default name"=w1526, "pattern (all files)"="*.xlsx", "pattern label"="Excel Workbook") -> ("selected path"=w1515:path, "cancelled"=w1512:bool, "error out"=w1531:errorcluster)  [unwired: 7 in, 1 out]
        n849 = Path To String(path=w1515) -> (string=w1532:string)
        n850 = Equal?(x=path "" ("selected path"), y=w1515) -> (x = y?=w1530:bool)
        n851 = Search 1D Array(1D array=w1514, element=w1515) -> (index of element=w1513:i32)  [unwired: 1 in]
        n852 = Strip Path(path=w1515) -> (stripped path=w1529:path)  [unwired: 1 out]
        n853 = call <vilib>:"Clear Errors.vi"("error in (no error)"=w1531) -> ()  [unwired: 6 in, 1 out]
        n854 = Less Than 0?(x=w1513) -> (x < 0?=w1509:bool)
        n855 = Select(t="", s=w1530, f=w1532) -> (s? t:f=w1528:string)
        n856 = call <vilib>:"Check if File or Folder Exists.vi"("path"=w1515) -> ("file or folder exists?"=w1525:bool)  [unwired: 8 in, 2 out]
        n857 = call "Excel File Query.vi"("Filename"=w1528) -> ("Excel File?"=w1524:bool)  [unwired: 4 in]
        n858 = And(x=w1525, y=w1524) -> (x .and. y?=w1510:bool)
        n859 = And(x=w1509, y=w1512) -> (x .and. y?=w1511:bool)
        n860 = And(x=w1509, y=w1510) -> (x .and. y?=w1508:bool)
        n861 = case shown="True" w1508 {
          tunnel: w1522 -> [w1543 w1554]
          tunnel: [w1543 w1553] -> w1521
          tunnel: w1530 -> [_ w1552]
          tunnel: w1515 -> [_ w1551]
          tunnel: w1529 -> [_ w1550]
          tunnel: [w1542 w1549] -> w1523
          tunnel: w1520 -> [w1542 w1548]
          tunnel: w1528 -> [_ w1547]
          tunnel: w1511 -> [w1541 _]
          tunnel: w1517 -> [_ w1546]
          frame False {
            n862 = case shown="False" w1541 {
              frame True {
                # "Load file was\ncancelled\n\ndo not error"
              }
              frame False {
                n863 = One Button Dialog(message="Invalid File!") -> ()  [unwired: 1 in, 1 out]
              }
            }
          }
          frame True {
            n864 = local write "File Location"(w1547) -> ()
            n865 = local write "RS File Location"(w1547) -> ()
            n866 = case shown="False" w1552 {
              tunnel: w1548 -> [w1565 w1568]
              tunnel: [w1564 w1567] -> w1549
              tunnel: w1551 -> [w1562 w1566]
              tunnel: w1550 -> [w1563 _]
              tunnel: w1546 -> [w1559 _]
              frame False {
                n867 = Bundle("selected path"=w1562, FALSE) -> (w1561:cluster{"selected path":path, bool})  [unwired: 1 in]
                n868 = Build Array (concatenate)(w1561, w1559) -> (w1558:cluster{"FilePath":path, "Save?":bool}[])
                n869 = Bundle By Name(cluster=w1565, "CurrentDataFile"=w1562, "DefaultDataPath"=w1563, "Created/ModFiles"=w1558, "NotLoadProfile"=TRUE) -> (w1564:T15)
              }
              frame True {
                n870 = Bundle By Name(cluster=w1568, "CurrentDataFile"=w1566) -> (w1567:T15)
              }
            }
            n871 = Insert Into Array(array=w1554, index=0, new element=string[] ["Load Data File", "Verify Stats"]) -> (w1553:string[])
            n872 = property on="pb.load profile" class="Bool"("DisabledEnum"=T17."Enabled" ("Disabled")) -> ()  [unwired: 2 in, 2 out]
          }
        }
      }
      frame "Load Profile Prep" {
        # "File exists and is the\ncorrect filetype"
        n873 = Unbundle By Name(w1570) -> ("PreviousDataFile"=w1572:path, "CurrentDataFile"=w1587:path)
        n874 = Empty String/Path?(string/path=w1587) -> (empty?=w1588:bool)
        n875 = Select(t=w1572, s=w1588, f=w1587) -> (s? t:f=w1580:path)
        n876 = Strip Path(path=w1580) -> (name=w1579:string)  [unwired: 1 out]
        n877 = call "File Dialog2"("start path"=w1580, "prompt"="Select a file to load", "default name"=w1579, "pattern (all files)"="*.xlsx", "pattern label"="Excel Workbook") -> ("selected path"=w1578:path, "cancelled"=w1581:bool, "error out"=w1585:errorcluster)  [unwired: 7 in, 1 out]
        n878 = Path To String(path=w1578) -> (string=w1586:string)
        n879 = Equal?(x=path "" ("selected path"), y=w1578) -> (x = y?=w1584:bool)
        n880 = Strip Path(path=w1578) -> (stripped path=w1583:path)  [unwired: 1 out]
        n881 = call <vilib>:"Clear Errors.vi"("error in (no error)"=w1585) -> ()  [unwired: 6 in, 1 out]
        n882 = Select(t="", s=w1584, f=w1586) -> (s? t:f=w1582:string)
        n883 = call <vilib>:"Check if File or Folder Exists.vi"("path"=w1578) -> ("file or folder exists?"=w1577:bool)  [unwired: 8 in, 2 out]
        n884 = call "Excel File Query.vi"("Filename"=w1582) -> ("Excel File?"=w1576:bool)  [unwired: 4 in]
        n885 = And(x=w1577, y=w1576) -> (x .and. y?=w1575:bool)
        n886 = case shown="True" w1575 {
          tunnel: w1574 -> [w1595 w1601]
          tunnel: [w1595 w1600] -> w1573
          tunnel: w1584 -> [_ _]
          tunnel: w1578 -> [_ w1599]
          tunnel: w1583 -> [_ _]
          tunnel: w1581 -> [w1594 _]
          tunnel: w1570 -> [w1593 w1598]
          tunnel: [w1593 w1597] -> w1569
          frame False {
            n887 = case shown="False" w1594 {
              frame True {
                # "Load file was\ncancelled\n\ndo not error"
              }
              frame False {
                n888 = One Button Dialog(message="Invalid File!") -> ()  [unwired: 1 in, 1 out]
              }
            }
          }
          frame True {
            n889 = Bundle By Name(cluster=w1598, "ProfilePath"=w1599) -> (w1597:T15)
            n890 = Insert Into Array(array=w1601, index=0, new element=string[] ["Load Profile"]) -> (w1600:string[])
          }
        }
      }
      frame "Load Profile" {
        # "remove all highlighting\nand select (0,0) in both\ntables"
        n891 = Unbundle By Name(w1645) -> ("ValidFile?"=w1605:bool, "TestCfgCluster"=w1614:T11, "LastFileState"=w1637:enum16{"New File", "Load File", "Neither"}, "ProfilePath"=w1646:path, "Controller List"=w1643:T9, "StandConfigCluster"=w1608:T14)
        n892 = disable-structure shown="Enabled" {
          disable-tunnel: w1605 -> [w1647 _]
          disable-tunnel: [w1647 TRUE ("ValidFile?")] -> w1604
          frame Disabled {
          }
          frame Enabled {
          }
        }
        n893 = call "Read Profile from Data File.vi"("Filepath"=w1646, "Controller List"=w1643) -> ("Profile"=w1642:string[][], "Pump Control Style"=w1613:i32, "Test Style"=w1606:enum32{"Flow", "Test", "Hot\nFuel"})  [unwired: 10 in, 1 out]
        n894 = Bundle By Name(cluster=w1614, "Pump Control Style"=w1613) -> (w1611:T11)
        n895 = Index Array(array=w1643, index=w1613) -> (element=w1609:T10)
        n896 = case shown="True" w1604 {
          frame False {
          }
          frame True {
            n897 = property on="pb.save" class="Bool"("DisabledEnum"=T17."Enabled" ("Disabled")) -> ()  [unwired: 2 in, 2 out]
          }
        }
        n898 = Unbundle By Name(w1609) -> ("Stop Command"=w1636:dbl, "Controller?"=w1615:bool, "Controller Name"=w1624:T4)
        n899 = local write "Parameters"(w1642) -> ()
        n900 = local write "TestType"(w1606) -> ()
        n901 = local write "Pump Control Style"(w1613) -> ()
        n902 = call "Set Parameter Controls.vi"("Controls Mode (Set)"=Parameter_Controls_Mode."Update Ranges", "StandConfigCluster"=w1608, "Controller"=w1609) -> ("Error Out"=w1607:errorcluster)  [unwired: 12 in]
        n903 = To Long Integer(number=w1624) -> (32bit integer=w1627:i32)
        n904 = Select(t=w1636, s=w1615, f=0.0) -> (s? t:f=w1619:dbl)
        n905 = Flatten To String(anything=w1627) -> (data string=w1628:string, error out=w1626:errorcluster)  [unwired: 3 in, 1 out]
        n906 = call "Test Config Update.vi"("Mode"=enum16{"Init", "Clear", "Update"}."Update", "TestCfgCluster"=w1611) -> ()  [unwired: 13 in, 1 out]
        n907 = Bundle(cluster=T22 {"Command"="", "FlattenedData"=""}, "Command"="Controller", "FlattenedData"=w1628) -> (w1630:T22)
        n908 = flat-sequence {
          tunnel: w1619 -> [w1649]
          tunnel: w1607 -> [_]
          frame #0 {
            n909 = local write "Setpoint3"(w1649) -> ()
          }
        }
        n910 = Flatten To String(anything=w1630, error in (no error)=w1626) -> (data string=w1632:string, error out=w1625:errorcluster)  [unwired: 2 in, 1 out]
        n911 = case shown="\"New File\", \"Neither\", Default" w1637 {
          tunnel: w1645 -> [w1656 w1673]
          tunnel: [w1655 w1672] -> w1644
          tunnel: w1642 -> [w1654 w1671]
          tunnel: w1609 -> [w1653 w1670]
          tunnel: w1613 -> [w1652 w1669]
          frame "New File", "Neither", Default {
            n912 = Bundle By Name(cluster=w1656, "NotLoadProfile"=FALSE, "Parameters"=w1654, "Controller"=w1653, "TestCfgCluster.Pump Control Style"=w1652) -> (w1655:T15)
          }
          frame "Load File" {
            w1660 = "" ("Technician Name")
            w1663 = T19 {"Row"=-2, "Column"=-2} ("Active Cell:Active Cell")
            w1661 = T19 {"Row"=0, "Column"=-2} ("Active Cell:Active Cell")
            w1662 = T19 {"Row"=0, "Column"=0} ("Active Cell:Active Cell")
            w1664 = u32 16777225 ("Active Cell:Cell Background Color")
            w1668 = string[] [] ("Untested SNs")
            w1667 = string[][] []
            n913 = call "Test Config Update.vi"("Mode"=enum16{"Init", "Clear", "Update"}."Clear") -> ()  [unwired: 14 in, 1 out]
            n914 = property on="table.Data" class="Tbl (strict)"("Active Cell"=w1663, "Cell BG Color"=w1664, "Selection Start"=w1662, "Active Cell"=w1661) -> ()  [unwired: 2 in, 2 out]
            n915 = local write "Notes"(w1660) -> ()
            n916 = local write "Next Serial Number"(w1660) -> ()
            n917 = local write "Serial Number"(w1660) -> ()
            n918 = property on="table.Stats" class="Tbl (strict)"("Active Cell"=w1663, "Cell BG Color"=w1664, "Selection Start"=w1662, "Active Cell"=w1661) -> ()  [unwired: 2 in, 2 out]
            n919 = property on="pb.save" class="Bool"("DisabledEnum"=T17."Disabled and Grayed Out" ("Disabled")) -> ()  [unwired: 2 in, 2 out]
            n920 = local write "Serial Numbers"(w1667) -> ()
            n921 = local write "table.Data"(w1667) -> ()
            n922 = local write "table.Stats"(w1667) -> ()
            n923 = local write "Tested Serial Numbers"(w1667) -> ()
            n924 = local write "Untested Serial Numbers"(w1667) -> ()
            n925 = Bundle By Name(cluster=w1673, "table.Data"=w1667, "table.Stats"=w1667, "ValidFile?"=FALSE, "LastDataRow"=1, "Serial Number"=w1660, "Untested SNs"=w1668, "Tested SNs"=w1668, "Serial Numbers"=w1668, "Parameters"=w1671, "Controller"=w1670, "TestCfgCluster.Pump Control Style"=w1669, "NotLoadProfile"=FALSE) -> (w1672:T15)
          }
        }
        n926 = call "PC Send Event.vi"("PC Send Command"=PCsend_RTrecv_CMD."Controller", "Mode"=Event_Mode."Set", "Flattened Data"=w1632, "Error In"=w1625) -> ()  [unwired: 10 in, 2 out]
        n927 = Not(x=w1615) -> (.not. x?=w1620:bool)
        n928 = Select(t="Pump\nVoltage (V)", s=w1620, f="Controller\nVoltage (V)") -> (s? t:f=w1621:string)
        n929 = Select(t="Pump Current\n(A RMS)" ("Caption.Text"), s=w1615, f="Pump Current\n(A)" ("Caption.Text")) -> (s? t:f=w1616:string)
        n930 = property on="Voltage (DC)" class="DigNum (strict)"("Caption.Text"=w1621) -> ()  [unwired: 2 in, 2 out]
        n931 = property on="PumpCurrent(Arms)" class="DigNum (strict)"("Caption.Text"=w1616) -> ()  [unwired: 2 in, 2 out]
        n932 = Insert Into Array(array=w1640, index=0, new element=string[] ["Write Command", "PS Abler", "Alter Run Screen", "Alter Parameter Setup", "Eval Parameters"]) -> (w1639:string[])
      }
      frame "Save Component Data" {
        w1679 = cluster{u32, u32}[] [{1985280, 1985280}, {6618880, 6618880}, {1985280, 1985280}, {6618880, 6618880}]  # Original Colors
        n933 = Unbundle By Name(w1674) -> ("CurrentDataFile"=w1677:path, "table.Data"=w1678:string[][], "ValidFile?"=w1676:bool, "table.Stats"=w1675:string[][])
        n934 = case shown="True" w1676 {
          tunnel: w1678 -> [_ w1695]
          tunnel: w1677 -> [_ w1682]
          tunnel: w1675 -> [_ w1681]
          frame False {
          }
          frame True {
            n935 = call "Filepath 2 Hidden Files.vi"("DataFilePath"=w1682, "Enum"=enum16{"Data", "Stats", "Specs"}."Stats") -> ("HiddenFilePath"=w1683:path)  [unwired: 13 in]
            n936 = Array Subset(array=w1695, index (col)=0 ("index"), length (col)=13 ("length")) -> (w1692:string[][])  [unwired: 2 in]
            n937 = call "Filepath 2 Hidden Files.vi"("DataFilePath"=w1682, "Enum"=enum16{"Data", "Stats", "Specs"}."Data") -> ("HiddenFilePath"=w1690:path)  [unwired: 13 in]
            n938 = Array Subset(array=w1681, index (col)=0 ("index"), length (col)=13 ("length")) -> (w1686:string[][])  [unwired: 2 in]
            n939 = call-poly <vilib>:"Write To Spreadsheet File.vi"("delimiter (\\t)"="~" ("delimiter (\\t)"), "2D data"=w1692, "file path (dialog if empty)"=w1690) -> ()  [unwired: 5 in, 1 out]
            n940 = call-poly <vilib>:"Write To Spreadsheet File.vi"("delimiter (\\t)"="~" ("delimiter (\\t)"), "2D data"=w1686, "file path (dialog if empty)"=w1683) -> ()  [unwired: 5 in, 1 out]
          }
        }
        n941 = property on="Stabilized?" class="Bool (strict)"("Colors [4]"=w1679) -> ()  [unwired: 2 in, 2 out]
      }
      frame "Store Parameters" {
        # "Had to add the sequence structure because if the row is inserted with the voltage\nactive in edit position then it stays there and is placed in the newly inserted blank row"
        n942 = Unbundle By Name(w1699) -> ("ValidFile?"=w1700:bool, "ColInsert"=w1698:bool)
        n943 = case shown="True" w1698 {
          tunnel: "Parameters" -> [w1703 w1716]
          tunnel: [w1703 w1717] -> w1696
          frame False {
          }
          frame True {
            # "Enter or Return was pressed in the last available row"
            n944 = property on="Parameters" class="Tbl (strict)"() -> ("EditPos"=w1704:T19)  [unwired: 2 in, 2 out]
            n945 = Unbundle(w1704) -> ("Column"=w1714:i32)  [unwired: 1 out]
            n946 = Index Array(array=w1716, index (col)=w1714) -> (element=w1715:string[])  [unwired: 1 in]
            n947 = Index Array(array=w1715) -> (element #1=w1713:string, element #2=w1712:string, element #3=w1711:string, element #4=w1710:string, element #5=w1709:string, element #6=w1708:string, element #7=w1707:string)  [unwired: 7 in]
            n948 = Concatenate Strings(w1713, w1712, w1711, w1710, w1709, w1708, w1707) -> (w1706:string)
            n949 = Empty String/Path?(string/path=w1706) -> (empty?=w1705:bool)
            n950 = case shown="False" w1705 {
              tunnel: [w1718 w1726] -> w1717
              tunnel: w1716 -> [w1718 w1727]
              tunnel: w1714 -> [_ w1725]
              tunnel: w1704 -> [_ w1722]
              frame True {
                # "Next column was empty\n     no action"
              }
              frame False {
                n951 = flat-sequence {
                  tunnel: w1722 -> [w1729]
                  tunnel: w1725 -> [w1730]
                  tunnel: w1727 -> [w1731]
                  tunnel: [w1731] -> w1721
                  tunnel: [w1730] -> w1720
                  tunnel: [w1729] -> w1719
                  tunnel: [w1734] -> w1724
                  tunnel: [w1732] -> w1723
                  tunnel: w1721 -> [w1736]
                  tunnel: w1720 -> [w1733]
                  tunnel: w1719 -> [w1732]
                  tunnel: [w1739] -> w1726
                  tunnel: w1724 -> [w1739]
                  tunnel: w1723 -> [w1738]
                  frame #0 {
                    n952 = property on="Parameters" class="Tbl (strict)"("Key Focus"=FALSE) -> ()  [unwired: 2 in, 2 out]
                  }
                  frame #1 {
                    # "Next column had data\nso insert blank column"
                    n953 = Insert Into Array(array=w1736, index (col)=w1733, new element=string[] [""] ("new element/subarray")) -> (w1734:string[][])  [unwired: 1 in]
                    n954 = local write "Parameters"(w1734) -> ()
                  }
                  frame #2 {
                    n955 = property on="Parameters" class="Tbl (strict)"("Key Focus"=TRUE, "EditPos"=w1738) -> ()  [unwired: 2 in, 2 out]
                  }
                }
              }
            }
          }
        }
        n956 = case shown="True" w1700 {
          frame False {
          }
          frame True {
            n957 = property on="pb.save" class="Bool"("DisabledEnum"=T17."Enabled" ("Disabled")) -> ()  [unwired: 2 in, 2 out]
          }
        }
        n958 = Bundle By Name(cluster=w1699, "Parameters"=w1696) -> (w1701:T15)
      }
      frame "Data Table Mouse Up" {
        n959 = Unbundle By Name(w1743) -> ("table.Data"=w1741:string[][], "table.Stats"=w1744:string[][])
        n960 = property on="table.Data" class="Tbl (strict)"() -> ("Selection Start"=w1745:T19)  [unwired: 2 in, 2 out]
        n961 = Unbundle(w1745) -> ("Row"=w1742:i32)  [unwired: 1 out]
        n962 = call "Full Table Handler.vi"("table.Data"=w1741, "table.Stats"=w1744, "Data Row Index"=w1742) -> ()  [unwired: 13 in]
      }
      frame "Alter Run Screen" {
        w1774 = T30 {"Left"=-755, "Top"=-863}  # 12
        w1775 = T30 {"Left"=-911, "Top"=-863}  # 11
        w1773 = T30 {"Left"=-821, "Top"=-829}  # 10
        w1776 = T30 {"Left"=-1002, "Top"=-829}  # 9
        w1772 = T30 {"Left"=-821, "Top"=-897}  # 8
        w1777 = T30 {"Left"=-1002, "Top"=-897}  # 7
        w1771 = T30 {"Left"=-755, "Top"=-829}  # 6
        w1778 = T30 {"Left"=-911, "Top"=-829}  # 5
        w1770 = T30 {"Left"=-1067, "Top"=-829}  # 4
        w1779 = T30 {"Left"=-755, "Top"=-897}  # 3
        w1769 = T30 {"Left"=-911, "Top"=-897}  # 2
        w1780 = T30 {"Left"=-1067, "Top"=-897}  # 1
        n963 = Unbundle By Name(w1787) -> ("Controller.CommSeg"=w1752:i32, "Controller.Controller?"=w1781:bool, "ValidPara?"=w1750:bool)
        n964 = local read "pb.StartManual"() -> (w1748:bool)
        n965 = local read "Parameters"() -> (w1783:string[][])
        n966 = Empty Array?(array=w1783) -> (empty?=w1782:bool)
        n967 = Not(x=w1782) -> (.not. x?=w1747:bool)
        n968 = Not Equal?(x=2, y=w1752) -> (x != y?=w1784:bool)
        n969 = Compound Arithmetic op=AND(w1750, w1748, w1747) -> (w1749:bool)
        n970 = case shown="True" w1781 {
          tunnel: w1749 -> [w1818 w1870]
          tunnel: w1780 -> [w1815 w1869]
          tunnel: w1779 -> [w1813 w1868]
          tunnel: w1778 -> [w1811 w1867]
          tunnel: w1777 -> [w1809 w1866]
          tunnel: w1776 -> [w1807 w1865]
          tunnel: w1775 -> [w1805 w1864]
          tunnel: w1774 -> [w1804 w1863]
          tunnel: w1773 -> [w1806 w1862]
          tunnel: w1772 -> [w1808 w1861]
          tunnel: w1771 -> [w1810 w1860]
          tunnel: w1770 -> [w1812 w1859]
          tunnel: w1769 -> [w1814 w1858]
          tunnel: w1786 -> [w1817 w1857]
          tunnel: [w1816 w1856] -> w1785
          tunnel: [w1803 w1853] -> w1765
          tunnel: [w1802 w1852] -> w1762
          tunnel: [w1801 w1851] -> w1761
          tunnel: [w1800 w1850] -> w1758
          tunnel: [w1799 w1847] -> w1756
          tunnel: [w1798 w1849] -> w1768
          tunnel: [w1797 w1848] -> w1754
          tunnel: [w1796 w1855] -> w1753
          tunnel: [w1795 w1854] -> w1766
          tunnel: [w1794 w1846] -> w1764
          tunnel: [w1793 w1845] -> w1763
          tunnel: [w1792 w1844] -> w1760
          tunnel: [w1791 w1843] -> w1759
          tunnel: [w1790 w1842] -> w1757
          tunnel: [w1789 w1840] -> w1755
          tunnel: [w1788 w1841] -> w1767
          frame True {
            # "Has Controller - Show Parameter 3"
            n971 = case shown="True" w1818 {
              tunnel: w1817 -> [w1827 w1831]
              tunnel: [w1827 w1830] -> w1816
              tunnel: w1815 -> [w1825 _]
              tunnel: w1814 -> [w1824 w1838]
              tunnel: w1813 -> [w1823 w1835]
              tunnel: w1812 -> [w1822 _]
              tunnel: w1811 -> [w1821 w1836]
              tunnel: w1810 -> [w1820 w1833]
              tunnel: w1809 -> [_ _]
              tunnel: w1808 -> [_ _]
              tunnel: w1807 -> [_ _]
              tunnel: w1806 -> [_ _]
              tunnel: w1805 -> [_ w1837]
              tunnel: w1804 -> [_ w1834]
              tunnel: [w1819 w1839] -> w1803
              tunnel: [w1819 w1839] -> w1802
              tunnel: [w1819 w1839] -> w1801
              tunnel: [w1819 w1839] -> w1800
              tunnel: [w1819 w1839] -> w1799
              tunnel: [w1819 w1832] -> w1798
              tunnel: [w1819 w1839] -> w1797
              tunnel: [w1819 w1832] -> w1796
              tunnel: [FALSE w1832] -> w1795
              tunnel: [w1825 w1838] -> w1794
              tunnel: [w1824 w1837] -> w1793
              tunnel: [w1823 w1836] -> w1792
              tunnel: [w1822 w1835] -> w1791
              tunnel: [w1821 w1834] -> w1790
              tunnel: [w1820 w1833] -> w1789
              tunnel: [w1819 w1832] -> w1788
              frame False {
                w1819 = TRUE
                # "Display parameters normally"
              }
              frame True {
                w1839 = FALSE
                w1832 = TRUE
                # "Manual Mode w/ Test setup\nDisplay steps"
                n972 = Insert Into Array(array=w1831, index=0, new element="Populate Steps Enum" ("new element/subarray")) -> (w1830:string[])
              }
            }
          }
          frame False {
            # "Controllerless - No Parameter 3"
            n973 = case shown="True" w1870 {
              tunnel: w1869 -> [_ _]
              tunnel: w1868 -> [w1872 w1887]
              tunnel: w1867 -> [_ w1885]
              tunnel: w1866 -> [w1878 _]
              tunnel: w1865 -> [w1876 _]
              tunnel: w1864 -> [_ _]
              tunnel: w1863 -> [_ _]
              tunnel: w1862 -> [w1875 _]
              tunnel: w1861 -> [w1877 _]
              tunnel: w1860 -> [w1871 w1888]
              tunnel: w1859 -> [_ _]
              tunnel: w1858 -> [_ w1886]
              tunnel: w1857 -> [w1879 w1882]
              tunnel: [w1879 w1881] -> w1856
              tunnel: [w1873 w1889] -> w1855
              tunnel: [w1873 w1880] -> w1854
              tunnel: [w1874 w1880] -> w1853
              tunnel: [w1874 w1880] -> w1852
              tunnel: [w1873 w1889] -> w1851
              tunnel: [w1874 w1880] -> w1850
              tunnel: [w1873 w1889] -> w1849
              tunnel: [w1873 w1889] -> w1848
              tunnel: [w1874 w1880] -> w1847
              tunnel: [w1878 w1886] -> w1846
              tunnel: [w1877 w1885] -> w1845
              tunnel: [w1872 w1887] -> w1844
              tunnel: [w1876 w1887] -> w1843
              tunnel: [w1875 w1888] -> w1842
              tunnel: [w1873 w1889] -> w1841
              tunnel: [w1871 w1888] -> w1840
              frame False {
                w1874 = TRUE
                w1873 = FALSE
                # "Display parameters normally"
                # "NA"
                # "NA"
              }
              frame True {
                w1889 = FALSE
                w1880 = TRUE
                # "Manual Mode w/ Test setup\nDisplay steps"
                # "NA"
                # "NA"
                n974 = Insert Into Array(array=w1882, index=0, new element="Populate Steps Enum" ("new element/subarray")) -> (w1881:string[])
              }
            }
          }
        }
        n975 = property on="FFTwindowMin" class="DigNum (strict)"("Visible"=w1784) -> ()  [unwired: 2 in, 2 out]
        n976 = property on="FFTwindowMax" class="DigNum (strict)"("Visible"=w1784) -> ()  [unwired: 2 in, 2 out]
        n977 = property on="Controller CMD" class="DigNum (strict)"("Visible"=w1753) -> ()  [unwired: 2 in, 2 out]
        n978 = property on="Steps" class="Ring (strict)"("Visible"=w1766) -> ()  [unwired: 2 in, 2 out]
        n979 = property on="Parameter 1" class="Enum (strict)"("Caption.Visible"=w1765, "Position"=w1764) -> ()  [unwired: 2 in, 2 out]
        n980 = property on="Parameter 2" class="Enum (strict)"("Caption.Visible"=w1762, "Position"=w1763) -> ()  [unwired: 2 in, 2 out]
        n981 = property on="Parameter 3" class="Enum (strict)"("Caption.Visible"=w1761, "Position"=w1760, "Visible"=w1767) -> ()  [unwired: 2 in, 2 out]
        n982 = property on="Setpoint1" class="DigNum (strict)"("Caption.Visible"=w1758, "Position"=w1759) -> ()  [unwired: 2 in, 2 out]
        n983 = property on="Setpoint2" class="DigNum (strict)"("Caption.Visible"=w1756, "Position"=w1757) -> ()  [unwired: 2 in, 2 out]
        n984 = property on="Setpoint3" class="DigNum (strict)"("Caption.Visible"=w1754, "Position"=w1755, "Visible"=w1768) -> ()  [unwired: 2 in, 2 out]
      }
      frame "Alter Parameter Setup" {
        n985 = Unbundle By Name(w1894) -> ("Controller.Controller?"=w1892:bool)
        n986 = local read "TestType"() -> (w1891:enum32{"Flow", "Test", "Hot\nFuel"})
        n987 = case shown="\"Hot\\nFuel\"" w1891 {
          tunnel: w1892 -> [w1899 w1908 w1921]
          tunnel: [w1896 w1905 FALSE ("s")] -> w1890
          frame "Flow" {
            w1896 = TRUE ("s")
            w1897 = u32 16777225  # White
            w1898 = u32 9868950
            n988 = Select(t=w1898, s=w1896, f=w1897) -> (s? t:f=w1901:u32)
            n989 = Select(t=w1897, s=w1899, f=w1898) -> (s? t:f=w1900:u32)
            n990 = property on="Parameters" class="Tbl (strict)"("Active Cell"=T19 {"Row"=-2, "Column"=-2} ("Active Cell:Active Cell"), "Cell BG Color"=w1897, "Active Cell"=T19 {"Row"=1, "Column"=-2} ("Active Cell:Active Cell"), "Cell BG Color"=w1901, "Active Cell"=T19 {"Row"=6, "Column"=-2} ("Active Cell:Active Cell"), "Cell BG Color"=w1900) -> ()  [unwired: 2 in, 2 out]
          }
          frame "Test" {
            w1905 = FALSE ("s")
            w1906 = u32 16777225  # White
            w1907 = u32 9868950
            n991 = Select(t=w1907, s=w1905, f=w1906) -> (s? t:f=w1910:u32)
            n992 = Select(t=w1906, s=w1908, f=w1907) -> (s? t:f=w1909:u32)
            n993 = property on="Parameters" class="Tbl (strict)"("Active Cell"=T19 {"Row"=-2, "Column"=-2} ("Active Cell:Active Cell"), "Cell BG Color"=w1906, "Active Cell"=T19 {"Row"=1, "Column"=-2} ("Active Cell:Active Cell"), "Cell BG Color"=w1910, "Active Cell"=T19 {"Row"=6, "Column"=-2} ("Active Cell:Active Cell"), "Cell BG Color"=w1909) -> ()  [unwired: 2 in, 2 out]
          }
          frame "Hot\nFuel" {
            w1917 = u32 16777225  # White
            n994 = Select(t=w1917, s=w1921, f=u32 9868950) -> (s? t:f=w1914:u32)
            n995 = property on="Parameters" class="Tbl (strict)"("Active Cell"=T19 {"Row"=-2, "Column"=-2} ("Active Cell:Active Cell"), "Cell BG Color"=u32 9868950, "Active Cell"=T19 {"Row"=-2, "Column"=-1} ("Active Cell:Active Cell"), "Cell BG Color"=w1917, "Active Cell"=T19 {"Row"=-2, "Column"=0} ("Active Cell:Active Cell"), "Cell BG Color"=w1917, "Active Cell"=T19 {"Row"=6, "Column"=-1} ("Active Cell:Active Cell"), "Cell BG Color"=w1914, "Active Cell"=T19 {"Row"=6, "Column"=0} ("Active Cell:Active Cell"), "Cell BG Color"=w1914) -> ()  [unwired: 2 in, 2 out]
          }
        }
        n996 = Bundle By Name(cluster=w1894, "Flow?"=w1890) -> (w1893:T15)
      }
      frame "Eval Parameters" {
        n997 = Unbundle By Name(w1947) -> ("ValidFile?"=w1927:bool, "Controller.Command Step"=w1926:dbl, "Parameters"=w1946:string[][], "Controller.Controller?"=w1944:bool, "StandConfigCluster.Max Voltage"=w1954:dbl, "StandConfigCluster.Max Pressure"=w1953:dbl, "StandConfigCluster.Max Flow"=w1952:dbl, "Controller.High Command"=w1951:dbl, "Controller.Low Command"=w1949:dbl, "NotLoadProfile"=w1930:bool)
        n998 = local read "TestType"() -> (w1943:enum32{"Flow", "Test", "Hot\nFuel"})
        n999 = Build Array(w1954, w1953, w1952, 15000.0, w1951) -> (w1942:dbl[])
        n1000 = Replace Array Subset(array=dbl[] [0.0, -1.0, 0.0, 0.0, 0.0], new element=w1949, index=4) -> (w1941:dbl[])
        n1001 = And(x=w1927, y=w1930) -> (x .and. y?=w1929:bool)
        n1002 = call "Valid Test Verification.vi"("Parameters In"=w1946, "CmdStep"=w1926, "Controller?"=w1944, "Enum.Radio"=w1943, "Maxes"=w1942, "Mins"=w1941, "Intermediate?"=FALSE) -> ("Parameters Out"=w1945:string[][], "Valid?"=w1928:bool, "TimeValid?"=w1937:bool, "ProfileValid?"=w1936:bool, "NoCoerces"=w1935:bool)  [unwired: 4 in]
        n1003 = And(x=w1927, y=w1928) -> (x .and. y?=w1931:bool)
        n1004 = case shown="True" w1937 {
          tunnel: w1936 -> [w1961 _]
          tunnel: w1935 -> [w1960 _]
          tunnel: w1940 -> [w1959 w1978]
          tunnel: [w1958 w1978] -> w1939
          tunnel: w1929 -> [w1957 _]
          frame True {
            n1005 = case shown="True" w1961 {
              tunnel: w1960 -> [_ w1967]
              tunnel: w1959 -> [w1962 w1966]
              tunnel: [w1962 w1965] -> w1958
              tunnel: w1957 -> [_ w1964]
              frame False {
                n1006 = One Button Dialog(message="Profile Error: With controller need 3 parameters per step, with out controller 2. Any deadhead step has to have -1 in pressure and a voltage.") -> ()  [unwired: 1 in, 1 out]
              }
              frame True {
                n1007 = case shown="False" w1967 {
                  tunnel: w1966 -> [w1970 w1977]
                  tunnel: [w1969 w1977] -> w1965
                  tunnel: w1964 -> [w1968 _]
                  frame False {
                    n1008 = case shown="True" w1968 {
                      tunnel: w1970 -> [w1972 w1974]
                      tunnel: [w1972 w1973] -> w1969
                      frame False {
                      }
                      frame True {
                        n1009 = Insert Into Array(array=w1974, index=0, new element=string[] ["Save Test Config"]) -> (w1973:string[])
                      }
                    }
                    n1010 = One Button Dialog(message="Values in Parameter Setup have been coerced to the values specified by the Stand Config page.") -> ()  [unwired: 1 in, 1 out]
                  }
                  frame True {
                  }
                }
              }
            }
          }
          frame False {
            n1011 = One Button Dialog(message="When running a test the time row has to be filled out. Time is specified in seconds.") -> ()  [unwired: 1 in, 1 out]
          }
        }
        n1012 = local write "Parameters"(w1945) -> ()
        n1013 = Select(t=T17."Enabled" ("Disabled"), s=w1931, f=T17."Disabled and Grayed Out" ("Disabled")) -> (s? t:f=w1934:T17)
        n1014 = property on="pb.StartTest" class="Bool (strict)"("DisabledEnum"=w1934) -> ()  [unwired: 2 in, 2 out]
        n1015 = Bundle By Name(cluster=w1947, "Parameters"=w1945, "KF.Parameters"=FALSE, "ValidPara?"=w1928) -> (w1956:T15)
      }
      frame "Eval Para No Warning" {
        # "This is meant to be able to keep all values in range so that there\nis no surprise when values change at the end of entering a profile\n\nDeleted a lot of previous case (Eval Parameters) logic as that\ncase will still be ran before it is capable of saving the file"
        n1016 = Unbundle By Name(w1989) -> ("Controller.Command Step"=w1981:dbl, "Parameters"=w1988:string[][], "Controller.Controller?"=w1986:bool, "StandConfigCluster.Max Voltage"=w1996:dbl, "StandConfigCluster.Max Pressure"=w1995:dbl, "StandConfigCluster.Max Flow"=w1994:dbl, "Controller.High Command"=w1993:dbl, "Controller.Low Command"=w1991:dbl)
        n1017 = local read "TestType"() -> (w1985:enum32{"Flow", "Test", "Hot\nFuel"})
        n1018 = Build Array(w1996, w1995, w1994, 15000.0, w1993) -> (w1984:dbl[])
        n1019 = Replace Array Subset(array=dbl[] [0.0, -1.0, 0.0, 0.0, 0.0], new element=w1991, index=4) -> (w1983:dbl[])
        n1020 = call "Valid Test Verification.vi"("Parameters In"=w1988, "CmdStep"=w1981, "Controller?"=w1986, "Enum.Radio"=w1985, "Maxes"=w1984, "Mins"=w1983, "Intermediate?"=TRUE) -> ("Parameters Out"=w1987:string[][])  [unwired: 4 in, 4 out]
        n1021 = local write "Parameters"(w1987) -> ()
        n1022 = Bundle By Name(cluster=w1989, "Parameters"=w1987) -> (w1998:T15)
      }
      frame "Apply Limits" {
        # "In both the previous Eval Parameter cases the minimum for pressure is -1\nthat is so that in a profile a -1 can be a deadhead"
        n1023 = Unbundle By Name(w2013) -> ("CommandCluster.Para1"=w1999:i32, "CommandCluster.SP1"=w2014:dbl, "CommandCluster.Para2"=w2001:i32, "CommandCluster.SP2"=w2015:dbl, "CommandCluster.Para3"=w2000:i32, "CommandCluster.SP3"=w2016:dbl, "StandConfigCluster.Max Voltage"=w2028:dbl, "StandConfigCluster.Max Pressure"=w2027:dbl, "StandConfigCluster.Max Flow"=w2026:dbl, "Controller.High Command"=w2025:dbl, "Controller.Low Command"=w2023:dbl)
        n1024 = Build Array(w2028, w2027, w2026, 15000.0, w2025) -> (w2021:dbl[])
        n1025 = Replace Array Subset(array=dbl[] [0.0, 0.0, 0.0, 0.0, 0.0], new element=w2023, index=4) -> (w2020:dbl[])
        n1026 = Index Array(array=w2021, index=w1999) -> (element=w2019:dbl)
        n1027 = Index Array(array=w2020, index=w1999) -> (element=w2002:dbl)
        n1028 = Index Array(array=w2021, index=w2001) -> (element=w2018:dbl)
        n1029 = Index Array(array=w2020, index=w2001) -> (element=w2004:dbl)
        n1030 = Index Array(array=w2021, index=w2000) -> (element=w2017:dbl)
        n1031 = Index Array(array=w2020, index=w2000) -> (element=w2003:dbl)
        n1032 = Equal?(x=4, y=w1999) -> (x = y?=w2010:bool)
        n1033 = In Range and Coerce(upper limit=w2019, x=w2014, lower limit=w2002) -> (coerced(x)=w2009:dbl)  [unwired: 1 out]
        n1034 = In Range and Coerce(upper limit=w2018, x=w2015, lower limit=w2004) -> (coerced(x)=w2006:dbl)  [unwired: 1 out]
        n1035 = In Range and Coerce(upper limit=w2017, x=w2016, lower limit=w2003) -> (coerced(x)=w2005:dbl)  [unwired: 1 out]
        n1036 = Select(t=0.0, s=w2010, f=w2009) -> (s? t:f=w2007:dbl)
        n1037 = local write "Setpoint1"(w2007) -> ()
        n1038 = local write "Setpoint2"(w2006) -> ()
        n1039 = local write "Setpoint3"(w2005) -> ()
        n1040 = Bundle By Name(cluster=w2013, "CommandCluster.SP1"=w2007, "CommandCluster.SP2"=w2006, "CommandCluster.SP3"=w2005) -> (w2012:T15)
      }
      frame "Write Command" {
        w2039 = T6 {"Para1"=0, "SP1"=0.0, "Para2"=0, "SP2"=0.0, "Para3"=0, "SP3"=0.0}  # CommandCluster
        n1041 = Unbundle By Name(w2038) -> ("CommandCluster.Para1"=w2058:i32, "CommandCluster.SP1"=w2057:dbl, "CommandCluster.Para2"=w2055:i32, "CommandCluster.SP2"=w2054:dbl, "CommandCluster.Para3"=w2051:i32, "CommandCluster.SP3"=w2052:dbl, "DesiredParameters"=w2031:T6)
        n1042 = case shown="4" w2058 {
          selector: w2058 -> [w2062 w2063]
          tunnel: [w2062 w2066] -> w2049
          tunnel: w2057 -> [w2061 _]
          tunnel: [w2061 w2065] -> w2056
          tunnel: w2055 -> [w2060 w2066]
          tunnel: [w2060 w2063] -> w2050
          tunnel: w2054 -> [w2059 w2065]
          tunnel: [w2059 0.0 ("Setpoint2")] -> w2053
          frame Default {
          }
          frame 4 {
          }
        }
        n1043 = Bundle(cluster=w2039, "Para1"=w2049, "SP1"=w2056, "Para2"=w2050, "SP2"=w2053, "Para3"=w2051, "SP3"=w2052) -> (w2033:T6)
        n1044 = Bundle("CommandCluster"=w2033, "DesiredParameters"=w2031) -> (w2032:T31)  [unwired: 1 in]
        n1045 = Insert Into Array(array=w2036, index=0, new element=string[] ["PS Abler"]) -> (w2035:string[])
        n1046 = Flatten To String(anything=w2032) -> (data string=w2045:string, error out=w2041:errorcluster)  [unwired: 3 in, 1 out]
        n1047 = Bundle(cluster=T22 {"Command"="", "FlattenedData"=""}, "Command"="CMD", "FlattenedData"=w2045) -> (w2043:T22)
        n1048 = Flatten To String(anything=w2043, error in (no error)=w2041) -> (data string=w2042:string, error out=w2040:errorcluster)  [unwired: 2 in, 1 out]
        n1049 = call "PC Send Event.vi"("PC Send Command"=PCsend_RTrecv_CMD."CMD", "Mode"=Event_Mode."Set", "Flattened Data"=w2042, "Error In"=w2040) -> ()  [unwired: 10 in, 2 out]
      }
      frame "Stop Manual" {
        w2079 = 0.0 ("Setpoint1")
        n1050 = Unbundle By Name(w2082) -> ("CommandCluster"=w2068:T6, "CommandCluster.Para3"=w2077:i32, "Controller.Stop Command"=w2080:dbl)
        n1051 = Equal?(x=w2077, y=T2."Command") -> (x = y?=w2076:bool)
        n1052 = local write "Setpoint1"(w2079) -> ()
        n1053 = local write "Setpoint2"(w2079) -> ()
        n1054 = Select(t=w2080, s=w2076, f=w2079) -> (s? t:f=w2069:dbl)
        n1055 = Bundle(cluster=w2068, "Para1"=0 ("CommandCluster.Para2"), "SP1"=w2079, "Para2"=1 ("CommandCluster.Para2"), "SP2"=w2079, "Para3"=w2077, "SP3"=w2069) -> (w2067:T6)
        n1056 = Insert Into Array(array=w2073, index=0, new element=string[] ["Write Command"]) -> (w2070:string[])
        n1057 = Bundle By Name(cluster=w2082, "CommandCluster"=w2067, "DesiredParameters"=w2067) -> (w2081:T15)
        n1058 = local write "Setpoint3"(w2069) -> ()
      }
      frame "New Test Config" {
        w2087 = T19 {"Row"=-2, "Column"=-2} ("Active Cell:Active Cell")
        w2085 = T19 {"Row"=0, "Column"=-2} ("Active Cell:Active Cell")
        w2086 = T19 {"Row"=0, "Column"=0} ("Active Cell:Active Cell")
        w2088 = u32 16777225 ("Active Cell:Cell Background Color")
        w2089 = string[] [] ("Untested SNs")
        w2094 = T11 {"Technician Name"="", "Shop Order Number"="", "Customer"="", "Platform"="", "Flow Test Fluid"="", "Fuel Batch #"="", "CA Number"="", "Durability Tank #"="", "Durability Fluid"="", "Hours Completed"="", "Pump Model"="", "Pump Control Style"=enum."Kuhnke"}  # TestCfgCluster
        w2092 = "" ("Technician Name")
        w2084 = string[][] []
        # "Why am I not updating\nthese in the main bundle?"
        # "Keep the selected pump\ncontrol style but reset\neverything else to default"
        # "remove all highlighting\nand select (0,0) in both\ntables"
        n1059 = Unbundle By Name(w2096) -> ("TestCfgCluster.Pump Control Style"=w2095:T4)
        n1060 = local write "Serial Numbers"(w2084) -> ()
        n1061 = local write "Parameters"(w2084) -> ()
        n1062 = local write "table.Data"(w2084) -> ()
        n1063 = local write "table.Stats"(w2084) -> ()
        n1064 = local write "Tested Serial Numbers"(w2084) -> ()
        n1065 = local write "Untested Serial Numbers"(w2084) -> ()
        n1066 = property on="table.Data" class="Tbl (strict)"("Active Cell"=w2087, "Cell BG Color"=w2088, "Selection Start"=w2086, "Active Cell"=w2085) -> ()  [unwired: 2 in, 2 out]
        n1067 = Bundle By Name(cluster=w2094, "Pump Control Style"=w2095) -> (w2093:T11)
        n1068 = property on="table.Stats" class="Tbl (strict)"("Active Cell"=w2087, "Cell BG Color"=w2088, "Selection Start"=w2086, "Active Cell"=w2085) -> ()  [unwired: 2 in, 2 out]
        n1069 = Bundle By Name(cluster=w2096, "LastDataRow"=1 ("TotalPts"), "TestCfgCluster"=w2093, "Parameters"=w2084, "table.Data"=w2084, "table.Stats"=w2084, "Serial Number"=w2092, "ValidFile?"=FALSE, "Untested SNs"=w2089, "Tested SNs"=w2089, "Serial Numbers"=w2089) -> (w2097:T15)
        n1070 = local write "Notes"(w2092) -> ()
        n1071 = local write "Serial Number"(w2092) -> ()
        n1072 = local write "Next Serial Number"(w2092) -> ()
        n1073 = call "Test Config Update.vi"("Mode"=enum16{"Init", "Clear", "Update"}."Clear") -> ()  [unwired: 14 in, 1 out]
      }
      frame "Save Test Config" {
        w2111 = 0 ("index")
        n1074 = Unbundle By Name(w2137) -> ("Parameters"=w2115:string[][], "Serial Numbers"=w2133:string[], "TestCfgCluster.CA Number"=w2132:string, "TestCfgCluster.Shop Order Number"=w2131:string, "TestCfgCluster.Customer"=w2130:string, "TestCfgCluster.Platform"=w2129:string, "TestCfgCluster.Flow Test Fluid"=w2128:string, "TestCfgCluster.Fuel Batch #"=w2127:string, "TestCfgCluster.Pump Model"=w2126:string, "TestCfgCluster.Pump Control Style"=w2122:T4, "TestCfgCluster.Technician Name"=w2125:string, "TestCfgCluster.Durability Tank #"=w2124:string, "TestCfgCluster.Durability Fluid"=w2123:string, "TestCfgCluster.Hours Completed"=w2120:string, "Notes"=w2103:string, "Gauge Number"=w2116:string, "Calibration Due Date"=w2119:string, "CurrentDataFile"=w2114:path, "Created/ModFiles"=w2108:cluster{"FilePath":path, "Save?":bool}[])
        n1075 = local read "TestType"() -> (w2106:enum32{"Flow", "Test", "Hot\nFuel"})
        n1076 = Index Array(array=string[] ["Flow", "Test", "Hot Fuel"], index=w2106) -> (element=w2105:string)
        n1077 = property on="Pump Control Style" class="Enum (strict)"() -> ("Strings []"=w2139:string[])  [unwired: 2 in, 2 out]
        n1078 = Index Array(array=w2139, index=w2122) -> (element=w2121:string)
        n1079 = call "Remove Blanks (String Array).vi"("Array In"=w2133) -> ("Array Out"=w2134:string[])  [unwired: 18 in]
        n1080 = Index Array(array=w2108, index=w2111) -> (element=w2109:cluster{"FilePath":path, "Save?":bool})
        n1081 = Bundle By Name(cluster=w2109, "Save?"=TRUE) -> (w2110:cluster{"FilePath":path, "Save?":bool})
        n1082 = property on="pb.save" class="Bool"("DisabledEnum"=T17."Disabled and Grayed Out" ("Disabled")) -> ()  [unwired: 2 in, 2 out]
        n1083 = Replace Array Subset(array=w2108, new element=w2110, index=w2111) -> (w2107:cluster{"FilePath":path, "Save?":bool}[])
        n1084 = call <vilib>:"Space Constant.vi"() -> ("String"=w2101:string)
        n1085 = Bundle By Name(cluster=w2137, "ValidFile?"=TRUE, "PreviousDataFile"=w2114, "Created/ModFiles"=w2107) -> (w2136:T15)
        n1086 = Concatenate Strings(w2101, w2101, w2101, w2101, w2101) -> (w2100:string)
        n1087 = Search and Replace String(replace all?=TRUE ("replace all? (F)"), input string=w2103, search string="\n", replace string=w2100) -> (result string=w2102:string)  [unwired: 4 in, 3 out]
        n1088 = Build Array(w2132, w2131, w2130, w2129, w2128, w2127, w2126, w2121, w2125, w2124, w2123, w2120, w2102, w2116, w2119) -> (w2138:string[])
        n1089 = call "Save Hidden Config.vi"("EnumRadio"=w2105, "DataFilePath"=w2114, "Profile"=w2115, "Serial Numbers"=w2134, "Header Info"=w2138) -> ()  [unwired: 11 in]
      }
      frame "Start Test Prep" {
        n1090 = flat-sequence {
          tunnel: [w2167] -> w2145
          tunnel: w2144 -> [w2164]
          tunnel: w2144 -> [w2163]
          frame #0 {
            w2150 = 0 ("index")
            w2148 = TRUE ("TestRunning?")
            w2147 = T17."Disabled" ("Disabled")
            # "Added this in to point the data to the bottom of the array that way the data\nwon't just get shoved in between another set of data"
            n1091 = Unbundle By Name(w2164) -> ("Serial Number"=w2161:string, "Serial Numbers"=w2162:string[], "table.Data"=w2149:string[][], "Parameters"=w2146:string[][])
            n1092 = call "SN Analyze.vi"("Run Screen SN"=w2161, "Specified SNs"=w2162, "Data"=w2149, "Profile"=w2146) -> ("Next SN"=w2165:string, "Untested SNs"=w2159:string[], "Tested SNs"=w2155:string[])  [unwired: 9 in]
            n1093 = Array Size(array=w2149) -> (size(s)=w2154:i32[])
            n1094 = Build Array(w2159) -> (w2160:string[][])
            n1095 = Build Array(w2155) -> (w2157:string[][])
            n1096 = Index Array(array=w2154, index=w2150) -> (element=w2153:i32)
            n1097 = Transpose 2D Array(2D array=w2160) -> (transposed array=w2158:string[][])
            n1098 = Transpose 2D Array(2D array=w2157) -> (transposed array=w2156:string[][])
            n1099 = Decrement(x=w2153) -> (x-1=w2152:i32)
            n1100 = Bundle By Name(cluster=w2163, "StepIndex"=0, "TestRunning?"=w2148, "Untested SNs"=w2159, "Tested SNs"=w2155) -> (w2167:T15)
            n1101 = local write "Next Serial Number"(w2165) -> ()
            n1102 = local write "Untested Serial Numbers"(w2158) -> ()
            n1103 = local write "Tested Serial Numbers"(w2156) -> ()
            n1104 = Bundle(w2152, "index"=w2150) -> (w2151:cluster{i32, "index":i32})  [unwired: 1 in]
            n1105 = property on="table.Data" class="Tbl (strict)"("Selection Start"=w2151) -> ()  [unwired: 2 in, 2 out]
            n1106 = property on="Parameter 1" class="Enum (strict)"("DisabledEnum"=w2147) -> ()  [unwired: 2 in, 2 out]
            n1107 = property on="Setpoint1" class="DigNum (strict)"("DisabledEnum"=w2147) -> ()  [unwired: 2 in, 2 out]
            n1108 = property on="Parameter 2" class="Enum (strict)"("DisabledEnum"=w2147) -> ()  [unwired: 2 in, 2 out]
            n1109 = property on="Setpoint2" class="DigNum (strict)"("DisabledEnum"=w2147) -> ()  [unwired: 2 in, 2 out]
            n1110 = property on="Parameter 3" class="Enum (strict)"("DisabledEnum"=w2147) -> ()  [unwired: 2 in, 2 out]
            n1111 = property on="Setpoint3" class="DigNum (strict)"("DisabledEnum"=w2147) -> ()  [unwired: 2 in, 2 out]
            n1112 = property on="Serial Number" class="Str"("DisabledEnum"=w2147) -> ()  [unwired: 2 in, 2 out]
            "Running?" <- w2148
          }
          frame #1 {
            n1113 = property on="pb.select SN" class="Bool"("Key Focus"=TRUE) -> ()  [unwired: 2 in, 2 out]
            n1114 = call "Tab Handler.vi"("Mode"=T21."Other Tab") -> ()  [unwired: 15 in]
            n1115 = local write "Screen"(T1."Part Change" ("Screen")) -> ()
          }
        }
        n1116 = Insert Into Array(array=w2141, index=0, new element=string[] ["Data Table Mouse Up"]) -> (w2140:string[])
      }
      frame "Evaluate SNs" {
        w2182 = 0 ("disabled index (col)")
        w2183 = string[][] []
        n1117 = Unbundle By Name(w2177) -> ("Serial Number"=w2178:string, "Serial Numbers"=w2179:string[], "table.Data"=w2185:string[][], "Parameters"=w2175:string[][])
        n1118 = call "SN Analyze.vi"("Run Screen SN"=w2178, "Specified SNs"=w2179, "Data"=w2185, "Profile"=w2175) -> ("Next SN"=w2184:string, "Untested SNs"=w2172:string[], "Tested SNs"=w2174:string[])  [unwired: 9 in]
        n1119 = call "SN Sort.vi"("Array In"=w2172) -> ("Array Out"=w2171:string[])  [unwired: 14 in]
        n1120 = call "SN Sort.vi"("Array In"=w2174) -> ("Array Out"=w2173:string[])  [unwired: 14 in]
        n1121 = Insert Into Array(array=w2183, index (col)=w2182, new element=w2171) -> (w2180:string[][])  [unwired: 1 in]
        n1122 = Insert Into Array(array=w2183, index (col)=w2182, new element=w2173) -> (w2181:string[][])  [unwired: 1 in]
        n1123 = local write "Next Serial Number"(w2184) -> ()
        n1124 = local write "Untested Serial Numbers"(w2180) -> ()
        n1125 = local write "Tested Serial Numbers"(w2181) -> ()
        n1126 = Bundle By Name(cluster=w2177, "Untested SNs"=w2171, "Tested SNs"=w2173) -> (w2176:T15)
      }
      frame "PS Abler" {
        w2187 = "\u0000\u0000\u0000\bPSenable\u0000\u0000\u0000\u0001\u0000"  # PS Disable
        w2188 = "\u0000\u0000\u0000\bPSenable\u0000\u0000\u0000\u0001\u0001"  # PS Enable
        w2201 = 4  # Command
        # "For a brushed pump Solenoid Stop? is False so the PS\nwill be enabled whenever test or manual mode is active"
        # "IF it is in test or manual mode\n\nAND the controller does not have to be stopped by a solenoid\n          OR the command does not equal the stop command\n          OR the indirect flow or speed is not zero\n\nTHEN enable the solenoid on the output of the power supply"
        n1127 = Unbundle By Name(w2204) -> ("Controller.Solenoid Stop?"=w2203:bool, "CommandCluster.SP3"=w2196:dbl, "CommandCluster.Para3"=w2202:i32, "Controller.Stop Command"=w2193:dbl)
        n1128 = Not Equal?(x=w2202, y=w2201) -> (x != y?=w2200:bool)
        n1129 = local read "pb.StartManual"() -> (w2197:bool)
        n1130 = local read "pb.StartTest"() -> (w2198:bool)
        n1131 = Not Equal To 0?(x=w2196) -> (x != 0?=w2194:bool)
        n1132 = Not Equal?(x=w2196, y=w2193) -> (x != y?=w2195:bool)
        n1133 = Select(t=w2194, s=w2200, f=w2195) -> (s? t:f=w2199:bool)
        n1134 = Or(x=w2198, y=w2197) -> (x .or. y?=w2205:bool)
        n1135 = Compound Arithmetic op=OR(invert w2203, w2199) -> (w2206:bool)
        n1136 = And(x=w2205, y=w2206) -> (x .and. y?=w2189:bool)
        n1137 = disable-structure shown="Disabled" {
          frame Disabled {
            (unwired) "\u0000\u0000\u0000\bPSenable\u0000\u0000\u0000\u0001\u0000"  # PS Disable
            (unwired) "\u0000\u0000\u0000\bPSenable\u0000\u0000\u0000\u0001\u0001"  # PS Enable
            # "Equals"
            # "Equals"
            n1138 = Flatten To String(anything=TRUE) -> (data string=w2212:string)  [unwired: 3 in, 2 out]
            n1139 = Flatten To String(anything=FALSE) -> (data string=w2211:string)  [unwired: 3 in, 2 out]
            n1140 = Bundle("data string"="PSenable", "data string"=w2212) -> (w2215:T32)  [unwired: 1 in]
            n1141 = Bundle("data string"="PSenable", "data string"=w2211) -> (w2208:T32)  [unwired: 1 in]
            n1142 = Flatten To String(anything=w2215) -> ()  [unwired: 3 in, 3 out]
            n1143 = Flatten To String(anything=w2208) -> ()  [unwired: 3 in, 3 out]
          }
          frame Enabled {
          }
        }
        n1144 = Select(t=w2188, s=w2189, f=w2187) -> (s? t:f=w2192:string)
        n1145 = call "PC Send Event.vi"("PC Send Command"=PCsend_RTrecv_CMD."PSenable", "Mode"=Event_Mode."Set", "Flattened Data"=w2192) -> ()  [unwired: 11 in, 2 out]
      }
      frame "Free Flow" {
        w2226 = T2."Command" ("Parameter 3")
        w2228 = i32[] [] ("Disabled Items []")
        w2233 = enum16{"Voltage", "Pressure", "Flow", "Speed"}."Pressure" ("Parameter 2")
        w2232 = T3."Voltage" ("Parameter 1")
        n1146 = Unbundle By Name(w2235) -> ("StandConfigCluster.Init Free Flow"=w2239:dbl, "StandConfigCluster.Free Flow Voltage"=w2230:dbl, "StandConfigCluster.Free Flow Pressure"=w2231:dbl, "CommandCluster"=w2234:T6, "Controller.Low Command"=w2225:dbl, "Controller.High Command"=w2224:dbl)
        n1147 = Get Date/Time In Seconds() -> (seconds since 1Jan1904=w2240:timestamp)
        n1148 = To Double Precision Float(number=w2240) -> (double precision float=w2238:dbl)
        n1149 = Add(x=w2225, y=w2224) -> (x+y=w2223:dbl)
        n1150 = Add(x=w2238, y=w2239) -> (x+y=w2237:dbl)
        n1151 = Divide(x=w2223, y=2.0) -> (x/y=w2221:dbl)
        n1152 = property on="Parameter 1" class="Enum (strict)"("Disabled Items []"=w2228) -> ()  [unwired: 2 in, 2 out]
        n1153 = local write "Parameter 1"(w2232) -> ()
        n1154 = local write "Setpoint1"(w2230) -> ()
        n1155 = local write "Parameter 2"(w2233) -> ()
        n1156 = local write "Setpoint2"(w2231) -> ()
        n1157 = local write "Parameter 3"(w2226) -> ()
        n1158 = local write "Setpoint3"(w2221) -> ()
        n1159 = Insert Into Array(array=w2220, index=0, new element=string[] ["Write Command"]) -> (w2219:string[])
        n1160 = property on="Parameter 2" class="Enum (strict)"("Disabled Items []"=w2228) -> ()  [unwired: 2 in, 2 out]
        n1161 = property on="Parameter 3" class="Enum (strict)"("Disabled Items []"=i32[] [0, 1]) -> ()  [unwired: 2 in, 2 out]
        n1162 = Bundle By Name(cluster=w2234, "Para1"=w2232, "SP1"=w2230, "Para2"=w2233, "SP2"=w2231, "Para3"=w2226, "SP3"=w2221) -> (w2216:T6)
        n1163 = Bundle By Name(cluster=w2235, "Free Flow"=TRUE, "WaitingData"=FALSE, "StepTimeLimit"=w2237, "CommandCluster"=w2216, "DesiredParameters"=w2216) -> (w2241:T15)
      }
      frame "Start Test" {
        w2265 = T17."Enabled" ("Disabled")
        # "Enable Pause Test button now\nthat the free flow is over"
        # "The Start Test button first checks that the parameter information chart is correct if that is correct it checks the serial number slots to make sure one was assigned, then it comes here"
        n1164 = Get Date/Time In Seconds() -> (seconds since 1Jan1904=w2252:timestamp)
        n1165 = To Double Precision Float(number=w2252) -> (double precision float=w2250:dbl)
        n1166 = Round Toward -Infinity(1:w2250) -> (0:w2251:dbl)
        n1167 = To Quad Integer(1:w2251) -> (0:w2243:i64)
        n1168 = Unbundle By Name(w2253) -> ("Controller.Controller?"=w2261:bool, "CommandCluster"=w2263:T6, "Parameters"=w2264:string[][], "StandConfigCluster.Stable Count"=w2260:dbl, "StandConfigCluster.Parameter Timeout"=w2259:dbl)
        n1169 = local read "TestType"() -> (w2262:enum32{"Flow", "Test", "Hot\nFuel"})
        n1170 = call "Test Step Parser.vi"("Controller?"=w2261, "LastDataTime"=w2243, "Enum.Radio"=w2262, "Step In"=0, "CMD Cluster IN"=w2263, "Profile"=w2264, "Stable Count"=w2260, "Parameter Timeout"=w2259) -> ("StepDataActive"=w2258:dbl, "StepTimeLimit"=w2255:dbl, "Step Out"=w2257:i32, "CMD Cluster Out"=w2242:T6)  [unwired: 4 in]
        n1171 = Unbundle By Name(w2242) -> ("Para1"=w2268:i32, "SP1"=w2271:dbl, "Para2"=w2267:i32, "SP2"=w2270:dbl, "Para3"=w2266:i32, "SP3"=w2269:dbl)
        n1172 = Bundle By Name(cluster=w2253, "Free Flow"=FALSE, "LastDataTime"=w2243, "WaitingData"=TRUE, "StepDataActive"=w2258, "StepTimeLimit"=w2255, "StepIndex"=w2257, "CommandCluster"=w2242, "DesiredParameters"=w2242) -> (w2254:T15)
        n1173 = Insert Into Array(array=w2247, index=0, new element=string[] ["Write Command"]) -> (w2246:string[])
        n1174 = local write "Parameter 1"(w2268) -> ()
        n1175 = local write "Setpoint1"(w2271) -> ()
        n1176 = local write "Parameter 2"(w2267) -> ()
        n1177 = local write "Setpoint2"(w2270) -> ()
        n1178 = local write "Parameter 3"(w2266) -> ()
        n1179 = local write "Setpoint3"(w2269) -> ()
        n1180 = property on="pb.Pause Test" class="Bool (strict)"("DisabledEnum"=w2265) -> ()  [unwired: 2 in, 2 out]
        n1181 = property on="pb.Skip Step" class="Bool"("DisabledEnum"=w2265) -> ()  [unwired: 2 in, 2 out]
      }
      frame "Next Step" {
        n1182 = Unbundle By Name(w2296) -> ("LastDataTime"=w2283:i64, "Controller.Controller?"=w2284:bool, "StepIndex"=w2285:i32, "CommandCluster"=w2287:T6, "Parameters"=w2288:string[][], "StandConfigCluster.Stable Count"=w2282:dbl, "StandConfigCluster.Parameter Timeout"=w2281:dbl)
        n1183 = local read "TestType"() -> (w2286:enum32{"Flow", "Test", "Hot\nFuel"})
        n1184 = call "Test Step Parser.vi"("Controller?"=w2284, "LastDataTime"=w2283, "Enum.Radio"=w2286, "Step In"=w2285, "CMD Cluster IN"=w2287, "Profile"=w2288, "Stable Count"=w2282, "Parameter Timeout"=w2281) -> ("StepDataActive"=w2280:dbl, "StepTimeLimit"=w2277:dbl, "Step Out"=w2279:i32, "CMD Cluster Out"=w2272:T6)  [unwired: 4 in]
        n1185 = Unbundle By Name(w2272) -> ("Para1"=w2291:i32, "SP1"=w2294:dbl, "Para2"=w2290:i32, "SP2"=w2293:dbl, "Para3"=w2289:i32, "SP3"=w2292:dbl)
        n1186 = Insert Into Array(array=w2276, index=0, new element=string[] ["Write Command"]) -> (w2275:string[])
        n1187 = Bundle By Name(cluster=w2296, "WaitingData"=TRUE, "StepDataActive"=w2280, "StepTimeLimit"=w2277, "StepIndex"=w2279, "CommandCluster"=w2272, "DesiredParameters"=w2272) -> (w2295:T15)
        n1188 = local write "Parameter 1"(w2291) -> ()
        n1189 = local write "Setpoint1"(w2294) -> ()
        n1190 = local write "Parameter 2"(w2290) -> ()
        n1191 = local write "Setpoint2"(w2293) -> ()
        n1192 = local write "Parameter 3"(w2289) -> ()
        n1193 = local write "Setpoint3"(w2292) -> ()
      }
      frame "Part Change" {
        n1194 = local read "Next Serial Number"() -> (w2303:string)
        n1195 = Unbundle By Name(w2302) -> ("Untested SNs"=w2300:string[], "TestRunning?"=w2297:bool)
        n1196 = call "Remove Tildes (String).vi"("String In"=w2303) -> ("String Out"=w2304:string)  [unwired: 2 in]
        n1197 = Empty String/Path?(string/path=w2304) -> (empty?=w2305:bool)
        n1198 = case shown="False" w2305 {
          tunnel: w2304 -> [w2314 _]
          tunnel: w2302 -> [w2318 w2332]
          tunnel: [w2317 w2332] -> w2301
          tunnel: w2299 -> [w2316 w2331]
          tunnel: [w2315 w2331] -> w2298
          tunnel: w2300 -> [w2311 _]
          tunnel: w2297 -> [w2307 _]
          frame False {
            n1199 = flat-sequence {
              tunnel: [w2319] -> w2308
              frame #0 {
                w2319 = T21."Run Screen" ("Mode")
                n1200 = call "Tab Handler.vi"("Mode"=w2319) -> ()  [unwired: 15 in]
              }
            }
            n1201 = Search 1D Array(1D array=w2311, element=w2314) -> (index of element=w2310:i32)  [unwired: 1 in]
            n1202 = case shown="True" w2307 {
              tunnel: w2316 -> [w2324 w2330]
              tunnel: [w2324 w2329] -> w2315
              tunnel: w2308 -> [_ _]
              frame False {
              }
              frame True {
                w2325 = T17."Disabled and Grayed Out" ("Disabled")
                # "Cannot allow pause test to be\npressed when in free flow"
                n1203 = call "Tab Handler.vi"("Mode"=T21."Lock All") -> ()  [unwired: 15 in]
                n1204 = Insert Into Array(array=w2330, index=0, new element="Free Flow" ("new element/subarray")) -> (w2329:string[])
                n1205 = property on="pb.Pause Test" class="Bool (strict)"("DisabledEnum"=w2325) -> ()  [unwired: 2 in, 2 out]
                n1206 = property on="pb.Skip Step" class="Bool"("DisabledEnum"=w2325) -> ()  [unwired: 2 in, 2 out]
              }
            }
            n1207 = Not Equal?(x=w2310, y=-1) -> (x != y?=w2312:bool)
            n1208 = local write "Screen"(T1."Run Screen" ("Screen")) -> ()
            n1209 = case shown="True" w2312 {
              tunnel: w2311 -> [w2320 w2323]
              tunnel: w2310 -> [_ w2322]
              tunnel: [w2320 w2321] -> w2309
              frame False {
              }
              frame True {
                n1210 = Delete From Array(array=w2323, index=w2322) -> (array with subset deleted=w2321:string[])  [unwired: 1 in, 1 out]
              }
            }
            n1211 = Bundle By Name(cluster=w2318, "Untested SNs"=w2309, "Serial Number"=w2314) -> (w2317:T15)
            n1212 = local write "Serial Number"(w2314) -> ()
          }
          frame True {
          }
        }
      }
      frame "Next Part" {
        # "Take the next item in untested serial numbers and place it in next serial number and go to the part change screen"
        n1213 = Unbundle By Name(w2344) -> ("Untested SNs"=w2343:string[], "Tested SNs"=w2339:string[])
        n1214 = local read "Serial Number"() -> (w2346:string)
        n1215 = Search 1D Array(1D array=w2343, element=w2346) -> (index of element=w2347:i32)  [unwired: 1 in]
        n1216 = Delete From Array(array=w2343, index=w2347) -> (array with subset deleted=w2342:string[])  [unwired: 1 in, 1 out]
        n1217 = Array Size(array=w2339) -> (size(s)=w2348:i32)
        n1218 = Index Array(array=w2342, index=0 ("index (row)")) -> (element=w2349:string)
        n1219 = Insert Into Array(array=w2339, index=w2348, new element=w2346) -> (w2337:string[])
        n1220 = Build Array(w2342) -> (w2341:string[][])
        n1221 = Build Array(w2337) -> (w2338:string[][])
        n1222 = Transpose 2D Array(2D array=w2341) -> (transposed array=w2340:string[][])
        n1223 = Transpose 2D Array(2D array=w2338) -> (transposed array=w2336:string[][])
        n1224 = property on="pb.select SN" class="Bool"("Key Focus"=TRUE) -> ()  [unwired: 2 in, 2 out]
        n1225 = call "Tab Handler.vi"("Mode"=T21."Other Tab") -> ()  [unwired: 15 in]
        n1226 = local write "Untested Serial Numbers"(w2340) -> ()
        n1227 = local write "Next Serial Number"(w2349) -> ()
        n1228 = local write "Tested Serial Numbers"(w2336) -> ()
        n1229 = local write "Screen"(T1."Part Change" ("Screen")) -> ()
        n1230 = Bundle By Name(cluster=w2344, "Untested SNs"=w2342, "Tested SNs"=w2337) -> (w2345:T15)
      }
      frame "Pause Test" {
        w2377 = enum16{"Voltage", "Pressure", "Flow", "Speed"}[] [enum."Pressure", enum."Flow", enum."Speed"] items=["Voltage", "Pressure", "Flow", "Speed"]
        w2365 = FALSE ("TestRunning?")
        w2380 = 0.0 ("SP1")
        w2364 = T17."Enabled" ("Disabled")
        n1231 = Unbundle By Name(w2382) -> ("LastDataSet"=w2373:string[], "StepIndex"=w2368:i32, "CommandCluster"=w2358:T6, "Controller.Stop Command"=w2361:dbl)
        n1232 = local read "Parameter 1"() -> (w2363:T3)
        n1233 = local read "Parameter 2"() -> (w2362:enum16{"Voltage", "Pressure", "Flow", "Speed"})
        n1234 = Equal?(x=T3."Deadhead", y=w2363) -> (x = y?=w2376:bool)
        n1235 = Build Array(w2363) -> (w2378:T26)
        n1236 = Build Array(w2362) -> (w2375:enum16{"Voltage", "Pressure", "Flow", "Speed"}[])
        n1237 = call "Handle Parameter 3 Control.vi"("Parameter 1"=w2363, "Parameter 2"=w2362, "Stop Command"=w2361, "Last Command"=w2361) -> ("Parameter 3"=w2359:i32, "Command  Out"=w2360:dbl)  [unwired: 9 in, 1 out]
        n1238 = Select(t=w2377, s=w2376, f=w2378) -> (s? t:f=w2379:T26)
        n1239 = local write "Setpoint1"(w2380) -> ()
        n1240 = local write "Setpoint2"(w2380) -> ()
        n1241 = Bundle By Name(cluster=w2358, "SP1"=w2380, "SP2"=w2380, "Para3"=w2359, "SP3"=w2360) -> (w2352:T6)
        n1242 = local write "Setpoint3"(w2360) -> ()
        n1243 = property on="Parameter 2" class="Enum (strict)"("Disabled Items []"=w2379) -> ()  [unwired: 2 in, 2 out]
        n1244 = property on="Parameter 1" class="Enum (strict)"("Disabled Items []"=w2375) -> ()  [unwired: 2 in, 2 out]
        n1245 = Index Array(array=w2373, index=11) -> (element=w2371:string)
        n1246 = Decrement(x=w2368) -> (x-1=w2369:i32)
        n1247 = Decimal String To Number(string=w2371) -> (number=w2370:i32)  [unwired: 2 in, 1 out]
        n1248 = Equal?(x=w2370, y=w2369) -> (x = y?=w2367:bool)
        n1249 = Select(t=w2369, s=w2367, f=w2368) -> (s? t:f=w2366:i32)
        n1250 = local write "Running?"(w2365) -> ()
        n1251 = Bundle By Name(cluster=w2382, "StepIndex"=w2366, "TestRunning?"=w2365, "WaitingData"=w2365, "CommandCluster"=w2352, "DesiredParameters"=w2352) -> (w2381:T15)
        n1252 = Insert Into Array(array=w2356, index=0, new element=string[] ["Write Command"]) -> (w2355:string[])
        n1253 = call "Tab Handler.vi"("Mode"=T21."Run Screen") -> ()  [unwired: 15 in]
        n1254 = property on="Parameter 1" class="Enum (strict)"("DisabledEnum"=w2364) -> ()  [unwired: 2 in, 2 out]
        n1255 = property on="Setpoint1" class="DigNum (strict)"("DisabledEnum"=w2364) -> ()  [unwired: 2 in, 2 out]
        n1256 = property on="Parameter 2" class="Enum (strict)"("DisabledEnum"=w2364) -> ()  [unwired: 2 in, 2 out]
        n1257 = property on="Setpoint2" class="DigNum (strict)"("DisabledEnum"=w2364) -> ()  [unwired: 2 in, 2 out]
        n1258 = property on="Parameter 3" class="Enum (strict)"("DisabledEnum"=w2364) -> ()  [unwired: 2 in, 2 out]
        n1259 = property on="Setpoint3" class="DigNum (strict)"("DisabledEnum"=w2364) -> ()  [unwired: 2 in, 2 out]
        n1260 = property on="Serial Number" class="Str"("DisabledEnum"=w2364) -> ()  [unwired: 2 in, 2 out]
      }
      frame "Resume Test" {
        w2392 = TRUE ("WaitingData")
        w2412 = T17."Disabled" ("Disabled")
        w2414 = i32[] [] ("Disabled Items []")
        n1261 = call "Tab Handler.vi"("Mode"=T21."Lock All") -> ()  [unwired: 15 in]
        n1262 = property on="Parameter 1" class="Enum (strict)"("DisabledEnum"=w2412) -> ()  [unwired: 2 in, 2 out]
        n1263 = property on="Setpoint1" class="DigNum (strict)"("DisabledEnum"=w2412) -> ()  [unwired: 2 in, 2 out]
        n1264 = property on="Parameter 2" class="Enum (strict)"("DisabledEnum"=w2412) -> ()  [unwired: 2 in, 2 out]
        n1265 = property on="Setpoint2" class="DigNum (strict)"("DisabledEnum"=w2412) -> ()  [unwired: 2 in, 2 out]
        n1266 = property on="Parameter 3" class="Enum (strict)"("DisabledEnum"=w2412) -> ()  [unwired: 2 in, 2 out]
        n1267 = property on="Setpoint3" class="DigNum (strict)"("DisabledEnum"=w2412) -> ()  [unwired: 2 in, 2 out]
        n1268 = property on="Serial Number" class="Str"("DisabledEnum"=w2412) -> ()  [unwired: 2 in, 2 out]
        n1269 = Get Date/Time In Seconds() -> (seconds since 1Jan1904=w2391:timestamp)
        n1270 = To Double Precision Float(number=w2391) -> (double precision float=w2389:dbl)
        n1271 = Round Toward -Infinity(1:w2389) -> (0:w2390:dbl)
        n1272 = To Quad Integer(1:w2390) -> (0:w2388:i64)
        n1273 = Unbundle By Name(w2394) -> ("Controller.Controller?"=w2400:bool, "StepIndex"=w2401:i32, "CommandCluster"=w2403:T6, "Parameters"=w2404:string[][], "StandConfigCluster.Stable Count"=w2399:dbl, "StandConfigCluster.Parameter Timeout"=w2398:dbl)
        n1274 = local read "TestType"() -> (w2402:enum32{"Flow", "Test", "Hot\nFuel"})
        n1275 = call "Test Step Parser.vi"("Controller?"=w2400, "LastDataTime"=w2388, "Enum.Radio"=w2402, "Step In"=w2401, "CMD Cluster IN"=w2403, "Profile"=w2404, "Stable Count"=w2399, "Parameter Timeout"=w2398) -> ("StepDataActive"=w2397:dbl, "StepTimeLimit"=w2395:dbl, "Step Out"=w2396:i32, "CMD Cluster Out"=w2383:T6)  [unwired: 4 in]
        n1276 = Unbundle By Name(w2383) -> ("Para1"=w2407:i32, "SP1"=w2410:dbl, "Para2"=w2406:i32, "SP2"=w2409:dbl, "Para3"=w2405:i32, "SP3"=w2408:dbl)
        n1277 = Bundle By Name(cluster=w2394, "LastDataTime"=w2388, "TestRunning?"=w2392, "WaitingData"=w2392, "StepDataActive"=w2397, "StepTimeLimit"=w2395, "StepIndex"=w2396, "CommandCluster"=w2383, "DesiredParameters"=w2383) -> (w2393:T15)
        n1278 = Insert Into Array(array=w2385, index=0, new element=string[] ["Write Command"]) -> (w2384:string[])
        n1279 = local write "Parameter 1"(w2407) -> ()
        n1280 = local write "Setpoint1"(w2410) -> ()
        n1281 = local write "Parameter 2"(w2406) -> ()
        n1282 = local write "Setpoint2"(w2409) -> ()
        n1283 = local write "Parameter 3"(w2405) -> ()
        n1284 = local write "Setpoint3"(w2408) -> ()
        n1285 = local write "Running?"(w2392) -> ()
        n1286 = property on="Parameter 1" class="Enum (strict)"("Disabled Items []"=w2414) -> ()  [unwired: 2 in, 2 out]
        n1287 = property on="Parameter 2" class="Enum (strict)"("Disabled Items []"=w2414) -> ()  [unwired: 2 in, 2 out]
        n1288 = property on="Parameter 3" class="Enum (strict)"("Disabled Items []"=i32[] [0, 1]) -> ()  [unwired: 2 in, 2 out]
      }
      frame "Skip Step" {
        n1289 = Get Date/Time In Seconds() -> (seconds since 1Jan1904=w2417:timestamp)
        n1290 = To Double Precision Float(number=w2417) -> (double precision float=w2416:dbl)
        n1291 = Decrement(x=w2416) -> (x-1=w2415:dbl)
        n1292 = Bundle By Name(cluster=w2420, "StepDataActive"=w2415, "StepTimeLimit"=w2415, "WaitingData"=TRUE) -> (w2419:T15)
      }
      frame "Stop Test" {
        w2430 = T17."Disabled and Grayed Out" ("Disabled")
        w2441 = enum16{"Voltage", "Pressure", "Flow", "Speed"}[] [enum."Pressure", enum."Flow", enum."Speed"] items=["Voltage", "Pressure", "Flow", "Speed"]
        w2434 = FALSE ("TestRunning?")
        w2444 = cluster{u32, u32}[] [{1985280, 1985280}, {6618880, 6618880}, {1985280, 1985280}, {6618880, 6618880}]  # Original Colors
        w2446 = 0.0 ("SP1")
        w2431 = T17."Enabled" ("Disabled")
        # "resetting this so that there is no\npause test option during free flow"
        # "setting free flow to false has\nto be done in case the test was\nstopped while still in free flow"
        n1293 = Unbundle By Name(w2445) -> ("CommandCluster"=w2433:T6, "Controller.Stop Command"=w2428:dbl)
        n1294 = flat-sequence {
          tunnel: w2428 -> [w2449]
          tunnel: [w2449] -> w2427
          frame #0 {
            n1295 = local write "Parameter 3"(T2."Command" ("Parameter 3")) -> ()
          }
        }
        n1296 = local read "Parameter 1"() -> (w2437:T3)
        n1297 = local read "Parameter 2"() -> (w2436:enum16{"Voltage", "Pressure", "Flow", "Speed"})
        n1298 = property on="pb.Pause Test" class="Bool (strict)"("DisabledEnum"=w2430) -> ()  [unwired: 2 in, 2 out]
        n1299 = property on="pb.Skip Step" class="Bool"("DisabledEnum"=w2430) -> ()  [unwired: 2 in, 2 out]
        n1300 = Equal?(x=T3."Deadhead", y=w2437) -> (x = y?=w2440:bool)
        n1301 = Build Array(w2437) -> (w2442:T26)
        n1302 = Build Array(w2436) -> (w2439:enum16{"Voltage", "Pressure", "Flow", "Speed"}[])
        n1303 = call "Handle Parameter 3 Control.vi"("Parameter 1"=w2437, "Parameter 2"=w2436, "Stop Command"=w2427, "Last Command"=w2427) -> ("Parameter 3"=w2429:i32, "Command  Out"=w2435:dbl)  [unwired: 9 in, 1 out]
        n1304 = local write "Setpoint1"(w2446) -> ()
        n1305 = local write "Setpoint2"(w2446) -> ()
        n1306 = local write "Setpoint3"(w2435) -> ()
        n1307 = Bundle By Name(cluster=w2433, "SP1"=w2446, "SP2"=w2446, "Para3"=w2429, "SP3"=w2435) -> (w2422:T6)
        n1308 = Select(t=w2441, s=w2440, f=w2442) -> (s? t:f=w2443:T26)
        n1309 = property on="Parameter 2" class="Enum (strict)"("Disabled Items []"=w2443) -> ()  [unwired: 2 in, 2 out]
        n1310 = property on="Parameter 1" class="Enum (strict)"("Disabled Items []"=w2439) -> ()  [unwired: 2 in, 2 out]
        n1311 = local write "Running?"(w2434) -> ()
        n1312 = local write "pb.StartTest"(w2434) -> ()
        n1313 = Insert Into Array(array=w2424, index=0, new element=string[] ["Write Command"]) -> (w2423:string[])
        n1314 = Bundle By Name(cluster=w2445, "StepIndex"=0, "TestRunning?"=w2434, "WaitingData"=w2434, "Free Flow"=w2434, "CommandCluster"=w2422, "DesiredParameters"=w2422) -> (w2447:T15)
        n1315 = call "Tab Handler.vi"("Mode"=T21."Run Screen") -> ()  [unwired: 15 in]
        n1316 = property on="Stabilized?" class="Bool (strict)"("Colors [4]"=w2444) -> ()  [unwired: 2 in, 2 out]
        n1317 = property on="Parameter 1" class="Enum (strict)"("DisabledEnum"=w2431) -> ()  [unwired: 2 in, 2 out]
        n1318 = property on="Setpoint1" class="DigNum (strict)"("DisabledEnum"=w2431) -> ()  [unwired: 2 in, 2 out]
        n1319 = property on="Parameter 2" class="Enum (strict)"("DisabledEnum"=w2431) -> ()  [unwired: 2 in, 2 out]
        n1320 = property on="Setpoint2" class="DigNum (strict)"("DisabledEnum"=w2431) -> ()  [unwired: 2 in, 2 out]
        n1321 = property on="Parameter 3" class="Enum (strict)"("DisabledEnum"=w2431) -> ()  [unwired: 2 in, 2 out]
        n1322 = property on="Setpoint3" class="DigNum (strict)"("DisabledEnum"=w2431) -> ()  [unwired: 2 in, 2 out]
        n1323 = property on="Serial Number" class="Str"("DisabledEnum"=w2431) -> ()  [unwired: 2 in, 2 out]
        n1324 = property on="pb.StartManual" class="Bool (strict)"("DisabledEnum"=w2431) -> ()  [unwired: 2 in, 2 out]
      }
      frame "Freeze Screen" {
        n1325 = control-ref of="This VI"() -> (w2453:refnum<vi>)
        n1326 = property class="VI"(reference=w2453) -> ("Panel"=w2452:refnum<vi>)  [unwired: 1 in, 2 out]
        n1327 = property class="Pnl"(reference=w2452, "DeferPanUpdts"=TRUE ("Defer Panel Updates")) -> ()  [unwired: 1 in, 2 out]
      }
      frame "Store Data" {
        w2478 = FALSE
        # "Was thinking I could look at if the values were on both or\nonly one side of SP to know if it was Unstable or Unreached"
        # "Addition of setting waiting data to false\nif it is manual it should already be false\nand stops the constant looping in test mode"
        n1328 = Unbundle By Name(w2483) -> ("Controller.Command Step"=w2459:dbl, "table.Data"=w2461:string[][], "SkipStep"=w2464:bool, "StepIndex"=w2462:i32, "LastDataRow"=w2468:i32, "TestRunning?"=w2467:bool, "DataCluster"=w2471:T13, "Controller.Controller?"=w2466:bool, "Serial Number"=w2465:string, "DesiredParameters"=w2457:T6, "Stability Cluster"=w2456:T5, "Serial Numbers"=w2470:string[], "ValidFile?"=w2469:bool)
        n1329 = control-ref of="table.Data"() -> (w2493:refnum<vi>)
        n1330 = Increment(x=w2468) -> (x+1=w2480:i32)
        n1331 = Search 1D Array(1D array=w2470, element=w2465) -> (index of element=w2487:i32)  [unwired: 1 in]
        n1332 = property class="Tbl (strict)"(reference=w2493) -> ("Selection Start"=w2492:T19)  [unwired: 1 in, 2 out]
        n1333 = local read "Steps"() -> (w2463:u16)
        n1334 = Equal?(x=w2487, y=-1) -> (x = y?=w2477:bool)
        n1335 = And(x=w2477, y=w2469) -> (x .and. y?=w2476:bool)
        n1336 = Unbundle By Name(w2492) -> ("Row"=w2474:i32)
        n1337 = Array Size(array=w2461) -> (size(s)=w2495:i32[])
        n1338 = call "Create Data Row.vi"("TestRunning?"=w2467, "Steps"=w2463, "StepIndex"=w2462, "SkipStep"=w2464, "DataCluster"=w2471, "CMD Step"=w2459, "Controller?"=w2466, "Serial Number"=w2465, "DesiredParameters"=w2457, "Stability Cluster"=w2456) -> ("DataRowWithParameters"=w2472:string[], "DataRow"=w2460:string[], "LastDataTime"=w2458:i64)  [unwired: 3 in]
        n1339 = Increment(x=w2474) -> (x+1=w2473:i32)
        n1340 = Index Array(array=w2495, index=0) -> (element=w2475:i32)
        n1341 = Not Equal To 0?(x=w2475) -> (x != 0?=w2490:bool)
        n1342 = Select(t=w2473, s=w2490, f=w2475) -> (s? t:f=w2491:i32)
        "StoredDataRow" <- w2491
        n1343 = Select(t=w2475, s=w2490, f=1) -> (s? t:f=w2488:i32)
        n1344 = call "Data Table Handler.vi"("TableRef"=w2493, "DesiredRow"=w2491, "TableRows"=w2488) -> ("RowIndex"=w2481:i32)  [unwired: 12 in]
        n1345 = Insert Into Array(array=w2461, index (row)=w2481, new element=w2472) -> (w2479:string[][])  [unwired: 1 in]
        n1346 = local write "table.Data"(w2479) -> ()
        n1347 = case shown="True" w2476 {
          tunnel: w2485 -> [w2504 w2521]
          tunnel: [w2504 w2520] -> w2484
          tunnel: w2483 -> [w2503 w2515]
          tunnel: [w2502 w2514] -> w2482
          tunnel: w2480 -> [w2501 w2516]
          tunnel: w2460 -> [w2500 w2517]
          tunnel: w2479 -> [w2499 w2518]
          tunnel: w2465 -> [_ w2512]
          tunnel: w2470 -> [_ w2513]
          tunnel: w2478 -> [w2498 w2509]
          tunnel: w2478 -> [w2497 w2508]
          tunnel: w2458 -> [w2496 w2506]
          frame False {
            n1348 = Bundle By Name(cluster=w2503, "table.Data"=w2499, "LastDataSet"=w2500, "LastDataRow"=w2501, "WaitingData"=w2498, "SkipStep"=w2497, "LastDataTime"=w2496) -> (w2502:T15)
          }
          frame True {
            n1349 = Insert Into Array(array=w2513, index=0, new element=w2512) -> (w2510:string[])
            n1350 = Sort 1D Array(array=w2510) -> (sorted array=w2505:string[])
            n1351 = Bundle By Name(cluster=w2515, "table.Data"=w2518, "LastDataSet"=w2517, "LastDataRow"=w2516, "WaitingData"=w2509, "SkipStep"=w2508, "LastDataTime"=w2506, "Serial Numbers"=w2505) -> (w2514:T15)
            n1352 = Insert Into Array(array=w2521, index=0, new element=string[] ["Save Test Config"]) -> (w2520:string[])
          }
        }
      }
      frame "Find Stats" {
        n1353 = Unbundle By Name(w2535) -> ("StatBundle"=w2526:T7, "Controller.Command Step"=w2523:dbl, "DesiredParameters"=w2522:T6, "LastDataSet"=w2524:string[], "Controller.Controller?"=w2525:bool, "table.Data"=w2529:string[][], "CurrentDataFile"=w2532:path, "ValidFile?"=w2531:bool)
        n1354 = local read "StoredDataRow"() -> (w2530:i32)
        n1355 = call "Handle Stat Sections.vi"("StatBundle In"=w2526, "CMD Step"=w2523, "DesiredParameters"=w2522, "LastDataSet"=w2524, "Controller?"=w2525) -> ("StatBundle Out"=w2528:T7)  [unwired: 10 in]
        n1356 = call "Stat Bundles to Table.vi"("StatBundle"=w2528) -> ("table.Stats"=w2527:string[][])  [unwired: 14 in]
        n1357 = case shown="True" w2531 {
          tunnel: w2532 -> [_ w2538]
          tunnel: w2527 -> [_ w2536]
          frame False {
          }
          frame True {
            n1358 = call "Filepath 2 Hidden Files.vi"("DataFilePath"=w2538, "Enum"=enum16{"Data", "Stats", "Specs"}."Stats") -> ("HiddenFilePath"=w2537:path)  [unwired: 13 in]
            n1359 = Array Subset(array=w2536, index (col)=0 ("index"), length (col)=13 ("length")) -> (w2541:string[][])  [unwired: 2 in]
            n1360 = call-poly <vilib>:"Write To Spreadsheet File.vi"("delimiter (\\t)"="~" ("delimiter (\\t)"), "2D data"=w2541, "file path (dialog if empty)"=w2537) -> ()  [unwired: 5 in, 1 out]
          }
        }
        n1361 = local write "table.Stats"(w2527) -> ()
        n1362 = call "Full Table Handler.vi"("table.Data"=w2529, "table.Stats"=w2527, "Data Row Index"=w2530) -> ()  [unwired: 13 in]
        n1363 = Bundle By Name(cluster=w2535, "StatBundle"=w2528, "table.Stats"=w2527) -> (w2534:T15)
      }
      frame "Verify Stats" {
        # "Update bundle to calculated\nbut not display in case they\nare different then they can\nbe corrected or left as is"
        # "Because hot fuel has no stats"
        n1364 = Unbundle By Name(w2562) -> ("table.Stats"=w2546:string[][], "StatBundle"=w2557:T7)
        n1365 = call "Stat Bundles to Table.vi"("StatBundle"=w2557) -> ("table.Stats"=w2545:string[][])  [unwired: 14 in]
        n1366 = Array Size(array=w2546) -> (size(s)=w2551:i32[])
        n1367 = Array Size(array=w2545) -> (size(s)=w2550:i32[])
        n1368 = Equal?(x=w2551, y=w2550) -> (x = y?=w2553:bool[])
        n1369 = And Array Elements(Boolean array=w2553) -> (logical AND=w2549:bool)
        n1370 = Not(x=w2549) -> (.not. x?=w2552:bool)
        n1371 = for {
          tunnel: w2546 -> [w2568] mode=indexing
          tunnel: w2545 -> [w2567] mode=indexing
          shift-right: [w2565] -> w2548
          shift-left: w2552 -> [w2566]
          stop <- w2565 stop-if-true
          n1372 = for {
            tunnel: w2568 -> [w2571] mode=indexing
            tunnel: w2567 -> [w2570] mode=indexing
            shift-right: [w2572] -> w2565
            shift-left: w2566 -> [w2573]
            stop <- w2572 stop-if-true
            n1373 = Not Equal?(x=w2571, y=w2570) -> (x != y?=w2569:bool)
            n1374 = Or(x=w2569, y=w2573) -> (x .or. y?=w2572:bool)
          }
        }
        n1375 = Empty Array?(array=w2546) -> (empty?=w2555:bool)
        n1376 = Empty Array?(array=w2545) -> (empty?=w2554:bool)
        n1377 = And(x=w2555, y=w2554) -> (x .and. y?=w2556:bool)
        n1378 = Select(t=FALSE, s=w2556, f=w2548) -> (s? t:f=w2559:bool)
        n1379 = local read "TestType"() -> (w2560:enum32{"Flow", "Test", "Hot\nFuel"})
        n1380 = case shown="\"Hot\\nFuel\"" w2560 {
          tunnel: w2545 -> [w2574 _]
          tunnel: w2559 -> [w2575 _]
          tunnel: [w2575 FALSE ("Invalid?")] -> w2544
          tunnel: [w2574 string[][] [] ("Stat Array Out")] -> w2558
          frame "Flow", "Test", Default {
          }
          frame "Hot\nFuel" {
          }
        }
        n1381 = case shown="True" w2544 {
          tunnel: w2564 -> [w2581 w2582]
          tunnel: [w2580 w2582] -> w2563
          frame True {
            n1382 = Insert Into Array(array=w2581, index=0, new element=string[] ["Thaw Screen", "Unset Cursor Busy", "Invalid Stats"]) -> (w2580:string[])
          }
          frame False {
          }
        }
        n1383 = Bundle By Name(cluster=w2562, "table.Stats"=w2558) -> (w2561:T15)
      }
      frame "Invalid Stats" {
        n1384 = Two Button Dialog(message="WARNING!\n\nThe loaded files Stat tab and the calculated stats do not match.\nThis could be from modifying the file outside this program.\nClicking continue will rewrite the Stat tab in the Excel file.", 2:"Continue" ("T button name (\"OK\")")) -> (T button?=w2587:bool)  [unwired: 1 in]
        n1385 = case shown="True" w2587 {
          tunnel: w2586 -> [w2594 w2601]
          tunnel: [w2594 w2600] -> w2585
          tunnel: w2584 -> [w2596 w2597]
          tunnel: [w2595 w2597] -> w2583
          frame False {
            w2591 = string[] []
            w2592 = string[][] []
            w2593 = "" ("Serial Number")
            n1386 = local write "Next Serial Number"(w2593) -> ()
            n1387 = local write "Serial Number"(w2593) -> ()
            n1388 = local write "table.Data"(w2592) -> ()
            n1389 = local write "table.Stats"(w2592) -> ()
            n1390 = local write "Parameters"(w2592) -> ()
            n1391 = local write "Serial Numbers"(w2592) -> ()
            n1392 = local write "Untested Serial Numbers"(w2592) -> ()
            n1393 = local write "Tested Serial Numbers"(w2592) -> ()
            n1394 = call "Test Config Update.vi"("Mode"=enum16{"Init", "Clear", "Update"}."Clear") -> ()  [unwired: 14 in, 1 out]
            n1395 = local write "File Location"(w2593) -> ()
            n1396 = local write "RS File Location"(w2593) -> ()
            n1397 = Bundle By Name(cluster=w2596, "Serial Number"=w2593, "table.Data"=w2592, "table.Stats"=w2592, "Parameters"=w2592, "Serial Numbers"=w2591, "Untested SNs"=w2591, "Tested SNs"=w2591) -> (w2595:T15)
          }
          frame True {
            n1398 = Insert Into Array(array=w2601, index=0, new element=string[] ["Correct Stats"]) -> (w2600:string[])
          }
        }
      }
      frame "Correct Stats" {
        w2608 = 0 ("index")
        # "The only way to get to the correct stats case is if there\nis ValidFile? so the stats will always get written here"
        n1399 = Unbundle By Name(w2605) -> ("Created/ModFiles"=w2603:cluster{"FilePath":path, "Save?":bool}[], "table.Data"=w2618:string[][], "CurrentDataFile"=w2611:path, "table.Stats"=w2614:string[][])
        n1400 = local write "table.Stats"(w2614) -> ()
        n1401 = Array Subset(array=w2614, index (col)=0 ("index"), length (col)=13 ("length")) -> (w2615:string[][])  [unwired: 2 in]
        n1402 = call "Filepath 2 Hidden Files.vi"("DataFilePath"=w2611, "Enum"=enum16{"Data", "Stats", "Specs"}."Stats") -> ("HiddenFilePath"=w2610:path)  [unwired: 13 in]
        n1403 = call "Full Table Handler.vi"("table.Data"=w2618, "table.Stats"=w2614) -> ()  [unwired: 14 in]
        n1404 = Index Array(array=w2603, index=w2608) -> (element=w2607:cluster{"FilePath":path, "Save?":bool})
        n1405 = Bundle By Name(cluster=w2607, "Save?"=TRUE) -> (w2602:cluster{"FilePath":path, "Save?":bool})
        n1406 = call-poly <vilib>:"Write To Spreadsheet File.vi"("delimiter (\\t)"="~" ("delimiter (\\t)"), "2D data"=w2615, "file path (dialog if empty)"=w2610) -> ()  [unwired: 5 in, 1 out]
        n1407 = Replace Array Subset(array=w2603, new element=w2602, index=w2608) -> (w2606:cluster{"FilePath":path, "Save?":bool}[])
        n1408 = Bundle By Name(cluster=w2605, "Created/ModFiles"=w2606) -> (w2604:T15)
      }
      frame "Save Data" {
        w2626 = cluster{u32, u32}[] [{1985280, 1985280}, {6618880, 6618880}, {1985280, 1985280}, {6618880, 6618880}]  # Original Colors
        n1409 = Unbundle By Name(w2622) -> ("CurrentDataFile"=w2624:path, "table.Data"=w2625:string[][], "ValidFile?"=w2623:bool, "Created/ModFiles"=w2621:cluster{"FilePath":path, "Save?":bool}[])
        n1410 = case shown="True" w2623 {
          tunnel: w2625 -> [_ w2644]
          tunnel: w2624 -> [_ w2639]
          tunnel: w2622 -> [w2628 w2636]
          tunnel: w2621 -> [_ w2634]
          tunnel: [w2628 w2629] -> w2620
          frame False {
          }
          frame True {
            w2633 = 0 ("index")
            n1411 = Array Subset(array=w2644, index (col)=0 ("index"), length (col)=13 ("length")) -> (w2641:string[][])  [unwired: 2 in]
            n1412 = Index Array(array=w2634, index=w2633) -> (element=w2631:cluster{"FilePath":path, "Save?":bool})
            n1413 = Bundle By Name(cluster=w2631, "Save?"=TRUE) -> (w2632:cluster{"FilePath":path, "Save?":bool})
            n1414 = call "Filepath 2 Hidden Files.vi"("DataFilePath"=w2639, "Enum"=enum16{"Data", "Stats", "Specs"}."Data") -> ("HiddenFilePath"=w2638:path)  [unwired: 13 in]
            n1415 = Replace Array Subset(array=w2634, new element=w2632, index=w2633) -> (w2630:cluster{"FilePath":path, "Save?":bool}[])
            n1416 = call-poly <vilib>:"Write To Spreadsheet File.vi"("delimiter (\\t)"="~" ("delimiter (\\t)"), "2D data"=w2641, "file path (dialog if empty)"=w2638) -> ()  [unwired: 5 in, 1 out]
            n1417 = Bundle By Name(cluster=w2636, "Created/ModFiles"=w2630) -> (w2629:T15)
          }
        }
        n1418 = property on="Stabilized?" class="Bool (strict)"("Colors [4]"=w2626) -> ()  [unwired: 2 in, 2 out]
      }
      frame "Thaw Screen" {
        n1419 = control-ref of="This VI"() -> (w2649:refnum<vi>)
        n1420 = property class="VI"(reference=w2649) -> ("Panel"=w2648:refnum<vi>)  [unwired: 1 in, 2 out]
        n1421 = property class="Pnl"(reference=w2648, "DeferPanUpdts"=FALSE ("Defer Panel Updates")) -> ()  [unwired: 1 in, 2 out]
      }
      frame "Check Test" {
        n1422 = Unbundle By Name(w2663) -> ("StepIndex"=w2660:i32, "Parameters"=w2655:string[][], "Untested SNs"=w2656:string[])
        n1423 = Array Size(array=w2655) -> (size(s)=w2659:i32[])
        n1424 = local read "TestType"() -> (w2654:enum32{"Flow", "Test", "Hot\nFuel"})
        n1425 = Index Array(array=w2659, index=1) -> (element=w2657:i32)
        n1426 = Equal?(x=w2654, y=enum32{"Flow", "Test", "Hot\nFuel"}."Hot\nFuel") -> (x = y?=w2652:bool)
        n1427 = Less?(x=w2660, y=w2657) -> (x < y?=w2651:bool)
        n1428 = Or(x=w2652, y=w2651) -> (x .or. y?=w2650:bool)
        n1429 = case shown="False" w2650 {
          tunnel: w2662 -> [w2672 w2678]
          tunnel: [w2673 w2677] -> w2661
          tunnel: w2656 -> [w2668 _]
          frame False {
            n1430 = Empty Array?(array=w2668) -> (empty?=w2664:bool)
            n1431 = Select(t=enum32{"Manual", "Test"}."Manual" ("Tab.Buttons"), s=w2664, f=enum32{"Manual", "Test"}."Test" ("Tab.Buttons")) -> (s? t:f=w2665:enum32{"Manual", "Test"})
            n1432 = Select(t=string[] ["Stop Test"], s=w2664, f=string[] ["Stop Manual", "Next Part"]) -> (s? t:f=w2669:string[])
            n1433 = local write "Tab.Buttons"(w2665) -> ()
            n1434 = Insert Into Array(array=w2672, index=0, new element=w2669) -> (w2673:string[])
          }
          frame True {
            n1435 = Insert Into Array(array=w2678, index=0, new element=string[] ["Next Step"]) -> (w2677:string[])
          }
        }
      }
      frame "Delete Data Row", "Delete Stat Row" {
        # "Can use the data index even if the delete came from stats since they always correlate to each other"
        n1436 = Unbundle By Name(w2699) -> ("table.Data"=w2698:string[][], "CurrentDataFile"=w2684:path, "ValidFile?"=w2693:bool, "StatBundle"=w2690:T7, "Controller.Command Step"=w2686:dbl, "Created/ModFiles"=w2685:cluster{"FilePath":path, "Save?":bool}[])
        n1437 = property on="table.Data" class="Tbl (strict)"() -> ("Selection Start"=w2700:T19)  [unwired: 2 in, 2 out]
        n1438 = property on="table.Stats" class="Tbl (strict)"() -> ("Selection Start"=w2692:T19)  [unwired: 2 in, 2 out]
        n1439 = Unbundle(w2700) -> ("Row"=w2681:i32)  [unwired: 1 out]
        n1440 = Unbundle(w2692) -> ("Row"=w2682:i32)  [unwired: 1 out]
        n1441 = Delete From Array(array=w2698, index (row)=w2681) -> (deleted portion=w2687:string[], array with subset deleted=w2679:string[][])  [unwired: 2 in]
        n1442 = call "Delete Stat Row.vi"("StatBundle In"=w2690, "DeletedRow"=w2687, "CMD Step"=w2686) -> ("StatBundle Out"=w2688:T7)  [unwired: 12 in]
        n1443 = call "Stat Bundles to Table.vi"("StatBundle"=w2688) -> ("table.Stats"=w2680:string[][])  [unwired: 14 in]
        n1444 = call "Handle Tables after row deletion.vi"("table.Data"=w2679, "table.Stats"=w2680, "DataRowIndex"=w2681, "StatRowIndex"=w2682, "StateCalled"=w2683) -> ()  [unwired: 11 in]
        n1445 = local write "table.Data"(w2679) -> ()
        n1446 = local write "table.Stats"(w2680) -> ()
        n1447 = Bundle By Name(cluster=w2699, "table.Data"=w2679, "table.Stats"=w2680, "StatBundle"=w2688) -> (w2689:T15)
        n1448 = case shown="True" w2693 {
          tunnel: w2680 -> [_ w2718]
          tunnel: w2679 -> [_ w2711]
          tunnel: w2685 -> [_ w2705]
          tunnel: w2689 -> [w2701 w2704]
          tunnel: [w2701 w2703] -> w2694
          tunnel: w2684 -> [_ w2702]
          frame False {
          }
          frame True {
            w2709 = 0 ("index")
            n1449 = Index Array(array=w2705, index=w2709) -> (element=w2707:cluster{"FilePath":path, "Save?":bool})
            n1450 = Bundle By Name(cluster=w2707, "Save?"=TRUE) -> (w2708:cluster{"FilePath":path, "Save?":bool})
            n1451 = Array Subset(array=w2711, index (col)=0 ("index"), length (col)=13 ("length")) -> (w2722:string[][])  [unwired: 2 in]
            n1452 = Array Subset(array=w2718, index (col)=0 ("index"), length (col)=13 ("length")) -> (w2721:string[][])  [unwired: 2 in]
            n1453 = Replace Array Subset(array=w2705, new element=w2708, index=w2709) -> (w2706:cluster{"FilePath":path, "Save?":bool}[])
            n1454 = call "Filepath 2 Hidden Files.vi"("DataFilePath"=w2702, "Enum"=enum16{"Data", "Stats", "Specs"}."Data") -> ("HiddenFilePath"=w2715:path)  [unwired: 13 in]
            n1455 = call "Filepath 2 Hidden Files.vi"("DataFilePath"=w2702, "Enum"=enum16{"Data", "Stats", "Specs"}."Stats") -> ("HiddenFilePath"=w2714:path)  [unwired: 13 in]
            n1456 = Bundle By Name(cluster=w2704, "Created/ModFiles"=w2706) -> (w2703:T15)
            n1457 = call-poly <vilib>:"Write To Spreadsheet File.vi"("delimiter (\\t)"="~" ("delimiter (\\t)"), "2D data"=w2722, "file path (dialog if empty)"=w2715) -> ()  [unwired: 5 in, 1 out]
            n1458 = call-poly <vilib>:"Write To Spreadsheet File.vi"("delimiter (\\t)"="~" ("delimiter (\\t)"), "2D data"=w2721, "file path (dialog if empty)"=w2714) -> ()  [unwired: 5 in, 1 out]
          }
        }
        n1459 = Insert Into Array(array=w2691, index=0, new element=string[] ["Evaluate SNs"]) -> (w2697:string[])
      }
      frame "Populate Steps Enum" {
        n1460 = Unbundle By Name(w2735) -> ("Parameters"=w2733:string[][])
        n1461 = Delete From Array(array=w2733, length=2, index (row)=0) -> (array with subset deleted=w2730:string[][])  [unwired: 1 in, 1 out]
        n1462 = Transpose 2D Array(2D array=w2730) -> (transposed array=w2729:string[][])
        n1463 = for {
          tunnel: w2729 -> [w2746] mode=indexing
          tunnel: [w2741] -> w2728 mode=indexing
          i -> [w2740]
          n1464 = Increment(x=w2740) -> (x+1=w2739:i32)
          n1465 = Number To Decimal String(number=w2739) -> (decimal integer string=w2738:string)  [unwired: 1 in]
          n1466 = Concatenate Strings(w2738, ")   ") -> (w2736:string)
          n1467 = for {
            tunnel: w2746 -> [w2747] mode=indexing
            shift-right: [w2748] -> w2745
            shift-left: w2736 -> [w2749]
            i -> [w2751]
            n1468 = Empty String/Path?(string/path=w2747) -> (empty?=w2750:bool)
            n1469 = case shown="False" w2750 {
              tunnel: w2751 -> [_ w2758]
              tunnel: w2749 -> [w2752 w2757]
              tunnel: [w2752 w2754] -> w2748
              tunnel: w2747 -> [_ w2756]
              frame True {
              }
              frame False {
                n1470 = case shown="1" w2758 {
                  tunnel: ["V=" "P=" "F=" "S=" "C="] -> w2755
                  frame 0, Default {
                  }
                  frame 1 {
                  }
                  frame 2 {
                  }
                  frame 3 {
                  }
                  frame 4 {
                  }
                }
                n1471 = Concatenate Strings(w2757, w2755, w2756, ", ") -> (w2754:string)
              }
            }
          }
          n1472 = String Length(string=w2745) -> (length=w2744:i32)
          n1473 = Subtract(x=w2744, y=2) -> (x-y=w2742:i32)
          n1474 = String Subset(string=w2745, length (rest)=w2742) -> (substring=w2741:string)  [unwired: 1 in]
        }
        n1475 = Insert Into Array(array=w2728, index=0, new element="Manual" ("new element/subarray")) -> (w2727:string[])
        n1476 = property on="Steps" class="Ring (strict)"("Strings []"=w2727) -> ()  [unwired: 2 in, 2 out]
      }
      frame "Request Cal Date" {
        w2765 = "ReqCalDate" ("Flattened Data")
        n1477 = Bundle(cluster=T22 {"Command"="", "FlattenedData"=""}, "Command"=w2765, "FlattenedData"=w2765) -> (w2766:T22)
        n1478 = Flatten To String(anything=w2766) -> (data string=w2764:string)  [unwired: 3 in, 2 out]
        n1479 = call "PC Send Event.vi"("PC Send Command"=PCsend_RTrecv_CMD."ReqCalDate", "Mode"=Event_Mode."Set", "Flattened Data"=w2764) -> ()  [unwired: 11 in, 2 out]
      }
      frame "Save Config" {
        n1480 = Unbundle By Name(w2785) -> ("CurrentDataFile"=w2773:path, "StandConfigCluster"=w2789:T14, "IP Address"=w2790:string, "DefaultDataPath"=w2772:path, "Gauge Number"=w2779:string, "ExpectedFPGA"=w2777:i32)
        n1481 = call <vilib>:"Application Directory.vi"() -> ("Application Directory"=w2778:path)
        n1482 = Build Path(base path=w2778, name or relative path="Files\\Config.ini") -> (appended path=w2787:path)
        n1483 = Bundle("CurrentDataFile"=w2773, "StandConfigCluster"=w2789, "IP Address"=w2790, "DefaultDataPath"=w2772, "Gauge Number"=w2779, "ExpectedFPGA"=w2777) -> (w2783:T24)  [unwired: 1 in]
        n1484 = call "Read Write Config.vi"("Config File"=w2787, "Read?"=FALSE, "Cluster In"=w2783) -> ("Cluster Out"=w2786:T24)  [unwired: 11 in, 1 out]
        n1485 = Unbundle(w2786) -> ("CurrentDataFile"=w2774:path, "StandConfigCluster"=w2781:T14, "IP Address"=w2782:string, "DefaultDataPath"=w2775:path, "Gauge Number"=w2780:string, "ExpectedFPGA"=w2776:i32)
        n1486 = Bundle By Name(cluster=w2785, "CurrentDataFile"=w2774, "StandConfigCluster"=w2781, "IP Address"=w2782, "DefaultDataPath"=w2775, "Gauge Number"=w2780, "ExpectedFPGA"=w2776) -> (w2784:T15)
      }
      frame "RIO Connection" {
        n1487 = while {
          tunnel: w2796 -> [w2800]
          tunnel: [w2799] -> w2795
          shift-right: [w2797] -> w2793
          shift-left: w2794 -> [w2798]
          stop <- w2801 stop-if-true
          n1488 = event shown="[1] \"IP Address 2\": Value Change" {
            selector: _ -> [_ _ _ _]
            dyn-events: _ -> [_ _ _ _]
            timeout: 50 -> [_ _ _ _]
            tunnel: [FALSE TRUE ("Discard?") TRUE TRUE ("Discard?")] -> w2801
            tunnel: [w2804 w2807 w2836 string[] ["Exit Preparation"]] -> w2797
            tunnel: w2800 -> [w2805 w2812 w2840 w2844]
            tunnel: [w2805 w2811 w2840 w2844] -> w2799
            tunnel: w2798 -> [w2804 w2810 w2839 _]
            event Timeout {
              n1489 = event-data() -> ()  [unwired: 1 in, 1 out]
              n1490 = local write "Screen"(T1."RIO Connection" ("Screen")) -> ()
            }
            event "IP Address 2": Value Change {
              n1491 = event-data() -> ("NewVal"=w2813:string)  [unwired: 1 in]
              n1492 = String Length(string=w2813) -> (length=w2823:i32)
              n1493 = Search and Replace String(replace all?=TRUE ("replace all? (F)"), input string=w2813, search string=".") -> (number of replacements=w2817:i32)  [unwired: 5 in, 3 out]
              n1494 = In Range and Coerce(upper limit=15, x=w2823, lower limit=7) -> (In Range?=w2818:bool)  [unwired: 1 out]
              n1495 = Equal?(x=w2817, y=3) -> (x = y?=w2815:bool)
              n1496 = And(x=w2815, y=w2818) -> (x .and. y?=w2814:bool)
              n1497 = case shown="True" w2814 {
                tunnel: w2813 -> [_ w2827]
                frame False {
                }
                frame True {
                  n1498 = Current VI's Path() -> (path=w2831:path)
                  n1499 = Strip Path(path=w2831) -> (stripped path=w2830:path)  [unwired: 1 out]
                  n1500 = Build Path(base path=w2830, name or relative path="IP.ini") -> (appended path=w2828:path)
                  n1501 = call <vilib>:"Open Config Data.vi"("configuration file path"=w2828) -> ("error out"=w2834:errorcluster, "refnum"=w2832:T27)  [unwired: 8 in, 1 out]
                  n1502 = call-poly <vilib>:"Write Key.vi"("section"="IP", "error in (no error)"=w2834, "value"=w2827, "key"="IP Address", "refnum"=w2832) -> ("error out"=w2825:errorcluster, "refnum out"=w2826:T27)  [unwired: 4 in, 1 out]
                  n1503 = local write "IP Address"(w2827) -> ()
                  n1504 = local write "IP Address 2"(w2827) -> ()
                  n1505 = call <vilib>:"Close Config Data.vi"("error in (no error)"=w2825, "refnum"=w2826) -> ()  [unwired: 8 in, 2 out]
                }
              }
              n1506 = Bundle By Name(cluster=w2812, "IP Address"=w2813) -> (w2811:T15)
              n1507 = Insert Into Array(array=w2810, index=0, new element=string[] ["Save Config", "RIO Connection"]) -> (w2807:string[])
            }
            event "pb.RetryRIO": Value Change {
              n1508 = event-data() -> ()  [unwired: 1 in, 1 out]
              n1509 = local read "IP Address 2"() -> (w2842:string)
              n1510 = property on="pb.RetryRIO" class="Bool (strict)"("BoolText.Text"="Connecting" ("Boolean Text.Text")) -> ()  [unwired: 2 in, 2 out]
              n1511 = local write "IP Address"(w2842) -> ()
              n1512 = Insert Into Array(array=w2839, index=0, new element=string[] ["Set Cursor Busy", "Request Connection", "Connect to RIO"]) -> (w2836:string[])
            }
            event "Panel Close?": Value Change {
              n1513 = event-data() -> ()  [unwired: 1 in, 1 out]
            }
          }
        }
      }
      frame "Request Connection" {
        w2858 = T33 {"ConnectAttemptLimit(5)"=5, "IP Address"="", "Send Port"=0, "Recv Port"=0}  # ConnSettingCluster
        # "The calibration software creates ports based on last section of RIO IP address plus 5000\nsince our section start at 100 these ports are fine for now... should possibly do the same thing with a different base"
        n1514 = local read "IP Address"() -> (w2849:string)
        n1515 = Bundle(cluster=w2858, "ConnectAttemptLimit(5)"=u32 5, "IP Address"=w2849, "Send Port"=u16 5555, "Recv Port"=u16 5050) -> (w2857:T33)
        n1516 = Flatten To String(anything=w2857) -> (data string=w2856:string, error out=w2848:errorcluster)  [unwired: 3 in, 1 out]
        n1517 = call "PC Send Event.vi"("PC Send Command"=PCsend_RTrecv_CMD."ConnSettings", "Mode"=Event_Mode."Set", "Flattened Data"=w2856, "Error In"=w2848) -> ("Error Out"=w2850:errorcluster)  [unwired: 10 in, 1 out]
        n1518 = call "PC Send Event.vi"("PC Send Command"=PCsend_RTrecv_CMD."Connect", "Mode"=Event_Mode."Set", "Error In"=w2850) -> ("Error Out"=w2847:errorcluster)  [unwired: 11 in, 1 out]
        n1519 = call <vilib>:"Clear Errors.vi"("error in (no error)"=w2847) -> ()  [unwired: 6 in, 1 out]
      }
      frame "Set Cursor Busy" {
        n1520 = call <vilib>:"Set Busy.vi"() -> ()  [unwired: 10 in, 2 out]
      }
      frame "Unset Cursor Busy" {
        n1521 = call <vilib>:"Unset Busy.vi"() -> ()  [unwired: 11 in, 1 out]
      }
      frame "Component Files" {
        # "Before allowing any input that could result in a file this will check for any component files and if a whole set\nexists then I will assume that the previous run crashed so any components will be assembled into a final file"
        n1522 = Unbundle By Name(w2874) -> ("Controller List"=w2868:T9, "DefaultDataPath"=w2873:path, "TemplatePath"=w2869:path, "Controller.Command Step"=w2867:dbl)
        n1523 = List Folder(path=w2873) -> (path out=w2872:path, filenames=w2871:string[], error out=w2870:errorcluster)  [unwired: 3 in, 1 out]
        n1524 = case shown="No Error" w2870 {
          tunnel: w2872 -> [w2885 _]
          tunnel: w2871 -> [w2884 _]
          tunnel: w2869 -> [w2878 _]
          tunnel: w2868 -> [w2877 _]
          tunnel: w2867 -> [w2876 _]
          frame No Error {
            n1525 = for {
              tunnel: w2885 -> [w2923]
              tunnel: w2884 -> [w2917] mode=indexing
              tunnel: [w2920] -> w2883 mode=indexing if=w2919
              w2922 = 5 ("length (rest)")
              n1526 = String Subset(string=w2917, length (rest)=w2922) -> (substring=w2925:string)  [unwired: 1 in]
              n1527 = String Subset(string=w2917, offset (0)=w2922) -> (substring=w2916:string)  [unwired: 1 in]
              n1528 = for {
                tunnel: w2925 -> [w2928]
                tunnel: string[] ["Data_", "Spec_", "Stat_"] -> [w2929] mode=indexing
                tunnel: [w2927] -> w2919
                tunnel: [w2926] -> w2921
                i -> [w2926]
                stop <- w2927 stop-if-true
                n1529 = Equal?(x=w2929, y=w2928) -> (x = y?=w2927:bool)
              }
              n1530 = Build Path(base path=w2923, name or relative path=w2916) -> (appended path=w2918:path)
              n1531 = Bundle(w2916, w2921, "appended path"=w2918) -> (w2920:cluster{string, i32, "appended path":path})  [unwired: 1 in]
            }
            n1532 = Array Size(array=w2883) -> (size(s)=w2881:i32)
            n1533 = Sort 1D Array(array=w2883) -> (sorted array=w2882:cluster{string, i32, "appended path":path}[])
            n1534 = Subtract(x=w2881, y=2) -> (x-y=w2879:i32)
            n1535 = for {
              N: w2879 -> [_]
              tunnel: w2882 -> [w2904]
              tunnel: w2878 -> [w2888]
              tunnel: w2877 -> [w2887]
              tunnel: w2876 -> [w2886]
              i -> [w2903]
              n1536 = Array Subset(array=w2904, index=w2903, length=3) -> (w2901:cluster{string, i32, "appended path":path}[])
              n1537 = for {
                tunnel: w2901 -> [w2915] mode=indexing
                tunnel: [w2914] -> w2900 mode=indexing
                tunnel: [w2913] -> w2899 mode=indexing
                tunnel: [w2912] -> w2889
                n1538 = Unbundle(w2915) -> (w2913:string, w2914:i32, "appended path"=w2912:path)
              }
              n1539 = Add Array Elements(numeric array=w2900) -> (sum=w2895:i32)
              n1540 = Index Array(array=w2899) -> (element #1=w2897:string, element #2=w2898:string, element #3=w2896:string)  [unwired: 3 in]
              n1541 = Equal?(x=w2897, y=w2898) -> (x = y?=w2893:bool)
              n1542 = Equal?(x=w2898, y=w2896) -> (x = y?=w2892:bool)
              n1543 = Equal?(x=w2895, y=3) -> (x = y?=w2891:bool)
              n1544 = Compound Arithmetic op=AND(w2893, w2892, w2891) -> (w2890:bool)
              n1545 = case shown="True" w2890 {
                tunnel: w2889 -> [_ w2909]
                tunnel: w2888 -> [_ w2910]
                tunnel: w2887 -> [_ w2906]
                tunnel: w2886 -> [_ w2905]
                frame False {
                }
                frame True {
                  n1546 = Bundle("appended path"=w2909, TRUE) -> (w2907:cluster{"appended path":path, bool})  [unwired: 1 in]
                  n1547 = Build Array(w2907) -> (w2911:cluster{"appended path":path, bool}[])
                  n1548 = call "Merge Files.vi"("Controller List"=w2906, "TemplatePath"=w2910, "CMD Step"=w2905, "Created/ModFiles"=w2911) -> ()  [unwired: 8 in]
                }
              }
            }
          }
          frame Error {
          }
        }
      }
      frame "Exit Preparation" {
        w2933 = 0.0 ("SP1")
        w2941 = "\u0000\u0000\u0000\bPSenable\u0000\u0000\u0000\u0001\u0000"  # PS Disable
        n1549 = Unbundle By Name(w2944) -> ("Controller.Stop Command"=w2932:dbl, "CommandCluster"=w2930:T6, "Controller List"=w2939:T9, "Created/ModFiles"=w2940:cluster{"FilePath":path, "Save?":bool}[], "Controller.Command Step"=w2938:dbl, "TemplatePath"=w2937:path)
        n1550 = Bundle(cluster=w2930, "Para1"=0, "SP1"=w2933, "Para2"=1, "SP2"=w2933, "Para3"=4, "SP3"=w2932) -> (w2931:T6)
        n1551 = Bundle By Name(cluster=w2944, "RIOTries"=0, "CommandCluster"=w2931) -> (w2946:T15)
        n1552 = call "PC Send Event.vi"("PC Send Command"=PCsend_RTrecv_CMD."PSenable", "Mode"=Event_Mode."Set", "Flattened Data"=w2941) -> ()  [unwired: 11 in, 2 out]
        n1553 = Insert Into Array(array=w2950, index=0, new element=string[] ["Write Command", "EXIT"]) -> (w2948:string[])
        n1554 = call "Merge Files.vi"("Controller List"=w2939, "TemplatePath"=w2937, "CMD Step"=w2938, "Created/ModFiles"=w2940) -> ()  [unwired: 8 in]
      }
      frame "EXIT" {
        n1555 = property class="App"() -> ("App.Kind"=w2953:T20)  [unwired: 2 in, 2 out]
        n1556 = case shown="Default" w2953 {
          frame Default {
            n1557 = control-ref of="This VI"() -> (w2957:refnum<vi>)
            n1558 = invoke class="VI" method="FP.Close"(reference=w2957) -> ()  [unwired: 2 in, 3 out]
          }
          frame "Development System" {
          }
        }
        n1559 = call "PC Send Event.vi"("PC Send Command"=PCsend_RTrecv_CMD."Stop", "Mode"=Event_Mode."Set") -> ()  [unwired: 12 in, 2 out]
      }
      frame "Spare Terminals" {
        # "Could have a mouse down event\ncause a load file event"
      }
    }
  }
  n1560 = call "PC Engine.vi"("Error In"=w8) -> ("Error Out"=→"Error Out":errorcluster, "InvalidResponses"=→"InvalidResponses":string)  [unwired: 3 in]
  n1561 = while {
    tunnel: w8 -> [_]
    stop <- w2960 stop-if-true
    n1562 = event shown="[0] Timeout" {
      selector: _ -> [_ _]
      dyn-events: _ -> [_ _]
      timeout: 100 -> [_ _]
      tunnel: [FALSE w2963] -> w2960
      event Timeout {
        n1563 = event-data() -> ()  [unwired: 1 in, 1 out]
      }
      event Panel Close? {
        w2963 = TRUE ("Discard?")
        n1564 = event-data() -> ()  [unwired: 1 in, 1 out]
        n1565 = property on="Panel Close?" class="Bool (strict)"("Val(Sgnl)"=w2963) -> ()  [unwired: 2 in, 2 out]
        n1566 = event-data("Discard?"=w2963) -> ()  [unwired: 1 in, 1 out]
      }
    }
  }
  n1567 = disable-structure shown="Disabled" {
    frame Disabled {
      w2965 = T6 {"Para1"=0, "SP1"=0.0, "Para2"=0, "SP2"=0.0, "Para3"=0, "SP3"=0.0}  # CommandCluster
      w2964 = T6 {"Para1"=0, "SP1"=0.0, "Para2"=0, "SP2"=0.0, "Para3"=0, "SP3"=0.0}  # DesiredParameters
      n1568 = property on="Steps" class="Ring (strict)"() -> ("Value"=w2966:u16, "Visible"=w2968:bool)  [unwired: 2 in, 2 out]
      n1569 = Not Equal To 0?(x=w2966) -> (x != 0?=w2967:bool)
      n1570 = And(x=w2967, y=w2968) -> (x .and. y?=w2969:bool)
      n1571 = Select(t=w2964, s=w2969, f=w2965) -> ()  [unwired: 1 out]
    }
    frame Enabled {
    }
  }
